vi "MAPPA MISURE.vi"(0 "Torsiometro":refnum<vi>, 1 "DATI NM":T29, 2 "Cluster INFO":T30={"Scelta wattmetro"={"Wattmetro"=enum."No Selection"}, "SET RPM"=0.0, "SET TEMP"=0.0, "Array banchi"=[{"Nome"="Elettropompa", "Tors. scala1"=0, "Tors. scala2"=0, "rpm"=0, "TAMB"=0, "Indici Temperature"=[0, 1], "Indice freno"=1, "alimentatore trifase"=0, "alimentatore monofase"=0, "alimentatore dc arm"=0, "alimentatore dc ecc"=0, "alimentatore dc mp"=0}, {"Nome"="Sommersa", "Tors. scala1"=0, "Tors. scala2"=0, "rpm"=0, "TAMB"=1, "Indici Temperature"=[0, 1], "Indice freno"=0, "alimentatore trifase"=0, "alimentatore monofase"=0, "alimentatore dc arm"=0, "alimentatore dc ecc"=0, "alimentatore dc mp"=0}], "Array valvole linee avvio/fermata"=[], "banco selezionato"=0, "Nomi valvole prop sistema"=[], "canale-- sensore"=[], "Attriti B1"=[], "Attriti B2"=[], "Collegamento elettrico"={"ALIMENTAZIONE ELETTRICA"=enum."AC TRIFASE", "ID"=0, "#rami freddo\\eq term resmeter"=0, "#rami riscaldamento resmeter"=0, "#rami freddo\\eq term resistomat"=0, "#rami riscaldamento resistomat"=0, "CALCOLI"=enum."AC TRIFASE"}, "lingua"=0, "Costanti collaudo"={"P [bar]"=0.0, "T amb. [°C]"=0.0, "Umidità [%]"=0.0, "T acqua [°C] 2"=0.0}, "OPZIONI MISURE RES"={"MISURA A FREDDO"=enum."RESISTOMAT", "MISURA EQ. TERMICO"=enum."RESISTOMAT", "MISURA DT PROVA IN CORSO"=enum."RESISTOMAT - CON FERMATE", "MISURE PRIMA E DOPO"=enum."RESISTOMAT", "STRUMENTI PRESENTI"=enum."NESSUNO"}, "Dati targa motore"={"Vnom"=0.0, "Fnom"=0.0, "Inom"=0.0, "Cnom"=0.0, "Npoli"=0.0, "Scorta 1"=0.0, "Scorta 2"=0.0, "Scorta 3"=0.0}}, 3 "MISURE ALL":T2={"Cluster READ NI"={"AI (0-10V)"={"AI 0"=0.0, "AI 1"=0.0, "AI 2"=0.0, "AI 3"=0.0, "AI 4"=0.0, "AI 5"=0.0, "AI 6"=0.0, "AI 7"=0.0, "AI 8"=0.0, "AI 9"=0.0, "AI 10"=0.0, "AI 11"=0.0, "AI 12"=0.0, "AI 13"=0.0, "AI 14"=0.0, "AI 15"=0.0, "AI 16"=0.0, "AI 17"=0.0, "AI 18"=0.0, "AI 19"=0.0, "AI 20"=0.0, "AI 21"=0.0, "AI 22"=0.0, "AI 23"=0.0, "AI 24"=0.0, "AI 25"=0.0, "AI 26"=0.0, "AI 27"=0.0, "AI 28"=0.0, "AI 29"=0.0, "AI 30"=0.0, "AI 31"=0.0}, "StatoAO_Cdaq[0-10V]"={"AO 1"=0.0, "AO 2"=0.0, "AO 3"=0.0, "AO 4"=0.0}, "Contatori [rpm]"={"RPM 1"=0.0, "RPM 2"=0.0}, "StatoAO_Cdaq [4-20mA]"={"Cdaq_AO [0-10V] 0 for Torque"=0.0, "Cdaq_AO [0-10V] 1"=0.0, "Cdaq_AO [0-10V] 2"=0.0, "Cdaq_AO [0-10V] 3"=0.0}, "StatoDO_Cdaq"={"Scorta 0"=FALSE, "Scorta 1"=FALSE, "Scorta 2"=FALSE, "Scorta 3"=FALSE, "Scorta 4"=FALSE, "Scorta 5"=FALSE, "Scorta 6"=FALSE, "Scorta 7"=FALSE, "Scorta 8"=FALSE, "Scorta 9"=FALSE, "Scorta 10"=FALSE, "Scorta 11"=FALSE, "Scorta 12"=FALSE, "Scorta 13"=FALSE, "Scorta 14"=FALSE, "Scorta 15"=FALSE, "Scorta 16"=FALSE, "Scorta 17"=FALSE, "Scorta 18"=FALSE, "Scorta 19"=FALSE, "Scorta 20"=FALSE, "Scorta 21"=FALSE, "Scorta 22"=FALSE, "Scorta 23"=FALSE, "Scorta 24"=FALSE, "Scorta 25"=FALSE, "Scorta 26"=FALSE, "Scorta 27"=FALSE, "Scorta 28"=FALSE, "Scorta 29"=FALSE, "Scorta 30"=FALSE, "Scorta 31"=FALSE}, "DI"={"Scorta 0"=FALSE, "Scorta 1"=FALSE, "Scorta 2"=FALSE, "Scorta 3"=FALSE, "Scorta 4"=FALSE, "Scorta 5"=FALSE, "Scorta 6"=FALSE, "Scorta 7"=FALSE, "Scorta 8"=FALSE, "Scorta 9"=FALSE, "Scorta 10"=FALSE, "Scorta 11"=FALSE, "Scorta 12"=FALSE, "Scorta 13"=FALSE, "Scorta 14"=FALSE, "Scorta 15"=FALSE, "Scorta 16"=FALSE, "Scorta 17"=FALSE, "Scorta 18"=FALSE, "Scorta 19"=FALSE, "Scorta 20"=FALSE, "Scorta 21"=FALSE, "Scorta 22"=FALSE, "Scorta 23"=FALSE, "Scorta 24"=FALSE, "Scorta 25"=FALSE, "Scorta 26"=FALSE, "Scorta 27"=FALSE, "Scorta 28"=FALSE, "Scorta 29"=FALSE, "Scorta 30"=FALSE, "Scorta 31"=FALSE}, "AI (4-20mA)"={"AI 0"=0.0, "AI 1"=0.0, "AI 2"=0.0, "AI 3"=0.0, "AI 4"=0.0, "AI 5"=0.0, "AI 6"=0.0, "AI 7"=0.0, "AI 8"=0.0, "AI 9"=0.0, "AI 10"=0.0, "AI 11"=0.0, "AI 12"=0.0, "AI 13"=0.0, "AI 14"=0.0, "AI 15"=0.0}, "TC [°C]"={"tc 1"=0.0, "tc 2"=0.0, "tc 3"=0.0, "tc 4"=0.0}, "NI Read Values"={"RPM"=0.0, "Frequency"=0.0, "Mod 1"={"Torsiometro 1"=0.0, "Torsiometro 2"=0.0, "Strin Gauge 1"=0.0, "Strin Gauge 2"=0.0}, "Mod 2"={"Termocoppia 1"=0.0, "Termocoppia 2"=0.0, "Termocoppia 3"=0.0, "Termocoppia 4"=0.0}, "Mod 3"={"PT 100 1"=0.0, "PT 100 2"=0.0, "PT 100 3"=0.0, "PT 100 4"=0.0}}}, "MISURE WT"={"URMS 1"=0.0, "IRMS 1"=0.0, "P 1"=0.0, "S 1"=0.0, "Q 1"=0.0, "LAMBDA 1"=0.0, "PHI 1"=0.0, "F U 1"=0.0, "F I 1"=0.0, "NONE 1"=0.0, "URMS 2"=0.0, "IRMS 2"=0.0, "P 2"=0.0, "S 2"=0.0, "Q 2"=0.0, "LAMBDA 2"=0.0, "PHI 2"=0.0, "F U 2"=0.0, "F I 2"=0.0, "NONE 2"=0.0, "URMS 3"=0.0, "IRMS 3"=0.0, "P 3"=0.0, "S 3"=0.0, "Q 3"=0.0, "LAMBDA 3"=0.0, "PHI 3"=0.0, "F U 3"=0.0, "F I 3"=0.0, "NONE 3"=0.0, "URMS SIGMA"=0.0, "IRMS SIGMA"=0.0, "P SIGMA"=0.0, "S SIGMA"=0.0, "Q SIGMA"=0.0, "LAMBDA SIGMA"=0.0, "PHI SIGMA"=0.0, "F U SIGMA"=0.0, "F I SIGMA"=0.0, "NONE 4"=0.0}, "Resistenze Resistomat"={"Res Ch1"=0.0, "Res Ch2"=0.0, "Res Ch3"=0.0, "Tamb"=0.0}, "INTERFACCIA"={"AI"={"Portate"=[], "Pressioni"=[], "Coppie[Nm]"=[], "Valvole prop %"=[], "RPM"=[], "Livelli"=[], "Temperature"=[], "Riferimenti %"=[], "TENSIONI"=[], "CORRENTI"=[]}, "DI (logici)"={"Start da pulsantiera"=FALSE, "Stop da pulsantiera"=FALSE, "Reset da pulsantiera"=FALSE, "Sistema OK"=FALSE, "Collaudo abilitato"=FALSE, "Potenza trifase abilitata"=FALSE, "Potenza monofase abilitata"=FALSE, "Potenza DC abilitata"=FALSE, "Potenza DC ECC abilitata"=FALSE, "Start alimentazione AC"=FALSE, "Start alimentazione DC"=FALSE, "Start DC eccitazione"=FALSE, "Teleruttore WT abilitato"=FALSE, "Teleruttore Resistomat abilitato"=FALSE, "Teleruttore corto fasi"=FALSE, "Ramo 1 resistomat"=FALSE, "Ramo 2 resistomat"=FALSE, "Ramo 3 resistomat"=FALSE, "B1 Scelta linea elettrica 1"=FALSE, "B1 Scelta linea elettrica 2"=FALSE, "B1 Scelta linea elettrica 3"=FALSE, "B1 Scelta linea elettrica 4"=FALSE, "B1 Scelta linea elettrica 5"=FALSE, "B2 Scelta linea elettrica 1"=FALSE, "B2 Scelta linea elettrica 2"=FALSE, "B2 Scelta linea elettrica 3"=FALSE, "B2 Scelta linea elettrica 4"=FALSE, "B2 Scelta linea elettrica 5"=FALSE, "Rotore bloccato 1"=FALSE, "Rotore bloccato 2"=FALSE, "FRENO 1 abilitato"=FALSE, "FRENO 1 run"=FALSE, "FRENO 1 senso rotaz"=FALSE, "FRENO 1 ctrl velocità"=FALSE, "FRENO 2 abilitato"=FALSE, "FRENO 2 run"=FALSE, "FRENO 2 senso rotaz"=FALSE, "FRENO 2 ctrl velocità"=FALSE, "ALIM 1 abilitato"=FALSE, "ALIM 1 run"=FALSE, "ALIM 2 abilitato"=FALSE, "ALIM 2 run"=FALSE, "ALIM 3 abilitato"=FALSE, "ALIM 3 run"=FALSE, "FRENO 1 ctrl coppia"=FALSE, "FRENO 2 ctrl coppia"=FALSE, "FRENO 3 ctrl coppia"=FALSE, "DI (logici) aggiuntivi impianto"={"Solo freno abilitato"=FALSE, "Carico resistivo abilitato"=FALSE, "AFE+freno abilitato"=FALSE, "Protezioni chiuse"=FALSE, "Start potenza AFE"=FALSE, "AFE in marcia"=FALSE}, "Misura corrente diretta WT"=FALSE, "Misura corrente sens ext"=FALSE, "Sens ext abilitati"=FALSE}, "AO non scalati"={"FRENO1 rif vel"=0.0, "FRENO1 rif Coppia"=0.0, "FRENO2 rif vel"=0.0, "FRENO2 rif Coppia"=0.0, "ALIM1 rif V"=0.0, "ALIM1 rif F"=0.0, "ALIM2 rif V"=0.0, "ALIM2 rif F"=0.0, "ALIM3 rif V"=0.0, "ALIM3 rif F"=0.0, "Fnom keb"=0.0, "Rpm nom keb"=0.0, "Pnom keb"=0.0, "Inom keb"=0.0, "Vnom keb"=0.0, "Rpm max keb"=0.0, "Tempo rampa keb"=0.0, "Tipo Mot keb"=0.0, "FRENO  rif Coppia "=0.0, "FRENO  rif  Corrente"=0.0}, "AO scalati"={"FRENO1 rif vel"=0.0, "FRENO1 rif Coppia"=0.0, "FRENO2 rif vel"=0.0, "FRENO2 rif Coppia"=0.0, "ALIM1 rif V"=0.0, "ALIM1 rif F"=0.0, "ALIM2 rif V"=0.0, "ALIM2 rif F"=0.0, "ALIM3 rif V"=0.0, "ALIM3 rif F"=0.0, "Fnom keb"=0.0, "Rpm nom keb"=0.0, "Pnom keb"=0.0, "Inom keb"=0.0, "Vnom keb"=0.0, "Rpm max keb"=0.0, "Tempo rampa keb"=0.0, "Tipo Mot keb"=0.0, "FRENO  rif Coppia "=0.0, "FRENO  rif  Corrente"=0.0}, "DO (logici)"={"Scelta banco 1"=FALSE, "Scelta banco 2"=FALSE, "Scelta banco 3"=FALSE, "FRENO 1 abilita"=FALSE, "FRENO 1 start"=FALSE, "FRENO 1 senso rotaz"=FALSE, "FRENO 1 ctrl velocità"=FALSE, "FRENO 2 abilita"=FALSE, "FRENO 2 start"=FALSE, "FRENO 2 senso rotaz"=FALSE, "FRENO 2 ctrl velocità"=FALSE, "ALIM 1 abilita"=FALSE, "ALIM 1 start"=FALSE, "ALIM 2 abilita"=FALSE, "ALIM 2 start"=FALSE, "ALIM 3 abilita"=FALSE, "ALIM 3 start"=FALSE, "Abilita linea trifase"=FALSE, "Abilita linea monofase"=FALSE, "Abilita linea dc"=FALSE, "Abilita linea dc eccit"=FALSE, "B1 Linea elettrica 1"=FALSE, "B1 Linea elettrica 2"=FALSE, "B1 Linea elettrica 3"=FALSE, "B1 Linea elettrica 4"=FALSE, "B1 Linea elettrica 5"=FALSE, "B2 Linea elettrica 1"=FALSE, "B2 Linea elettrica 2"=FALSE, "B2 Linea elettrica 3"=FALSE, "B2 Linea elettrica 4"=FALSE, "B2 Linea elettrica 5"=FALSE, "Start potenza AC"=FALSE, "Stop pontenza AC"=FALSE, "Start potenza DC"=FALSE, "Stop potenza DC"=FALSE, "Start potenza eccitaz"=FALSE, "Stop potenza eccitaz"=FALSE, "Reset allarmi"=FALSE, "watchdog"=FALSE, "Scala torsiometro B1"=FALSE, "Controllo torsiom B1"=FALSE, "Scala torsiometro B2"=FALSE, "Controllo torsiom B2"=FALSE, "Teleruttore WT abilita"=FALSE, "Teleruttore Resistomat abilita"=FALSE, "Teleruttore corto fasi"=FALSE, "Ramo 1 resistomat"=FALSE, "Ramo 2 resistomat"=FALSE, "Ramo 3 resistomat"=FALSE, "Collaudo in corso"=FALSE, "Allarme presente"=FALSE, "Enable Res Meter"=FALSE, "Bypass Res Meter"=FALSE, "2nd canale Res Meter"=FALSE, "Scala 200/2000 res meter"=FALSE, "Taratura res meter"=FALSE, "FRENO 1 ctrl coppia"=FALSE, "FRENO 2 ctrl coppia"=FALSE, "FRENO 3 ctrl coppia"=FALSE, "Aggiuntivi impianto"={"Senso rotazione alim 1"=FALSE, "Senso rotazione alim 2"=FALSE}, "ALIM 1 stop"=FALSE, "ALIM 2 stop"=FALSE, "ALIM 3 stop"=FALSE, "FRENO 1 stop"=FALSE, "FRENO 2 stop"=FALSE, "FRENO 3 stop"=FALSE, "B1 configurazione freno B"=FALSE, "B2 configurazione freno B"=FALSE, "Abilita scrittura KEB"=FALSE, "Bench Selection (0-B1,1-B2)"=FALSE, "Select current mode"=FALSE, "Select torque mode"=FALSE, "Select speed mode"=FALSE, "Start"=FALSE, "Stop"=FALSE, "Block"=FALSE, "Enable Force mode"=FALSE, "Abilita linea 125 A"=FALSE, "Abilita linea 63 A"=FALSE, "Abilita linea 16 A"=FALSE, "Aum Tensione Variac"=FALSE, "Dim Tesnione Variac"=FALSE, "Abilita ellectro stractura"=FALSE, "Risprinito Emergence"=FALSE, "Abilita collaudo"=FALSE, "Disabilita collaudo"=FALSE, "External Alaram"=FALSE, "Enable external program"=FALSE, "Reset"=FALSE, "Abilita Ingresso Variac"=FALSE, "Abilita Ventilatore Variac"=FALSE, "Abilita Uscita Variac "=FALSE}}, "FREDDO resistomat"={"Res Ch1"=0.0, "Res Ch2"=0.0, "tAMB"=0.0, "Res Ch3"=0.0}, "STATO PLC 1"={"USCITE PLC"={"AO (real) 2"={"SCORTA 1"=0.0, "SCORTA 2"=0.0, "SCORTA 3"=0.0, "SCORTA 4"=0.0, "SCORTA 5"=0.0, "SCORTA 6"=0.0, "SCORTA 7"=0.0, "SCORTA 8"=0.0}, "statoAO_PLC out"={"Rif Lim coppia freno [%]"=nan, "Rif rpm freno [%]"=nan, "Rif coppia freno [%]"=0.0, "Rif V alimentatore [%]"=0.0, "Rif F alimentatore [%]"=0.0}, "DO (bit)"={"Scelta banco 1"=FALSE, "Set dati motore freno 2"=FALSE, "Diretto inverter"=FALSE, "Filtro LC"=FALSE, "Marcia ALIM (1s)"=FALSE, "Marcia FRENO (1s)"=FALSE, "Stop AFE (1s)"=FALSE, "Stop freno (1s)"=FALSE, "Reset allarmi"=FALSE, "Watchdog"=FALSE, "Senso rotazione"=FALSE, "Abilita collaudo (1s)"=FALSE, "Disabilita collaudo (1s)"=FALSE, "Abilitazione ALIM"=FALSE, "Abilitazione FRENO"=FALSE, "Teleruttore WT"=FALSE, "Senso rot motore prova"=FALSE, "Scorta 7"=FALSE, "Scorta 8"=FALSE, "Scorta 9"=FALSE, "Scorta 10"=FALSE, "Scorta 11"=FALSE, "Scorta 12"=FALSE, "Scorta 13"=FALSE}}, "Stato DI_PLC"={"Sistema OK"=FALSE, "Rotore bloccato"=FALSE, "Scorta 1"=FALSE, "Prova diretto inverter"=FALSE, "Prova con filtro LC"=FALSE, "Teleruttore WT abilitato"=FALSE, "Alim sinus penta abilitato"=FALSE, "Alim sinus penta in marcia"=FALSE, "Freno abilitato"=FALSE, "Freno in marcia"=FALSE, "Senso rotazione freno"=FALSE, "Potenza abilitata"=FALSE, "Scorta 3"=FALSE, "Scorta 4"=FALSE, "scorta 5"=FALSE, "scorta 6"=FALSE}, "AI plc"={"Allarmi 1"=0.0, "Allarmi 2"=0.0, "Scorta 1"=0.0, "Scorta 2"=0.0, "RPM mot prova"=0.0, "I mot prova"=0.0, "RPM freno"=0.0, "I freno"=0.0, "Scorta 3"=0.0, "Scorta 4"=0.0}}, "Res Ch2"=0.0, "Res Ch2 2"=0.0, "FREDDO res meter"={"Res Ch1"=0.0, "Res Ch2"=0.0, "tAMB"=0.0, "Res Ch3"=0.0}, "Resistenze Res Meter"={"Res Ch1"=0.0, "Res Ch2"=0.0, "Res Ch3"=0.0, "Tamb"=0.0}, "READ SINUS PENTA"={"Menù Misure motore (M000-M030)"={"Rif vel a regime (int)"=0, "Rif vel a regime (dec)"=0, "Rif vel dopo rampe (int)"=0, "Rif vel dopo rampe (dec)"=0, "RPM motore (int)"=0, "RPM motore (dec)"=0, "FREQout inverter"=0, "Rif coppia a regime(Nm)"=0, "Richiesta di coppia (Nm)"=0, "Coppia generata dal motore(Nm)"=0, "Rif coppia a regime(%)"=0, "Richiesta di coppia (%)"=0, "Coppia generata dal motore(%)"=0, "Coppia max richiesta prima delle rampe(Nm)"=0, "Coppia max richiesta dopo le rampe(Nm)"=0, "Limite di velocità prima delle rampe"=0, "Limite di velocità dopo le rampe"=0, "Coppia max richiesta prima delle rampe(%)"=0, "Coppia max richiesta dopo le rampe(%)"=0, "Rif di flusso"=0, "Corrente di uscita"=0, "Capacità termica del motore"=0, "Tensione di uscita"=0, "Potenza di uscita"=0, "Energia consumata (LSword)"=0, "Energia consumata (MSword)"=0, "Tensione bus DC"=0, "Tensione di rete"=0}, "Menù regolatore PID (M018-M024)"={"Rif PID a regime(%)"=0, "Rif pid dopo rampe(%)"=0, "Retroazione del pid(%)"=0, "Errore del pid(%)"=0, "uscita del pid(%)"=0, "Rif del pid dopo le rampe"=0, "Retroazione del pid"=0}, "Menù ingressi digitali (M031-M036)"={"Ingressi digitali ritardati"=0, "Ingressi digitali istantanei"=0, "Moresettiera comando loc"=0, "Morsett comando da seriale"=0, "Morsett comando bus di campo"=0, "Ing dig ausiliari da morsettiera"=0, "Ing dig ausiliari da seriale"=0}, "Menù riferimenti (M037-M051)"={"Rif analog est REF"=0, "Rif analog est AIN1"=0, "Rif analog est AIN2"=0, "Rif analog est XAIN4"=0, "Rif analog est XAIN5"=0, "Rif velocità da seriale(int)"=0, "Rif velocità bus di campo(int)"=0, "Rif coppia da seriale"=0, "Rif coppia bus di campo"=0, "Rif del PID da seriale"=0, "Rif del PID da bus di campo"=0, "Retroazione del PID da seriale"=0, "Retroazione del PIDda bus di campo"=0, "Rif da encoder"=0, "Rif in frequenza"=0, "Rif velocità da seriale(dec)"=0, "Rif velocità bus di campo(dec)"=0}, "Menù rampe (P009-P033)"={"Tempo di dec rampa di vel 1"=0, "Tempo di acc rampa di vel 2"=0, "Tempo di dec rampa di vel 2"=0, "Tempo di acc rampa di vel 1"=0, "Unità di mis tempi rampe vel 1/2"=0, "Tempo di acc rampa di vel 3"=0, "Tempo di dec rampa di vel 3"=0, "Tempo di acc rampa di vel 4"=0, "Tempo di dec rampa di vel 4"=0, "Unità di mis tempi rampe vel 3/4"=0, "Selettore arrottondam rampe"=0, "Tempo di arrotond iniz rampa acc"=0, "Tempo di arrotond finale rampa acc"=0, "Tempo di arrotond iniz rampa dec"=0, "Tempo di rampa di salita rif coppia"=0, "Tempo di rampa di discesa rif coppia"=0, "Unità di misura rampa coppia"=0, "Tempo rampa acc marcia jog"=0, "Tempo rampa dec marcia jog"=0, "Reset acc ai cambi pendenza"=0, "rampa di acc in fire mode"=0, "rampa di dec in fire mode"=0, "Tempo di arrotond finale rampa dec"=0}, "Menù controllo motore(C008-C128)"={"Numero motori configurati"=0, "Tipo algoritmo di controllo Mot1"=0, "Tipo rif Mot1"=0, "Tensione nominale rete"=0, "Retroaz di vel da encoder Mot1"=0, "Tipo curva V/f Mot1"=0, "Rotazione delle fasi Mot1"=0, "Freq nominale del motore Mot1"=0, "RPM nominali del motore Mot1"=0, "Potenza nominale del motore Mot1"=0, "Corrente nominale del motore Mot1"=0, "Tensione nominale del motore mot1"=0, "Potenza a vuoto del motore Mot1"=0, "Corrente a vuoto del motore Mot1"=0, "Resistenza statorica del motore Mot1"=0, "Induttanza di dispersione Mot1"=0, "Induttanza mutua motore"=0, "Costante di tempo rotorica"=0, "Costante di tempo filtro pb"=0, "Velocità minima motore"=0, "Velocità massima motore"=0}, "Menù configurazione PID"={"Selezione riferimento n.1"=0, "Selezione retroazione n.1"=0, "Modalità di fuzionamento PID"=0, "Termine derivativo calcolato su err o mis"=0, "Proporz moltiplica deriv e integrale"=0, "Azione del PID"=0}, "ID"=0.0, "Menù uscite digitali"={"MDO4 Inverter pronto"=0}, "Fcarrier"={"Fcarrier Min (Hz)"=0, "Fcarrier Max (Hz)"=0}, "stato inverter M089"=0.0, "Riferimenti"={"Rif tensione"=0, "Rif velocità"=0}, "Comunicazione"=FALSE, "Modalità stop"=0.0}, "STATO PLC 2"={"USCITE PLC"={"AO (real) 2"={"SCORTA 1"=0.0, "SCORTA 2"=0.0, "SCORTA 3"=0.0, "SCORTA 4"=0.0, "SCORTA 5"=0.0, "SCORTA 6"=0.0, "SCORTA 7"=0.0, "SCORTA 8"=0.0}, "statoAO_PLC out"={"Condensatori"=0.0, "Scorta 1"=0.0, "Scorta 2"=0.0}, "DO (bit)"={"Relè misura resistomat"=FALSE, "Misura res ramo 1"=FALSE, "Misura res ramo 2"=FALSE, "Misura res ramo 3"=FALSE, "Scelta banco 2"=FALSE, "Scala Torsiometro"=FALSE, "Ctrl torsiometro"=FALSE, "Select current mode"=FALSE, "Select Torque mode"=FALSE, "Select speed mode"=FALSE, "Watchdog"=FALSE, "Scorta"=FALSE, "Scorta 2"=FALSE, "Scorta 3"=FALSE, "Scorta 4"=FALSE, "Scorta 5"=FALSE, "Bench selection"=FALSE, "External alarm"=FALSE, "Enable external program"=FALSE, "Reset allarmi"=FALSE, "Start"=FALSE, "Stop"=FALSE, "Block"=FALSE, "Scorta 6"=FALSE}}, "Stato DI_PLC"={"Sistema ok"=FALSE, "Relè Resistomat abilitato"=FALSE, "Freno abilitato"=FALSE, "Freno in marcia"=FALSE, "scorta b"=FALSE, "scorta a"=FALSE, "scorta 1"=FALSE, "scorta 2"=FALSE, "scorta 3"=FALSE, "scorta 4"=FALSE, "Scorta 5"=FALSE, "Scorta 6"=FALSE, "Scorta 7"=FALSE, "Scorta 8"=FALSE, "Scorta 9"=FALSE, "Scorta 10"=FALSE}, "AI plc"={"Allarmi 1"=0.0, "Allarmi 2"=0.0, "TC 1"=0.0, "TC 2"=0.0, "TC 3"=0.0, "TC 4"=0.0, "TC 5"=0.0, "TC 6"=0.0, "TC 7"=0.0, "TC 8"=0.0, "PT1000 1"=0.0, "PT1000 2"=0.0, "PT1000 3"=0.0, "PT1000 4"=0.0}}, "STATO PLC 3"={"USCITE PLC"={"AO (real) 2"={"SCORTA 1"=0.0, "SCORTA 2"=0.0, "SCORTA 3"=0.0, "SCORTA 4"=0.0, "SCORTA 5"=0.0, "SCORTA 6"=0.0, "SCORTA 7"=0.0, "SCORTA 8"=0.0}, "statoAO_PLC out"={"Rif velocità alimentatore"=0.0, "Scorta"=0.0, "Tipo Motore  keb"=0.0, "I nom keb"=0.0, "RPM nom keb"=0.0, "V nom keb"=0.0, "F nom keb"=0.0, "t rampa keb"=0.0}, "DO (bit)"={"Select linea Inverter"=FALSE, "Abilita sense wattmetro"=FALSE, "Bypass filtro LC"=FALSE, "Filtro LC"=FALSE, "Bypass trasformatore"=FALSE, "Trasformatore"=FALSE, "Abilita uscite variac"=FALSE, "Abilita linea 125 A"=FALSE, "Abilita linea 63 A"=FALSE, "Abilita linea 16 A"=FALSE, "Abilita Scrittura Dati Keb"=FALSE, "Abilita alimentatore"=FALSE, "Marcia alimentatore (1s)"=FALSE, "Stop alimentatore (1s)"=FALSE, "Senso rot mot prova"=FALSE, "Watchdog"=FALSE, "Aumenta tensione variac"=FALSE, "Diminuisci tensione variac "=FALSE, "Blocco elettroserrature"=FALSE, "Ripristino emergence"=FALSE, "Abilita ingresso variac"=FALSE, "Abilita ventilatore variac"=FALSE, "Reset Allarm"=FALSE, "Scorta 1"=FALSE, "Scorta 2"=FALSE, "Scorta 3"=FALSE, "Scorta 4"=FALSE, "Scorta 5"=FALSE, "Scorta 6"=FALSE, "Scorta 7"=FALSE, "Scorta 8"=FALSE, "Scorta 9"=FALSE, "Abilita collaudo"=FALSE, "Disabilita collaudo "=FALSE, "Scorta 10"=FALSE, "Scorta 11"=FALSE, "Scorta 12"=FALSE, "Scorta 13"=FALSE, "Scorta 14"=FALSE, "Scorta 15"=FALSE}}, "Stato DI_PLC"={"Sistema OK"=FALSE, "Rotore bloccato"=FALSE, "Filtro LC"=FALSE, "Bypass Filtro LC"=FALSE, "Scelta Trasformatore"=FALSE, "Scelta Bypass trasformatore"=FALSE, "Teleruttore wt abilitato"=FALSE, "Alimentatore abilitato"=FALSE, "Alimentatore in marcia"=FALSE, "Scorta 1"=FALSE, "Scorta 2"=FALSE, "Scorta 3"=FALSE, "Potenza abilitata"=FALSE, "Alimentatore in allarme"=FALSE, "Scorta 4"=FALSE, "Conferma dati KEB"=FALSE, "Scorta 5"=FALSE, "Warning Inverter Alimentatore"=FALSE, "Variac Abilitato"=FALSE, "Linea 125 A abilitata"=FALSE, "Linea 63 A abilitata"=FALSE, "Linea 16 A abilitata"=FALSE, "Scorta 6"=FALSE, "Enable force mode"=FALSE}, "AI plc"={"Allarmi 1"=0.0, "Allarmi 2"=0.0, "RPM motore prova"=0.0, "Corrente motore prova"=0.0, "RPM freno"=0.0, "Corrente freno"=0.0, "Tipo motore keb"=0.0, "I nom keb"=0.0, "RPM nom keb"=0.0, "V nom keb"=0.0, "F nom keb"=0.0, "T rampa keb"=0.0, "scorta"=0.0, "Scorta 2"=0.0}}, "DCREG"={"Parametri di misura"={"M000"=0.0, "M001"=0.0, "M002"=0.0, "M003"=0.0, "M004"=0.0, "M005"=0.0, "M006"=0.0, "M007"=0.0, "M008"=0.0, "M009"=0.0, "M010"=0.0, "M011"=0.0, "M012"=0.0, "M013"=0.0, "M014"=0.0, "M015"=0.0, "M016"=0.0, "M017"=0.0, "M018"=0.0, "M019"=0.0, "M020"=0.0, "M021"=0.0, "M022"=0.0, "M023"=0.0, "M024"=0.0, "M025"=0.0, "M026"=0.0, "M027"=0.0, "M028"=0.0, "M029"=0.0, "M030"=0.0, "M031"=0.0}, "Parametri di programmazione"={"P000"=0.0, "P001"=0.0, "P002"=0.0, "P003"=0.0, "P004"=0.0, "P005"=0.0, "P006"=0.0, "P010"=0.0, "P011"=0.0, "P012"=0.0, "P013"=0.0, "P014"=0.0, "P015"=0.0, "P016"=0.0, "P030"=0.0, "P031"=0.0, "P032"=0.0, "P033"=0.0, "P034"=0.0, "P035"=0.0, "P036"=0.0, "P037"=0.0, "P038"=0.0, "P039"=0.0, "P040"=0.0, "P050"=0.0, "P051"=0.0, "P052"=0.0, "P053"=0.0, "P054"=0.0, "P055"=0.0, "P056"=0.0, "P057"=0.0, "P058"=0.0, "P059"=0.0, "P060"=0.0, "P061"=0.0, "P062"=0.0, "P070"=0.0, "P071"=0.0, "P073"=0.0, "P074"=0.0, "P076"=0.0, "P077"=0.0, "P079"=0.0, "P080"=0.0, "P082"=0.0, "P083"=0.0, "P084"=0.0, "P085"=0.0, "P086"=0.0, "P087"=0.0, "P088"=0.0, "P100"=0.0, "P101"=0.0, "P102"=0.0, "P103"=0.0, "P104"=0.0, "P110"=0.0, "P111"=0.0, "P120"=0.0, "P121"=0.0, "P122"=0.0, "P123"=0.0, "P124"=0.0, "P125"=0.0, "P126"=0.0, "P127"=0.0, "P128"=0.0, "P129"=0.0, "P130"=0.0, "P131"=0.0, "P132"=0.0, "P133"=0.0, "P134"=0.0, "P150"=0.0, "P151"=0.0, "P152"=0.0, "P153"=0.0, "P154"=0.0, "P155"=0.0, "P156"=0.0, "P157"=0.0, "P158"=0.0, "P170"=0.0, "P171"=0.0, "P172"=0.0, "P173"=0.0, "P174"=0.0, "P175"=0.0, "P176"=0.0, "P177"=0.0, "P178"=0.0, "P179"=0.0, "P180"=0.0, "P181"=0.0, "P182"=0.0, "P183"=0.0, "P184"=0.0, "P185"=0.0, "P186"=0.0, "P187"=0.0, "P188"=0.0, "P189"=0.0, "P190"=0.0, "P191"=0.0, "P192"=0.0, "P193"=0.0, "P194"=0.0, "P195"=0.0, "P196"=0.0, "P197"=0.0, "P198"=0.0, "P199"=0.0, "P211"=0.0, "P212"=0.0, "P213"=0.0, "P214"=0.0, "P215"=0.0, "P216"=0.0, "P217"=0.0, "P221"=0.0, "P222"=0.0, "P223"=0.0, "P224"=0.0, "P230"=0.0, "P231"=0.0, "P240"=0.0, "P250"=0.0, "P251"=0.0}, "Parametri di configurazione"={"C000"=0.0, "C001"=0.0, "C002"=0.0, "C010"=0.0, "C011"=0.0, "C012"=0.0, "C014"=0.0, "C015"=0.0, "C016"=0.0, "C017"=0.0, "C018"=0.0, "C030"=0.0, "C050"=0.0, "C051"=0.0, "C052"=0.0, "C060"=0.0, "C061"=0.0, "C062"=0.0, "C063"=0.0, "C070"=0.0, "C072"=0.0, "C074"=0.0, "C090"=0.0, "C091"=0.0, "C092"=0.0, "C093"=0.0, "C094"=0.0, "C100"=0.0, "C101"=0.0, "C102"=0.0, "C103"=0.0, "C105"=0.0, "C106"=0.0, "C107"=0.0, "C108"=0.0, "C110"=0.0, "C111"=0.0, "C112"=0.0, "C120"=0.0, "C121"=0.0, "C122"=0.0, "C130"=0.0, "C131"=0.0, "C132"=0.0, "C133"=0.0, "C134"=0.0, "C135"=0.0, "C141"=0.0, "C142"=0.0, "C143"=0.0, "C150"=0.0, "C151"=0.0, "C153"=0.0, "C154"=0.0, "C155"=0.0, "C156"=0.0, "C157"=0.0, "C158"=0.0, "C159"=0.0, "C160"=0.0, "C161"=0.0, "C162"=0.0, "C163"=0.0, "C164"=0.0, "C165"=0.0, "C170"=0.0}, "Codice allarme"=0.0, "Comunicazione"=FALSE}} {"Cluster READ NI"."AI (4-20mA)"."AI 15" format="%#_6f"; "Cluster READ NI"."AI (4-20mA)"."AI 14" format="%#_6f"; "Cluster READ NI"."AI (4-20mA)"."AI 13" format="%#_6f"; "Cluster READ NI"."AI (4-20mA)"."AI 11" format="%#_6f"; "Cluster READ NI"."AI (4-20mA)"."AI 10" format="%#_6f"; "Cluster READ NI"."AI (4-20mA)"."AI 9" format="%#_6f"; "Cluster READ NI"."AI (4-20mA)"."AI 4" format="%#_6f"; "Cluster READ NI"."AI (4-20mA)"."AI 12" format="%#_6f"; "Cluster READ NI"."AI (4-20mA)"."AI 0" format="%#_6f"; "Cluster READ NI"."AI (4-20mA)"."AI 1" format="%#_6f"; "Cluster READ NI"."AI (4-20mA)"."AI 2" format="%#_6f"; "Cluster READ NI"."AI (4-20mA)"."AI 3" format="%#_6f"; "Cluster READ NI"."AI (4-20mA)"."AI 5" format="%#_6f"; "Cluster READ NI"."AI (4-20mA)"."AI 6" format="%#_6f"; "Cluster READ NI"."AI (4-20mA)"."AI 7" format="%#_6f"; "Cluster READ NI"."AI (4-20mA)"."AI 8" format="%#_6f"; "Cluster READ NI"."AI (0-10V)"."AI 31" format="%#_6f"; "Cluster READ NI"."AI (0-10V)"."AI 30" format="%#_6f"; "Cluster READ NI"."AI (0-10V)"."AI 29" format="%#_6f"; "Cluster READ NI"."AI (0-10V)"."AI 28" format="%#_6f"; "Cluster READ NI"."AI (0-10V)"."AI 27" format="%#_6f"; "Cluster READ NI"."AI (0-10V)"."AI 26" format="%#_6f"; "Cluster READ NI"."AI (0-10V)"."AI 25" format="%#_6f"; "Cluster READ NI"."AI (0-10V)"."AI 24" format="%#_6f"; "Cluster READ NI"."AI (0-10V)"."AI 23" format="%#_6f"; "Cluster READ NI"."AI (0-10V)"."AI 22" format="%#_6f"; "Cluster READ NI"."AI (0-10V)"."AI 21" format="%#_6f"; "Cluster READ NI"."AI (0-10V)"."AI 20" format="%#_6f"; "Cluster READ NI"."AI (0-10V)"."AI 19" format="%#_6f"; "Cluster READ NI"."AI (0-10V)"."AI 18" format="%#_6f"; "Cluster READ NI"."AI (0-10V)"."AI 17" format="%#_6f"; "Cluster READ NI"."AI (0-10V)"."AI 16" format="%#_6f"; "Cluster READ NI"."AI (0-10V)"."AI 15" format="%#_6f"; "Cluster READ NI"."AI (0-10V)"."AI 14" format="%#_6f"; "Cluster READ NI"."AI (0-10V)"."AI 13" format="%#_6f"; "Cluster READ NI"."AI (0-10V)"."AI 11" format="%#_6f"; "Cluster READ NI"."AI (0-10V)"."AI 10" format="%#_6f"; "Cluster READ NI"."AI (0-10V)"."AI 9" format="%#_6f"; "Cluster READ NI"."AI (0-10V)"."AI 4" format="%#_6f"; "Cluster READ NI"."AI (0-10V)"."AI 12" format="%#_6f"; "Cluster READ NI"."AI (0-10V)"."AI 0" format="%#_6f"; "Cluster READ NI"."AI (0-10V)"."AI 1" format="%#_6f"; "Cluster READ NI"."AI (0-10V)"."AI 2" format="%#_6f"; "Cluster READ NI"."AI (0-10V)"."AI 3" format="%#_6f"; "Cluster READ NI"."AI (0-10V)"."AI 5" format="%#_6f"; "Cluster READ NI"."AI (0-10V)"."AI 6" format="%#_6f"; "Cluster READ NI"."AI (0-10V)"."AI 7" format="%#_6f"; "Cluster READ NI"."AI (0-10V)"."AI 8" format="%#_6f"}, 4 "ACQ RESISTOMAT?":bool=TRUE, 6 "SIMULAZIONE":bool) -> (14 "Cluster MISURE":T27={"MISURE NM"={"Banco"="", "Anno"="", "Numero"="", "Ntabella"="", "Misura"="", "Tipo Prova"="", "ProgressivoAcq"="", "Descrizione"="", "Data_ora"="", "t. acq [h:m:s]"="", "t. acq [min]"="", "t. acq [s]"="", "n [rpm]"="", "f [Hz]"="", "U1[V]"="", "U2 [V]"="", "U3 [V]"="", "U123_media [V]"="", "I1[A]"="", "I2[A]"="", "I3[A]"="", "I123_media [A]*I"="", "I_123_sbil [%]"="", "Ulin[V]"="", "Uc [V]"="", "Uaux [V]"="", "Ilin[A]*I"="", "Imar[A]"="", "Iaux[A]"="", "Uarm[V]"="", "Uecc[V]"="", "Iarm[A]*I"="", "Iecc[A]"="", "pf"="", "P1 [W]"="", "P1 [kW]"="", "Q [VAR]"="", "Q [kVAR]"="", "S [VA]"="", "S [kVA]"="", "P1arm[W]"="", "P1ecc[W]"="", "Parm[kW]"="", "P1ecc[kW]"="", "Cond[uF]"="", "P1_linea_6fili[W]"="", "P1_linea_6fili[kW]"="", "eta_gr_6fili [%]"="", "eta_inverter_6fili [%]"="", "pf_linea_6fili"="", "U4 [V]"="", "U5 [V]"="", "U6 [V]"="", "U456_media [V]"="", "I4 [A]"="", "I5 [A]"="", "I6 [A]"="", "I456_media [A]"="", "C [Nm]*C"="", "Cric [Nm]"="", "Cric\\Cnom"="", "Iric[A]"="", "Iric\\Inom"="", "P2_mecc [W]"="", "P2_mecc [kW]"="", "eta motore [%]"="", "Scorr[%]"="", "Tamb[°C]"="", "R1[ohm]"="", "R2[ohm]"="", "R3[ohm]"="", "Rmedia[ohm]"="", "DT_R1[°C]"="", "DT_R2[°C]"="", "DT_R3[°C]"="", "DT_media[°C]"="", "R_marcia[ohm]"="", "R_aux[ohm]"="", "DT_marcia[°C]"="", "DT_aux[°C]"="", "R_Arm[ohm]"="", "R_Ecc[ohm]"="", "DT_Arm[°C]"="", "DT_Ecc[°C]"="", "TambFreddo[°C]"="", "R1_freddo[ohm]"="", "R2_freddo[ohm]"="", "R3_freddo[ohm]"="", "Rmedia_freddo[ohm]"="", "R_Marcia_freddo[ohm]"="", "R_Aux_freddo[ohm]"="", "R_Arm_freddo[ohm]"="", "R_Ecc_freddo[ohm]"="", "TC1 [°C]"="", "TC2 [°C]"="", "TC3 [°C]"="", "TC4 [°C]"="", "TC5 [°C]"="", "TC6 [°C]"="", "TC7 [°C]"="", "TC8 [°C]"="", "PT1000_1[°C]"="", "PT1000_2[°C]"="", "PT1000_3[°C]"="", "Vdc eccitatrice[V]"="", "Idc eccitatrice[A]"="", "Vdc rotore[V]"="", "Idc rotore[A]"="", "Vac rotore[V]"="", "Iac rotore[V]"="", "V dinamo[V]"="", "Portata Q"="", "Pressione H"="", "U1'[V]"="", "U2'[V]"="", "U3'[V]"="", "I1'[A]"="", "I2'[A]"="", "I3'[A]"="", "U''R-N"="", "U''S-N"="", "U'' T-N"="", "U''R-S"="", "U''R-T"="", "U''S-T"="", "I1''[A]"="", "I2''[A]"="", "I3''[A]"="", "F''[Hz]"="", "P''[kW]"="", "CosFi''"="", "PT1000_4[°C]"="", "Scorta 3"=""}, "MISURE ALL"={"Cluster READ NI"={"AI (0-10V)"={"AI 0"=0.0, "AI 1"=0.0, "AI 2"=0.0, "AI 3"=0.0, "AI 4"=0.0, "AI 5"=0.0, "AI 6"=0.0, "AI 7"=0.0, "AI 8"=0.0, "AI 9"=0.0, "AI 10"=0.0, "AI 11"=0.0, "AI 12"=0.0, "AI 13"=0.0, "AI 14"=0.0, "AI 15"=0.0, "AI 16"=0.0, "AI 17"=0.0, "AI 18"=0.0, "AI 19"=0.0, "AI 20"=0.0, "AI 21"=0.0, "AI 22"=0.0, "AI 23"=0.0, "AI 24"=0.0, "AI 25"=0.0, "AI 26"=0.0, "AI 27"=0.0, "AI 28"=0.0, "AI 29"=0.0, "AI 30"=0.0, "AI 31"=0.0}, "StatoAO_Cdaq[0-10V]"={"AO 1"=0.0, "AO 2"=0.0, "AO 3"=0.0, "AO 4"=0.0}, "Contatori [rpm]"={"RPM 1"=0.0, "RPM 2"=0.0}, "StatoAO_Cdaq [4-20mA]"={"Cdaq_AO [0-10V] 0 for Torque"=0.0, "Cdaq_AO [0-10V] 1"=0.0, "Cdaq_AO [0-10V] 2"=0.0, "Cdaq_AO [0-10V] 3"=0.0}, "StatoDO_Cdaq"={"Scorta 0"=FALSE, "Scorta 1"=FALSE, "Scorta 2"=FALSE, "Scorta 3"=FALSE, "Scorta 4"=FALSE, "Scorta 5"=FALSE, "Scorta 6"=FALSE, "Scorta 7"=FALSE, "Scorta 8"=FALSE, "Scorta 9"=FALSE, "Scorta 10"=FALSE, "Scorta 11"=FALSE, "Scorta 12"=FALSE, "Scorta 13"=FALSE, "Scorta 14"=FALSE, "Scorta 15"=FALSE, "Scorta 16"=FALSE, "Scorta 17"=FALSE, "Scorta 18"=FALSE, "Scorta 19"=FALSE, "Scorta 20"=FALSE, "Scorta 21"=FALSE, "Scorta 22"=FALSE, "Scorta 23"=FALSE, "Scorta 24"=FALSE, "Scorta 25"=FALSE, "Scorta 26"=FALSE, "Scorta 27"=FALSE, "Scorta 28"=FALSE, "Scorta 29"=FALSE, "Scorta 30"=FALSE, "Scorta 31"=FALSE}, "DI"={"Scorta 0"=FALSE, "Scorta 1"=FALSE, "Scorta 2"=FALSE, "Scorta 3"=FALSE, "Scorta 4"=FALSE, "Scorta 5"=FALSE, "Scorta 6"=FALSE, "Scorta 7"=FALSE, "Scorta 8"=FALSE, "Scorta 9"=FALSE, "Scorta 10"=FALSE, "Scorta 11"=FALSE, "Scorta 12"=FALSE, "Scorta 13"=FALSE, "Scorta 14"=FALSE, "Scorta 15"=FALSE, "Scorta 16"=FALSE, "Scorta 17"=FALSE, "Scorta 18"=FALSE, "Scorta 19"=FALSE, "Scorta 20"=FALSE, "Scorta 21"=FALSE, "Scorta 22"=FALSE, "Scorta 23"=FALSE, "Scorta 24"=FALSE, "Scorta 25"=FALSE, "Scorta 26"=FALSE, "Scorta 27"=FALSE, "Scorta 28"=FALSE, "Scorta 29"=FALSE, "Scorta 30"=FALSE, "Scorta 31"=FALSE}, "AI (4-20mA)"={"AI 0"=0.0, "AI 1"=0.0, "AI 2"=0.0, "AI 3"=0.0, "AI 4"=0.0, "AI 5"=0.0, "AI 6"=0.0, "AI 7"=0.0, "AI 8"=0.0, "AI 9"=0.0, "AI 10"=0.0, "AI 11"=0.0, "AI 12"=0.0, "AI 13"=0.0, "AI 14"=0.0, "AI 15"=0.0}, "TC [°C]"={"tc 1"=0.0, "tc 2"=0.0, "tc 3"=0.0, "tc 4"=0.0}, "NI Read Values"={"RPM"=0.0, "Frequency"=0.0, "Mod 1"={"Torsiometro 1"=0.0, "Torsiometro 2"=0.0, "Strin Gauge 1"=0.0, "Strin Gauge 2"=0.0}, "Mod 2"={"Termocoppia 1"=0.0, "Termocoppia 2"=0.0, "Termocoppia 3"=0.0, "Termocoppia 4"=0.0}, "Mod 3"={"PT 100 1"=0.0, "PT 100 2"=0.0, "PT 100 3"=0.0, "PT 100 4"=0.0}}}, "MISURE WT"={"URMS 1"=0.0, "IRMS 1"=0.0, "P 1"=0.0, "S 1"=0.0, "Q 1"=0.0, "LAMBDA 1"=0.0, "PHI 1"=0.0, "F U 1"=0.0, "F I 1"=0.0, "NONE 1"=0.0, "URMS 2"=0.0, "IRMS 2"=0.0, "P 2"=0.0, "S 2"=0.0, "Q 2"=0.0, "LAMBDA 2"=0.0, "PHI 2"=0.0, "F U 2"=0.0, "F I 2"=0.0, "NONE 2"=0.0, "URMS 3"=0.0, "IRMS 3"=0.0, "P 3"=0.0, "S 3"=0.0, "Q 3"=0.0, "LAMBDA 3"=0.0, "PHI 3"=0.0, "F U 3"=0.0, "F I 3"=0.0, "NONE 3"=0.0, "URMS SIGMA"=0.0, "IRMS SIGMA"=0.0, "P SIGMA"=0.0, "S SIGMA"=0.0, "Q SIGMA"=0.0, "LAMBDA SIGMA"=0.0, "PHI SIGMA"=0.0, "F U SIGMA"=0.0, "F I SIGMA"=0.0, "NONE 4"=0.0}, "Resistenze Resistomat"={"Res Ch1"=0.0, "Res Ch2"=0.0, "Res Ch3"=0.0, "Tamb"=0.0}, "INTERFACCIA"={"AI"={"Portate"=[], "Pressioni"=[], "Coppie[Nm]"=[], "Valvole prop %"=[], "RPM"=[], "Livelli"=[], "Temperature"=[], "Riferimenti %"=[], "TENSIONI"=[], "CORRENTI"=[]}, "DI (logici)"={"Start da pulsantiera"=FALSE, "Stop da pulsantiera"=FALSE, "Reset da pulsantiera"=FALSE, "Sistema OK"=FALSE, "Collaudo abilitato"=FALSE, "Potenza trifase abilitata"=FALSE, "Potenza monofase abilitata"=FALSE, "Potenza DC abilitata"=FALSE, "Potenza DC ECC abilitata"=FALSE, "Start alimentazione AC"=FALSE, "Start alimentazione DC"=FALSE, "Start DC eccitazione"=FALSE, "Teleruttore WT abilitato"=FALSE, "Teleruttore Resistomat abilitato"=FALSE, "Teleruttore corto fasi"=FALSE, "Ramo 1 resistomat"=FALSE, "Ramo 2 resistomat"=FALSE, "Ramo 3 resistomat"=FALSE, "B1 Scelta linea elettrica 1"=FALSE, "B1 Scelta linea elettrica 2"=FALSE, "B1 Scelta linea elettrica 3"=FALSE, "B1 Scelta linea elettrica 4"=FALSE, "B1 Scelta linea elettrica 5"=FALSE, "B2 Scelta linea elettrica 1"=FALSE, "B2 Scelta linea elettrica 2"=FALSE, "B2 Scelta linea elettrica 3"=FALSE, "B2 Scelta linea elettrica 4"=FALSE, "B2 Scelta linea elettrica 5"=FALSE, "Rotore bloccato 1"=FALSE, "Rotore bloccato 2"=FALSE, "FRENO 1 abilitato"=FALSE, "FRENO 1 run"=FALSE, "FRENO 1 senso rotaz"=FALSE, "FRENO 1 ctrl velocità"=FALSE, "FRENO 2 abilitato"=FALSE, "FRENO 2 run"=FALSE, "FRENO 2 senso rotaz"=FALSE, "FRENO 2 ctrl velocità"=FALSE, "ALIM 1 abilitato"=FALSE, "ALIM 1 run"=FALSE, "ALIM 2 abilitato"=FALSE, "ALIM 2 run"=FALSE, "ALIM 3 abilitato"=FALSE, "ALIM 3 run"=FALSE, "FRENO 1 ctrl coppia"=FALSE, "FRENO 2 ctrl coppia"=FALSE, "FRENO 3 ctrl coppia"=FALSE, "DI (logici) aggiuntivi impianto"={"Solo freno abilitato"=FALSE, "Carico resistivo abilitato"=FALSE, "AFE+freno abilitato"=FALSE, "Protezioni chiuse"=FALSE, "Start potenza AFE"=FALSE, "AFE in marcia"=FALSE}, "Misura corrente diretta WT"=FALSE, "Misura corrente sens ext"=FALSE, "Sens ext abilitati"=FALSE}, "AO non scalati"={"FRENO1 rif vel"=0.0, "FRENO1 rif Coppia"=0.0, "FRENO2 rif vel"=0.0, "FRENO2 rif Coppia"=0.0, "ALIM1 rif V"=0.0, "ALIM1 rif F"=0.0, "ALIM2 rif V"=0.0, "ALIM2 rif F"=0.0, "ALIM3 rif V"=0.0, "ALIM3 rif F"=0.0, "Fnom keb"=0.0, "Rpm nom keb"=0.0, "Pnom keb"=0.0, "Inom keb"=0.0, "Vnom keb"=0.0, "Rpm max keb"=0.0, "Tempo rampa keb"=0.0, "Tipo Mot keb"=0.0, "FRENO  rif Coppia "=0.0, "FRENO  rif  Corrente"=0.0}, "AO scalati"={"FRENO1 rif vel"=0.0, "FRENO1 rif Coppia"=0.0, "FRENO2 rif vel"=0.0, "FRENO2 rif Coppia"=0.0, "ALIM1 rif V"=0.0, "ALIM1 rif F"=0.0, "ALIM2 rif V"=0.0, "ALIM2 rif F"=0.0, "ALIM3 rif V"=0.0, "ALIM3 rif F"=0.0, "Fnom keb"=0.0, "Rpm nom keb"=0.0, "Pnom keb"=0.0, "Inom keb"=0.0, "Vnom keb"=0.0, "Rpm max keb"=0.0, "Tempo rampa keb"=0.0, "Tipo Mot keb"=0.0, "FRENO  rif Coppia "=0.0, "FRENO  rif  Corrente"=0.0}, "DO (logici)"={"Scelta banco 1"=FALSE, "Scelta banco 2"=FALSE, "Scelta banco 3"=FALSE, "FRENO 1 abilita"=FALSE, "FRENO 1 start"=FALSE, "FRENO 1 senso rotaz"=FALSE, "FRENO 1 ctrl velocità"=FALSE, "FRENO 2 abilita"=FALSE, "FRENO 2 start"=FALSE, "FRENO 2 senso rotaz"=FALSE, "FRENO 2 ctrl velocità"=FALSE, "ALIM 1 abilita"=FALSE, "ALIM 1 start"=FALSE, "ALIM 2 abilita"=FALSE, "ALIM 2 start"=FALSE, "ALIM 3 abilita"=FALSE, "ALIM 3 start"=FALSE, "Abilita linea trifase"=FALSE, "Abilita linea monofase"=FALSE, "Abilita linea dc"=FALSE, "Abilita linea dc eccit"=FALSE, "B1 Linea elettrica 1"=FALSE, "B1 Linea elettrica 2"=FALSE, "B1 Linea elettrica 3"=FALSE, "B1 Linea elettrica 4"=FALSE, "B1 Linea elettrica 5"=FALSE, "B2 Linea elettrica 1"=FALSE, "B2 Linea elettrica 2"=FALSE, "B2 Linea elettrica 3"=FALSE, "B2 Linea elettrica 4"=FALSE, "B2 Linea elettrica 5"=FALSE, "Start potenza AC"=FALSE, "Stop pontenza AC"=FALSE, "Start potenza DC"=FALSE, "Stop potenza DC"=FALSE, "Start potenza eccitaz"=FALSE, "Stop potenza eccitaz"=FALSE, "Reset allarmi"=FALSE, "watchdog"=FALSE, "Scala torsiometro B1"=FALSE, "Controllo torsiom B1"=FALSE, "Scala torsiometro B2"=FALSE, "Controllo torsiom B2"=FALSE, "Teleruttore WT abilita"=FALSE, "Teleruttore Resistomat abilita"=FALSE, "Teleruttore corto fasi"=FALSE, "Ramo 1 resistomat"=FALSE, "Ramo 2 resistomat"=FALSE, "Ramo 3 resistomat"=FALSE, "Collaudo in corso"=FALSE, "Allarme presente"=FALSE, "Enable Res Meter"=FALSE, "Bypass Res Meter"=FALSE, "2nd canale Res Meter"=FALSE, "Scala 200/2000 res meter"=FALSE, "Taratura res meter"=FALSE, "FRENO 1 ctrl coppia"=FALSE, "FRENO 2 ctrl coppia"=FALSE, "FRENO 3 ctrl coppia"=FALSE, "Aggiuntivi impianto"={"Senso rotazione alim 1"=FALSE, "Senso rotazione alim 2"=FALSE}, "ALIM 1 stop"=FALSE, "ALIM 2 stop"=FALSE, "ALIM 3 stop"=FALSE, "FRENO 1 stop"=FALSE, "FRENO 2 stop"=FALSE, "FRENO 3 stop"=FALSE, "B1 configurazione freno B"=FALSE, "B2 configurazione freno B"=FALSE, "Abilita scrittura KEB"=FALSE, "Bench Selection (0-B1,1-B2)"=FALSE, "Select current mode"=FALSE, "Select torque mode"=FALSE, "Select speed mode"=FALSE, "Start"=FALSE, "Stop"=FALSE, "Block"=FALSE, "Enable Force mode"=FALSE, "Abilita linea 125 A"=FALSE, "Abilita linea 63 A"=FALSE, "Abilita linea 16 A"=FALSE, "Aum Tensione Variac"=FALSE, "Dim Tesnione Variac"=FALSE, "Abilita ellectro stractura"=FALSE, "Risprinito Emergence"=FALSE, "Abilita collaudo"=FALSE, "Disabilita collaudo"=FALSE, "External Alaram"=FALSE, "Enable external program"=FALSE, "Reset"=FALSE, "Abilita Ingresso Variac"=FALSE, "Abilita Ventilatore Variac"=FALSE, "Abilita Uscita Variac "=FALSE}}, "FREDDO resistomat"={"Res Ch1"=0.0, "Res Ch2"=0.0, "tAMB"=0.0, "Res Ch3"=0.0}, "STATO PLC 1"={"USCITE PLC"={"AO (real) 2"={"SCORTA 1"=0.0, "SCORTA 2"=0.0, "SCORTA 3"=0.0, "SCORTA 4"=0.0, "SCORTA 5"=0.0, "SCORTA 6"=0.0, "SCORTA 7"=0.0, "SCORTA 8"=0.0}, "statoAO_PLC out"={"Rif Lim coppia freno [%]"=nan, "Rif rpm freno [%]"=nan, "Rif coppia freno [%]"=0.0, "Rif V alimentatore [%]"=0.0, "Rif F alimentatore [%]"=0.0}, "DO (bit)"={"Scelta banco 1"=FALSE, "Set dati motore freno 2"=FALSE, "Diretto inverter"=FALSE, "Filtro LC"=FALSE, "Marcia ALIM (1s)"=FALSE, "Marcia FRENO (1s)"=FALSE, "Stop AFE (1s)"=FALSE, "Stop freno (1s)"=FALSE, "Reset allarmi"=FALSE, "Watchdog"=FALSE, "Senso rotazione"=FALSE, "Abilita collaudo (1s)"=FALSE, "Disabilita collaudo (1s)"=FALSE, "Abilitazione ALIM"=FALSE, "Abilitazione FRENO"=FALSE, "Teleruttore WT"=FALSE, "Senso rot motore prova"=FALSE, "Scorta 7"=FALSE, "Scorta 8"=FALSE, "Scorta 9"=FALSE, "Scorta 10"=FALSE, "Scorta 11"=FALSE, "Scorta 12"=FALSE, "Scorta 13"=FALSE}}, "Stato DI_PLC"={"Sistema OK"=FALSE, "Rotore bloccato"=FALSE, "Scorta 1"=FALSE, "Prova diretto inverter"=FALSE, "Prova con filtro LC"=FALSE, "Teleruttore WT abilitato"=FALSE, "Alim sinus penta abilitato"=FALSE, "Alim sinus penta in marcia"=FALSE, "Freno abilitato"=FALSE, "Freno in marcia"=FALSE, "Senso rotazione freno"=FALSE, "Potenza abilitata"=FALSE, "Scorta 3"=FALSE, "Scorta 4"=FALSE, "scorta 5"=FALSE, "scorta 6"=FALSE}, "AI plc"={"Allarmi 1"=0.0, "Allarmi 2"=0.0, "Scorta 1"=0.0, "Scorta 2"=0.0, "RPM mot prova"=0.0, "I mot prova"=0.0, "RPM freno"=0.0, "I freno"=0.0, "Scorta 3"=0.0, "Scorta 4"=0.0}}, "Res Ch2"=0.0, "Res Ch2 2"=0.0, "FREDDO res meter"={"Res Ch1"=0.0, "Res Ch2"=0.0, "tAMB"=0.0, "Res Ch3"=0.0}, "Resistenze Res Meter"={"Res Ch1"=0.0, "Res Ch2"=0.0, "Res Ch3"=0.0, "Tamb"=0.0}, "READ SINUS PENTA"={"Menù Misure motore (M000-M030)"={"Rif vel a regime (int)"=0, "Rif vel a regime (dec)"=0, "Rif vel dopo rampe (int)"=0, "Rif vel dopo rampe (dec)"=0, "RPM motore (int)"=0, "RPM motore (dec)"=0, "FREQout inverter"=0, "Rif coppia a regime(Nm)"=0, "Richiesta di coppia (Nm)"=0, "Coppia generata dal motore(Nm)"=0, "Rif coppia a regime(%)"=0, "Richiesta di coppia (%)"=0, "Coppia generata dal motore(%)"=0, "Coppia max richiesta prima delle rampe(Nm)"=0, "Coppia max richiesta dopo le rampe(Nm)"=0, "Limite di velocità prima delle rampe"=0, "Limite di velocità dopo le rampe"=0, "Coppia max richiesta prima delle rampe(%)"=0, "Coppia max richiesta dopo le rampe(%)"=0, "Rif di flusso"=0, "Corrente di uscita"=0, "Capacità termica del motore"=0, "Tensione di uscita"=0, "Potenza di uscita"=0, "Energia consumata (LSword)"=0, "Energia consumata (MSword)"=0, "Tensione bus DC"=0, "Tensione di rete"=0}, "Menù regolatore PID (M018-M024)"={"Rif PID a regime(%)"=0, "Rif pid dopo rampe(%)"=0, "Retroazione del pid(%)"=0, "Errore del pid(%)"=0, "uscita del pid(%)"=0, "Rif del pid dopo le rampe"=0, "Retroazione del pid"=0}, "Menù ingressi digitali (M031-M036)"={"Ingressi digitali ritardati"=0, "Ingressi digitali istantanei"=0, "Moresettiera comando loc"=0, "Morsett comando da seriale"=0, "Morsett comando bus di campo"=0, "Ing dig ausiliari da morsettiera"=0, "Ing dig ausiliari da seriale"=0}, "Menù riferimenti (M037-M051)"={"Rif analog est REF"=0, "Rif analog est AIN1"=0, "Rif analog est AIN2"=0, "Rif analog est XAIN4"=0, "Rif analog est XAIN5"=0, "Rif velocità da seriale(int)"=0, "Rif velocità bus di campo(int)"=0, "Rif coppia da seriale"=0, "Rif coppia bus di campo"=0, "Rif del PID da seriale"=0, "Rif del PID da bus di campo"=0, "Retroazione del PID da seriale"=0, "Retroazione del PIDda bus di campo"=0, "Rif da encoder"=0, "Rif in frequenza"=0, "Rif velocità da seriale(dec)"=0, "Rif velocità bus di campo(dec)"=0}, "Menù rampe (P009-P033)"={"Tempo di dec rampa di vel 1"=0, "Tempo di acc rampa di vel 2"=0, "Tempo di dec rampa di vel 2"=0, "Tempo di acc rampa di vel 1"=0, "Unità di mis tempi rampe vel 1/2"=0, "Tempo di acc rampa di vel 3"=0, "Tempo di dec rampa di vel 3"=0, "Tempo di acc rampa di vel 4"=0, "Tempo di dec rampa di vel 4"=0, "Unità di mis tempi rampe vel 3/4"=0, "Selettore arrottondam rampe"=0, "Tempo di arrotond iniz rampa acc"=0, "Tempo di arrotond finale rampa acc"=0, "Tempo di arrotond iniz rampa dec"=0, "Tempo di rampa di salita rif coppia"=0, "Tempo di rampa di discesa rif coppia"=0, "Unità di misura rampa coppia"=0, "Tempo rampa acc marcia jog"=0, "Tempo rampa dec marcia jog"=0, "Reset acc ai cambi pendenza"=0, "rampa di acc in fire mode"=0, "rampa di dec in fire mode"=0, "Tempo di arrotond finale rampa dec"=0}, "Menù controllo motore(C008-C128)"={"Numero motori configurati"=0, "Tipo algoritmo di controllo Mot1"=0, "Tipo rif Mot1"=0, "Tensione nominale rete"=0, "Retroaz di vel da encoder Mot1"=0, "Tipo curva V/f Mot1"=0, "Rotazione delle fasi Mot1"=0, "Freq nominale del motore Mot1"=0, "RPM nominali del motore Mot1"=0, "Potenza nominale del motore Mot1"=0, "Corrente nominale del motore Mot1"=0, "Tensione nominale del motore mot1"=0, "Potenza a vuoto del motore Mot1"=0, "Corrente a vuoto del motore Mot1"=0, "Resistenza statorica del motore Mot1"=0, "Induttanza di dispersione Mot1"=0, "Induttanza mutua motore"=0, "Costante di tempo rotorica"=0, "Costante di tempo filtro pb"=0, "Velocità minima motore"=0, "Velocità massima motore"=0}, "Menù configurazione PID"={"Selezione riferimento n.1"=0, "Selezione retroazione n.1"=0, "Modalità di fuzionamento PID"=0, "Termine derivativo calcolato su err o mis"=0, "Proporz moltiplica deriv e integrale"=0, "Azione del PID"=0}, "ID"=0.0, "Menù uscite digitali"={"MDO4 Inverter pronto"=0}, "Fcarrier"={"Fcarrier Min (Hz)"=0, "Fcarrier Max (Hz)"=0}, "stato inverter M089"=0.0, "Riferimenti"={"Rif tensione"=0, "Rif velocità"=0}, "Comunicazione"=FALSE, "Modalità stop"=0.0}, "STATO PLC 2"={"USCITE PLC"={"AO (real) 2"={"SCORTA 1"=0.0, "SCORTA 2"=0.0, "SCORTA 3"=0.0, "SCORTA 4"=0.0, "SCORTA 5"=0.0, "SCORTA 6"=0.0, "SCORTA 7"=0.0, "SCORTA 8"=0.0}, "statoAO_PLC out"={"Condensatori"=0.0, "Scorta 1"=0.0, "Scorta 2"=0.0}, "DO (bit)"={"Relè misura resistomat"=FALSE, "Misura res ramo 1"=FALSE, "Misura res ramo 2"=FALSE, "Misura res ramo 3"=FALSE, "Scelta banco 2"=FALSE, "Scala Torsiometro"=FALSE, "Ctrl torsiometro"=FALSE, "Select current mode"=FALSE, "Select Torque mode"=FALSE, "Select speed mode"=FALSE, "Watchdog"=FALSE, "Scorta"=FALSE, "Scorta 2"=FALSE, "Scorta 3"=FALSE, "Scorta 4"=FALSE, "Scorta 5"=FALSE, "Bench selection"=FALSE, "External alarm"=FALSE, "Enable external program"=FALSE, "Reset allarmi"=FALSE, "Start"=FALSE, "Stop"=FALSE, "Block"=FALSE, "Scorta 6"=FALSE}}, "Stato DI_PLC"={"Sistema ok"=FALSE, "Relè Resistomat abilitato"=FALSE, "Freno abilitato"=FALSE, "Freno in marcia"=FALSE, "scorta b"=FALSE, "scorta a"=FALSE, "scorta 1"=FALSE, "scorta 2"=FALSE, "scorta 3"=FALSE, "scorta 4"=FALSE, "Scorta 5"=FALSE, "Scorta 6"=FALSE, "Scorta 7"=FALSE, "Scorta 8"=FALSE, "Scorta 9"=FALSE, "Scorta 10"=FALSE}, "AI plc"={"Allarmi 1"=0.0, "Allarmi 2"=0.0, "TC 1"=0.0, "TC 2"=0.0, "TC 3"=0.0, "TC 4"=0.0, "TC 5"=0.0, "TC 6"=0.0, "TC 7"=0.0, "TC 8"=0.0, "PT1000 1"=0.0, "PT1000 2"=0.0, "PT1000 3"=0.0, "PT1000 4"=0.0}}, "STATO PLC 3"={"USCITE PLC"={"AO (real) 2"={"SCORTA 1"=0.0, "SCORTA 2"=0.0, "SCORTA 3"=0.0, "SCORTA 4"=0.0, "SCORTA 5"=0.0, "SCORTA 6"=0.0, "SCORTA 7"=0.0, "SCORTA 8"=0.0}, "statoAO_PLC out"={"Rif velocità alimentatore"=0.0, "Scorta"=0.0, "Tipo Motore  keb"=0.0, "I nom keb"=0.0, "RPM nom keb"=0.0, "V nom keb"=0.0, "F nom keb"=0.0, "t rampa keb"=0.0}, "DO (bit)"={"Select linea Inverter"=FALSE, "Abilita sense wattmetro"=FALSE, "Bypass filtro LC"=FALSE, "Filtro LC"=FALSE, "Bypass trasformatore"=FALSE, "Trasformatore"=FALSE, "Abilita uscite variac"=FALSE, "Abilita linea 125 A"=FALSE, "Abilita linea 63 A"=FALSE, "Abilita linea 16 A"=FALSE, "Abilita Scrittura Dati Keb"=FALSE, "Abilita alimentatore"=FALSE, "Marcia alimentatore (1s)"=FALSE, "Stop alimentatore (1s)"=FALSE, "Senso rot mot prova"=FALSE, "Watchdog"=FALSE, "Aumenta tensione variac"=FALSE, "Diminuisci tensione variac "=FALSE, "Blocco elettroserrature"=FALSE, "Ripristino emergence"=FALSE, "Abilita ingresso variac"=FALSE, "Abilita ventilatore variac"=FALSE, "Reset Allarm"=FALSE, "Scorta 1"=FALSE, "Scorta 2"=FALSE, "Scorta 3"=FALSE, "Scorta 4"=FALSE, "Scorta 5"=FALSE, "Scorta 6"=FALSE, "Scorta 7"=FALSE, "Scorta 8"=FALSE, "Scorta 9"=FALSE, "Abilita collaudo"=FALSE, "Disabilita collaudo "=FALSE, "Scorta 10"=FALSE, "Scorta 11"=FALSE, "Scorta 12"=FALSE, "Scorta 13"=FALSE, "Scorta 14"=FALSE, "Scorta 15"=FALSE}}, "Stato DI_PLC"={"Sistema OK"=FALSE, "Rotore bloccato"=FALSE, "Filtro LC"=FALSE, "Bypass Filtro LC"=FALSE, "Scelta Trasformatore"=FALSE, "Scelta Bypass trasformatore"=FALSE, "Teleruttore wt abilitato"=FALSE, "Alimentatore abilitato"=FALSE, "Alimentatore in marcia"=FALSE, "Scorta 1"=FALSE, "Scorta 2"=FALSE, "Scorta 3"=FALSE, "Potenza abilitata"=FALSE, "Alimentatore in allarme"=FALSE, "Scorta 4"=FALSE, "Conferma dati KEB"=FALSE, "Scorta 5"=FALSE, "Warning Inverter Alimentatore"=FALSE, "Variac Abilitato"=FALSE, "Linea 125 A abilitata"=FALSE, "Linea 63 A abilitata"=FALSE, "Linea 16 A abilitata"=FALSE, "Scorta 6"=FALSE, "Enable force mode"=FALSE}, "AI plc"={"Allarmi 1"=0.0, "Allarmi 2"=0.0, "RPM motore prova"=0.0, "Corrente motore prova"=0.0, "RPM freno"=0.0, "Corrente freno"=0.0, "Tipo motore keb"=0.0, "I nom keb"=0.0, "RPM nom keb"=0.0, "V nom keb"=0.0, "F nom keb"=0.0, "T rampa keb"=0.0, "scorta"=0.0, "Scorta 2"=0.0}}, "DCREG"={"Parametri di misura"={"M000"=0.0, "M001"=0.0, "M002"=0.0, "M003"=0.0, "M004"=0.0, "M005"=0.0, "M006"=0.0, "M007"=0.0, "M008"=0.0, "M009"=0.0, "M010"=0.0, "M011"=0.0, "M012"=0.0, "M013"=0.0, "M014"=0.0, "M015"=0.0, "M016"=0.0, "M017"=0.0, "M018"=0.0, "M019"=0.0, "M020"=0.0, "M021"=0.0, "M022"=0.0, "M023"=0.0, "M024"=0.0, "M025"=0.0, "M026"=0.0, "M027"=0.0, "M028"=0.0, "M029"=0.0, "M030"=0.0, "M031"=0.0}, "Parametri di programmazione"={"P000"=0.0, "P001"=0.0, "P002"=0.0, "P003"=0.0, "P004"=0.0, "P005"=0.0, "P006"=0.0, "P010"=0.0, "P011"=0.0, "P012"=0.0, "P013"=0.0, "P014"=0.0, "P015"=0.0, "P016"=0.0, "P030"=0.0, "P031"=0.0, "P032"=0.0, "P033"=0.0, "P034"=0.0, "P035"=0.0, "P036"=0.0, "P037"=0.0, "P038"=0.0, "P039"=0.0, "P040"=0.0, "P050"=0.0, "P051"=0.0, "P052"=0.0, "P053"=0.0, "P054"=0.0, "P055"=0.0, "P056"=0.0, "P057"=0.0, "P058"=0.0, "P059"=0.0, "P060"=0.0, "P061"=0.0, "P062"=0.0, "P070"=0.0, "P071"=0.0, "P073"=0.0, "P074"=0.0, "P076"=0.0, "P077"=0.0, "P079"=0.0, "P080"=0.0, "P082"=0.0, "P083"=0.0, "P084"=0.0, "P085"=0.0, "P086"=0.0, "P087"=0.0, "P088"=0.0, "P100"=0.0, "P101"=0.0, "P102"=0.0, "P103"=0.0, "P104"=0.0, "P110"=0.0, "P111"=0.0, "P120"=0.0, "P121"=0.0, "P122"=0.0, "P123"=0.0, "P124"=0.0, "P125"=0.0, "P126"=0.0, "P127"=0.0, "P128"=0.0, "P129"=0.0, "P130"=0.0, "P131"=0.0, "P132"=0.0, "P133"=0.0, "P134"=0.0, "P150"=0.0, "P151"=0.0, "P152"=0.0, "P153"=0.0, "P154"=0.0, "P155"=0.0, "P156"=0.0, "P157"=0.0, "P158"=0.0, "P170"=0.0, "P171"=0.0, "P172"=0.0, "P173"=0.0, "P174"=0.0, "P175"=0.0, "P176"=0.0, "P177"=0.0, "P178"=0.0, "P179"=0.0, "P180"=0.0, "P181"=0.0, "P182"=0.0, "P183"=0.0, "P184"=0.0, "P185"=0.0, "P186"=0.0, "P187"=0.0, "P188"=0.0, "P189"=0.0, "P190"=0.0, "P191"=0.0, "P192"=0.0, "P193"=0.0, "P194"=0.0, "P195"=0.0, "P196"=0.0, "P197"=0.0, "P198"=0.0, "P199"=0.0, "P211"=0.0, "P212"=0.0, "P213"=0.0, "P214"=0.0, "P215"=0.0, "P216"=0.0, "P217"=0.0, "P221"=0.0, "P222"=0.0, "P223"=0.0, "P224"=0.0, "P230"=0.0, "P231"=0.0, "P240"=0.0, "P250"=0.0, "P251"=0.0}, "Parametri di configurazione"={"C000"=0.0, "C001"=0.0, "C002"=0.0, "C010"=0.0, "C011"=0.0, "C012"=0.0, "C014"=0.0, "C015"=0.0, "C016"=0.0, "C017"=0.0, "C018"=0.0, "C030"=0.0, "C050"=0.0, "C051"=0.0, "C052"=0.0, "C060"=0.0, "C061"=0.0, "C062"=0.0, "C063"=0.0, "C070"=0.0, "C072"=0.0, "C074"=0.0, "C090"=0.0, "C091"=0.0, "C092"=0.0, "C093"=0.0, "C094"=0.0, "C100"=0.0, "C101"=0.0, "C102"=0.0, "C103"=0.0, "C105"=0.0, "C106"=0.0, "C107"=0.0, "C108"=0.0, "C110"=0.0, "C111"=0.0, "C112"=0.0, "C120"=0.0, "C121"=0.0, "C122"=0.0, "C130"=0.0, "C131"=0.0, "C132"=0.0, "C133"=0.0, "C134"=0.0, "C135"=0.0, "C141"=0.0, "C142"=0.0, "C143"=0.0, "C150"=0.0, "C151"=0.0, "C153"=0.0, "C154"=0.0, "C155"=0.0, "C156"=0.0, "C157"=0.0, "C158"=0.0, "C159"=0.0, "C160"=0.0, "C161"=0.0, "C162"=0.0, "C163"=0.0, "C164"=0.0, "C165"=0.0, "C170"=0.0}, "Codice allarme"=0.0, "Comunicazione"=FALSE}}} {"MISURE ALL"."Cluster READ NI"."AI (4-20mA)"."AI 15" format="%#_6f"; "MISURE ALL"."Cluster READ NI"."AI (4-20mA)"."AI 14" format="%#_6f"; "MISURE ALL"."Cluster READ NI"."AI (4-20mA)"."AI 13" format="%#_6f"; "MISURE ALL"."Cluster READ NI"."AI (4-20mA)"."AI 11" format="%#_6f"; "MISURE ALL"."Cluster READ NI"."AI (4-20mA)"."AI 10" format="%#_6f"; "MISURE ALL"."Cluster READ NI"."AI (4-20mA)"."AI 9" format="%#_6f"; "MISURE ALL"."Cluster READ NI"."AI (4-20mA)"."AI 4" format="%#_6f"; "MISURE ALL"."Cluster READ NI"."AI (4-20mA)"."AI 12" format="%#_6f"; "MISURE ALL"."Cluster READ NI"."AI (4-20mA)"."AI 0" format="%#_6f"; "MISURE ALL"."Cluster READ NI"."AI (4-20mA)"."AI 1" format="%#_6f"; "MISURE ALL"."Cluster READ NI"."AI (4-20mA)"."AI 2" format="%#_6f"; "MISURE ALL"."Cluster READ NI"."AI (4-20mA)"."AI 3" format="%#_6f"; "MISURE ALL"."Cluster READ NI"."AI (4-20mA)"."AI 5" format="%#_6f"; "MISURE ALL"."Cluster READ NI"."AI (4-20mA)"."AI 6" format="%#_6f"; "MISURE ALL"."Cluster READ NI"."AI (4-20mA)"."AI 7" format="%#_6f"; "MISURE ALL"."Cluster READ NI"."AI (4-20mA)"."AI 8" format="%#_6f"; "MISURE ALL"."Cluster READ NI"."AI (0-10V)"."AI 31" format="%#_6f"; "MISURE ALL"."Cluster READ NI"."AI (0-10V)"."AI 30" format="%#_6f"; "MISURE ALL"."Cluster READ NI"."AI (0-10V)"."AI 29" format="%#_6f"; "MISURE ALL"."Cluster READ NI"."AI (0-10V)"."AI 28" format="%#_6f"; "MISURE ALL"."Cluster READ NI"."AI (0-10V)"."AI 27" format="%#_6f"; "MISURE ALL"."Cluster READ NI"."AI (0-10V)"."AI 26" format="%#_6f"; "MISURE ALL"."Cluster READ NI"."AI (0-10V)"."AI 25" format="%#_6f"; "MISURE ALL"."Cluster READ NI"."AI (0-10V)"."AI 24" format="%#_6f"; "MISURE ALL"."Cluster READ NI"."AI (0-10V)"."AI 23" format="%#_6f"; "MISURE ALL"."Cluster READ NI"."AI (0-10V)"."AI 22" format="%#_6f"; "MISURE ALL"."Cluster READ NI"."AI (0-10V)"."AI 21" format="%#_6f"; "MISURE ALL"."Cluster READ NI"."AI (0-10V)"."AI 20" format="%#_6f"; "MISURE ALL"."Cluster READ NI"."AI (0-10V)"."AI 19" format="%#_6f"; "MISURE ALL"."Cluster READ NI"."AI (0-10V)"."AI 18" format="%#_6f"; "MISURE ALL"."Cluster READ NI"."AI (0-10V)"."AI 17" format="%#_6f"; "MISURE ALL"."Cluster READ NI"."AI (0-10V)"."AI 16" format="%#_6f"; "MISURE ALL"."Cluster READ NI"."AI (0-10V)"."AI 15" format="%#_6f"; "MISURE ALL"."Cluster READ NI"."AI (0-10V)"."AI 14" format="%#_6f"; "MISURE ALL"."Cluster READ NI"."AI (0-10V)"."AI 13" format="%#_6f"; "MISURE ALL"."Cluster READ NI"."AI (0-10V)"."AI 11" format="%#_6f"; "MISURE ALL"."Cluster READ NI"."AI (0-10V)"."AI 10" format="%#_6f"; "MISURE ALL"."Cluster READ NI"."AI (0-10V)"."AI 9" format="%#_6f"; "MISURE ALL"."Cluster READ NI"."AI (0-10V)"."AI 4" format="%#_6f"; "MISURE ALL"."Cluster READ NI"."AI (0-10V)"."AI 12" format="%#_6f"; "MISURE ALL"."Cluster READ NI"."AI (0-10V)"."AI 0" format="%#_6f"; "MISURE ALL"."Cluster READ NI"."AI (0-10V)"."AI 1" format="%#_6f"; "MISURE ALL"."Cluster READ NI"."AI (0-10V)"."AI 2" format="%#_6f"; "MISURE ALL"."Cluster READ NI"."AI (0-10V)"."AI 3" format="%#_6f"; "MISURE ALL"."Cluster READ NI"."AI (0-10V)"."AI 5" format="%#_6f"; "MISURE ALL"."Cluster READ NI"."AI (0-10V)"."AI 6" format="%#_6f"; "MISURE ALL"."Cluster READ NI"."AI (0-10V)"."AI 7" format="%#_6f"; "MISURE ALL"."Cluster READ NI"."AI (0-10V)"."AI 8" format="%#_6f"})   [LabVIEW 2019]
uses:
  TypeDef/Cluster INFO.ctl
  TypeDef/WT SELECTION.ctl
  TypeDef/Definizione linea.ctl
  TypeDef/Collegamenti_elettrici.ctl
  TypeDef/Control Calcoli.ctl
  TypeDef/Cluster MISURE.ctl
  TypeDef/MISURE NM.ctl
  TypeDef/Cluster misure ALL.ctl
  TypeDef/Cluster NI.ctl
  cDAQ_PLC Folder/controls/StatoAO_cdaq.ctl
  cDAQ_PLC Folder/controls/statoDO_Cdaq.ctl
  TypeDef/MISURE WT.ctl
  TypeDef/ClusterRes.ctl
  TypeDef/INTERFACCIA.ctl
  TypeDef/Lista AO sistema.ctl
  TypeDef/DOinterfaccia.ctl
  cDAQ_PLC Folder/ST1200_LIST_IO/STATO PLC 1.ctl
  cDAQ_PLC Folder/ST1200_LIST_IO/Uscite PLC 1.ctl
  cDAQ_PLC Folder/controls/statoAO_plc_1.ctl
  cDAQ_PLC Folder/ST1200_LIST_IO/StatoDO_PLC_1.ctl
  SINUS PENTA SANTERNO/controls/Parametri inverter letti.ctl
  cDAQ_PLC Folder/ST1200_LIST_IO/STATO PLC 2.ctl
  cDAQ_PLC Folder/ST1200_LIST_IO/Uscite PLC 2.ctl
  cDAQ_PLC Folder/controls/statoAO_plc_2.ctl
  cDAQ_PLC Folder/ST1200_LIST_IO/StatoDO_PLC_2.ctl
  cDAQ_PLC Folder/ST1200_LIST_IO/STATO PLC 3.ctl
  cDAQ_PLC Folder/ST1200_LIST_IO/Uscite PLC 3.ctl
  cDAQ_PLC Folder/controls/statoAO_plc_3.ctl
  cDAQ_PLC Folder/ST1200_LIST_IO/StatoDO_PLC_3.ctl
  DCREG/Parametri DCREG letti.ctl
  cDAQ_PLC Folder/cDAQ/SET ARRAY DO.ctl
  cDAQ_PLC Folder/cDAQ/SET SINGLE DO.ctl
  cDAQ_PLC Folder/cDAQ/DO List.ctl
  Global procedura abilitata.vi
  Linea idraulica selezionata.vi
  Prova selezionata.vi
  Global prova in corso.vi
  Stato comandi freno.vi
  Stato alimentatore 1.vi
  Global compensazione attriti.vi
  Global grandezze linea.vi
  <vilib>/ptbypt/NI_PtbyPt.lvlib
panel:
  in  "Descrizione":string
  in  "Reset":bool
  in  "Array":T1(array[cluster])
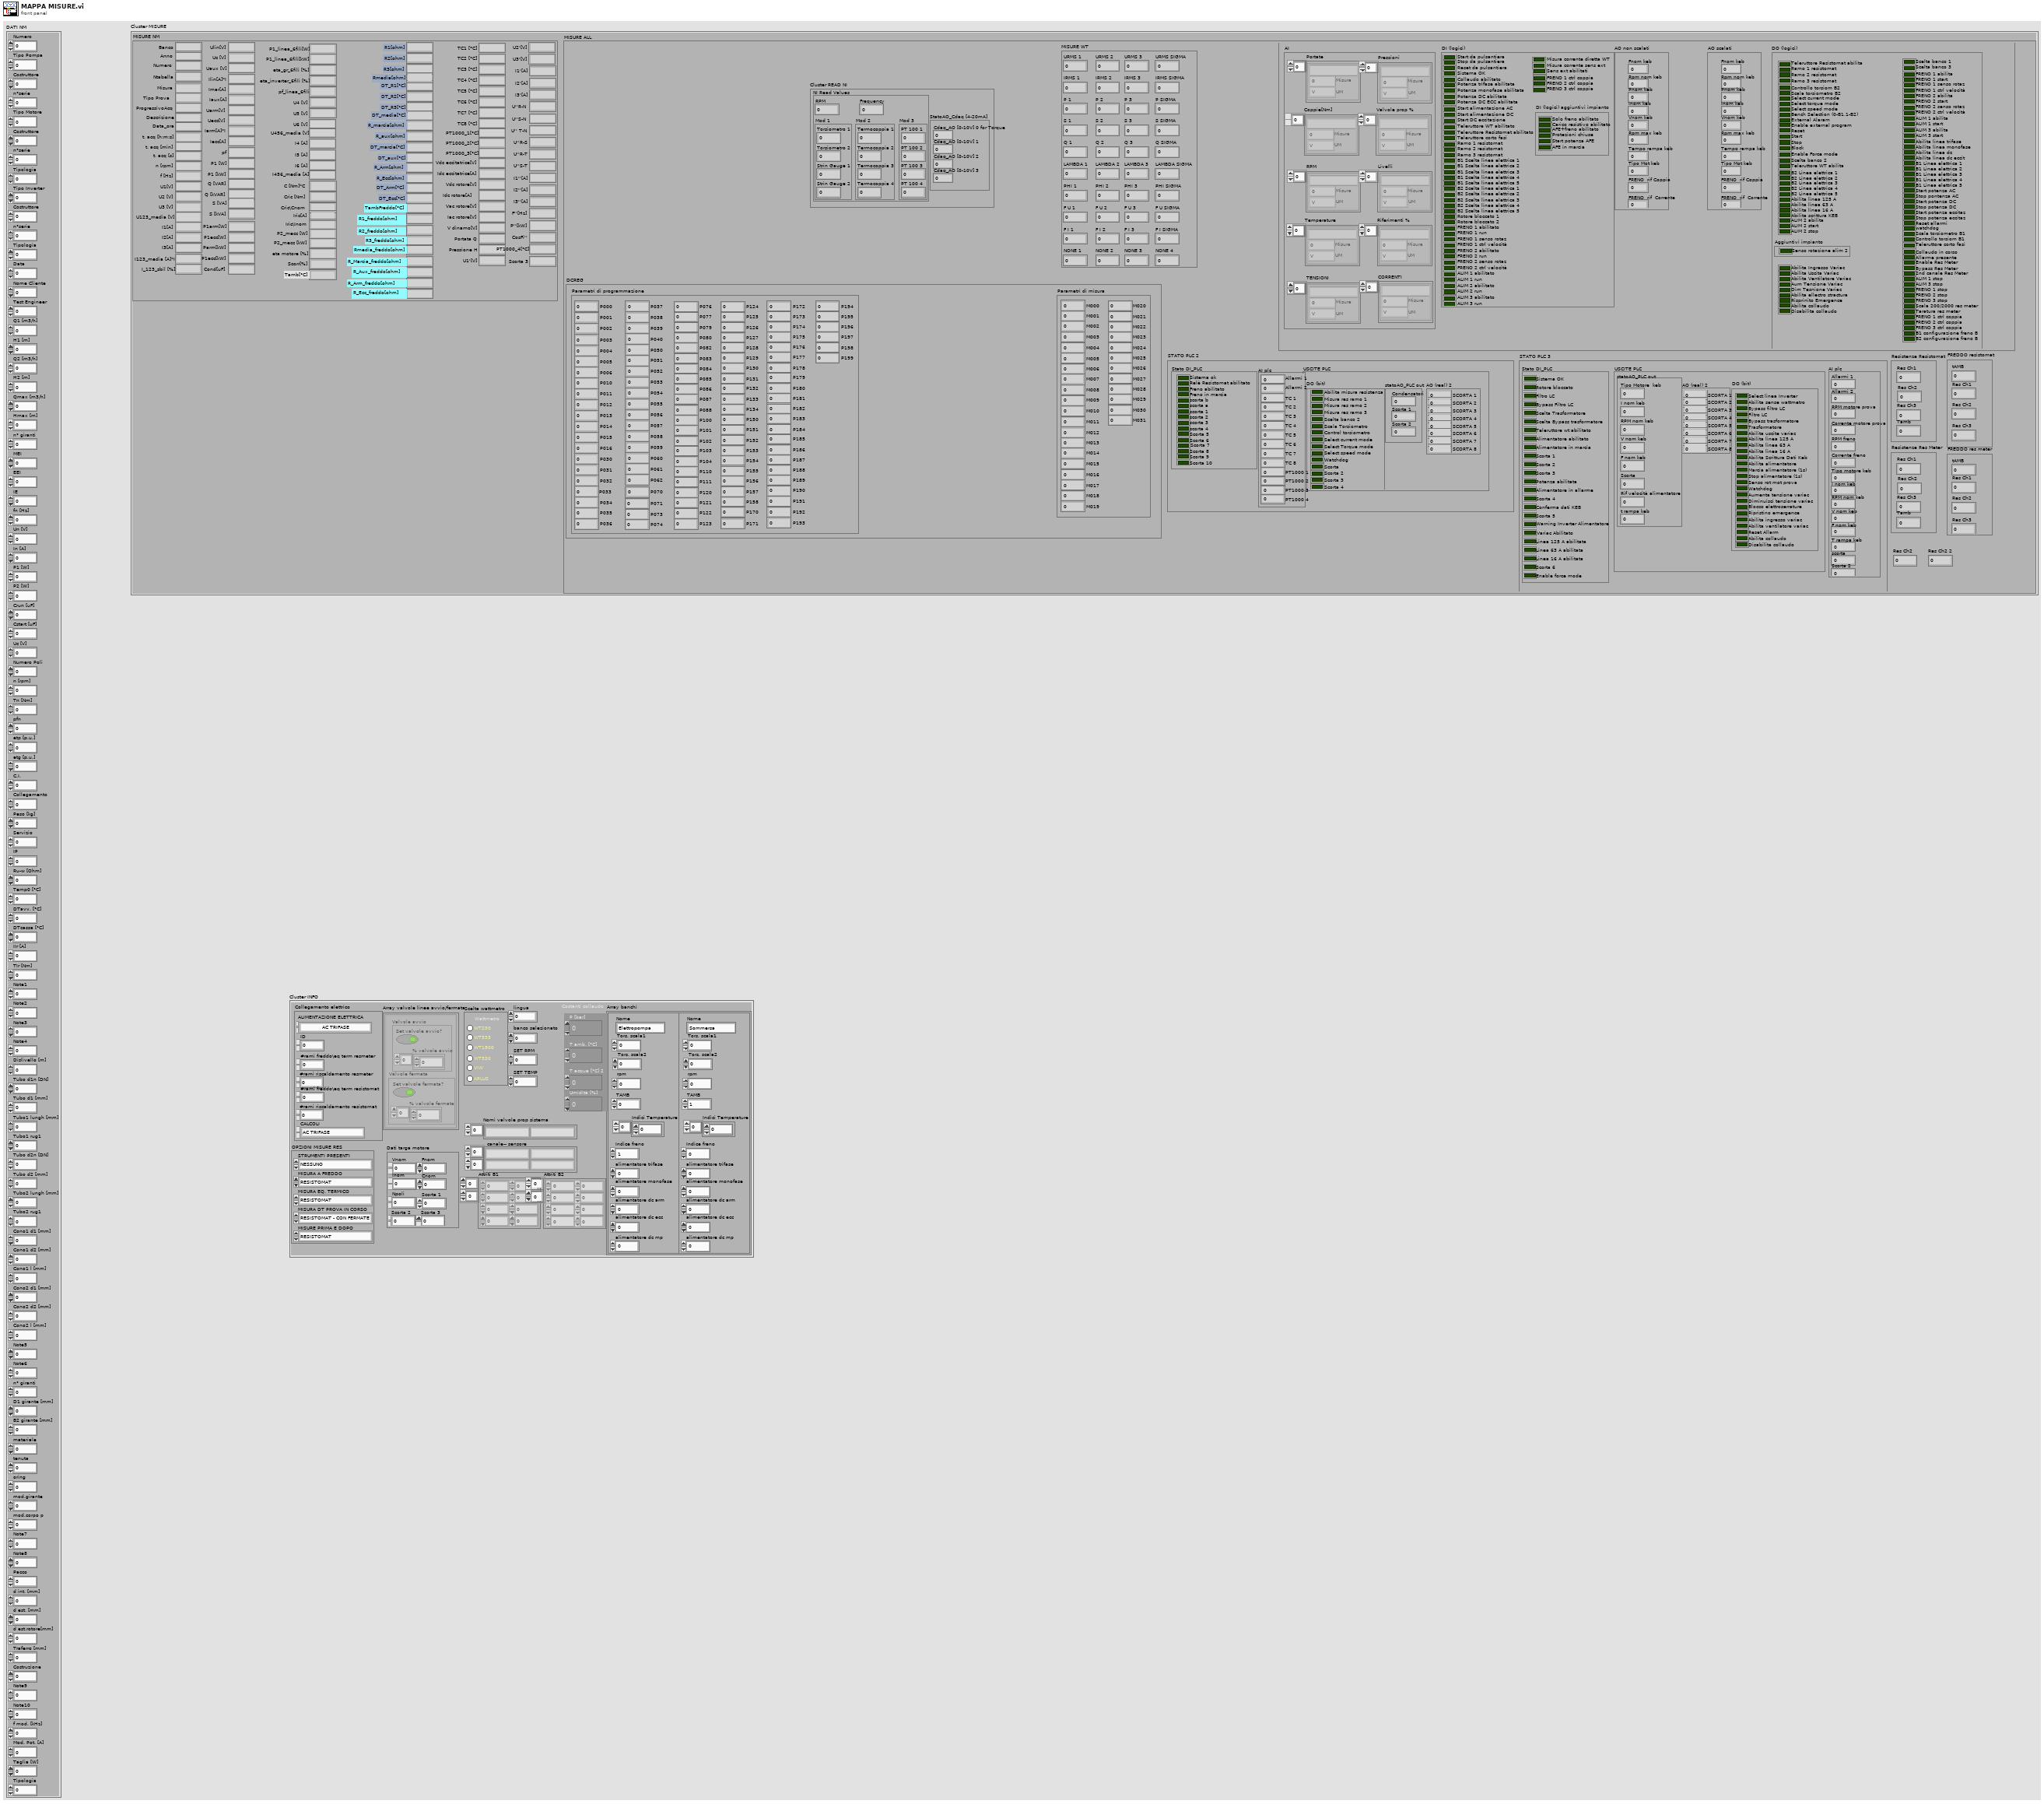
[diagram p1: front panel]
types:
  T1 = cluster{"portata":i32, "Hasp":i32, "Hmand":i32, "Torsiometro":i32, "rpm":i32, "Hdiff?":bool}[]
  T2 = typedef "Cluster misure ALL.ctl" = cluster{"Cluster READ NI":T3, "MISURE WT":T6, "Resistenze Resistomat":T7, "INTERFACCIA":T8, "FREDDO resistomat":cluster{"Res Ch1":dbl, "Res Ch2":dbl, "tAMB":dbl, "Res Ch3":dbl}, "STATO PLC 1":T13, "Res Ch2":dbl, "Res Ch2 2":dbl, "FREDDO res meter":cluster{"Res Ch1":dbl, "Res Ch2":dbl, "tAMB":dbl, "Res Ch3":dbl}, "Resistenze Res Meter":T7, "READ SINUS PENTA":T17, "STATO PLC 2":T18, "STATO PLC 3":T22, "DCREG":T26}
  T3 = typedef "Cluster NI.ctl" = cluster{"AI (0-10V)":cluster{"AI 0":dbl, "AI 1":dbl, "AI 2":dbl, "AI 3":dbl, "AI 4":dbl, "AI 5":dbl, "AI 6":dbl, "AI 7":dbl, "AI 8":dbl, "AI 9":dbl, "AI 10":dbl, "AI 11":dbl, "AI 12":dbl, "AI 13":dbl, "AI 14":dbl, "AI 15":dbl, "AI 16":dbl, "AI 17":dbl, "AI 18":dbl, "AI 19":dbl, "AI 20":dbl, "AI 21":dbl, "AI 22":dbl, "AI 23":dbl, "AI 24":dbl, "AI 25":dbl, "AI 26":dbl, "AI 27":dbl, "AI 28":dbl, "AI 29":dbl, "AI 30":dbl, "AI 31":dbl}, "StatoAO_Cdaq[0-10V]":cluster{"AO 1":dbl, "AO 2":dbl, "AO 3":dbl, "AO 4":dbl}, "Contatori [rpm]":cluster{"RPM 1":dbl, "RPM 2":dbl}, "StatoAO_Cdaq [4-20mA]":T4, "StatoDO_Cdaq":T5, "DI":cluster{"Scorta 0":bool, "Scorta 1":bool, "Scorta 2":bool, "Scorta 3":bool, "Scorta 4":bool, "Scorta 5":bool, "Scorta 6":bool, "Scorta 7":bool, "Scorta 8":bool, "Scorta 9":bool, "Scorta 10":bool, "Scorta 11":bool, "Scorta 12":bool, "Scorta 13":bool, "Scorta 14":bool, "Scorta 15":bool, "Scorta 16":bool, "Scorta 17":bool, "Scorta 18":bool, "Scorta 19":bool, "Scorta 20":bool, "Scorta 21":bool, "Scorta 22":bool, "Scorta 23":bool, "Scorta 24":bool, "Scorta 25":bool, "Scorta 26":bool, "Scorta 27":bool, "Scorta 28":bool, "Scorta 29":bool, "Scorta 30":bool, "Scorta 31":bool}, "AI (4-20mA)":cluster{"AI 0":dbl, "AI 1":dbl, "AI 2":dbl, "AI 3":dbl, "AI 4":dbl, "AI 5":dbl, "AI 6":dbl, "AI 7":dbl, "AI 8":dbl, "AI 9":dbl, "AI 10":dbl, "AI 11":dbl, "AI 12":dbl, "AI 13":dbl, "AI 14":dbl, "AI 15":dbl}, "TC [°C]":cluster{"tc 1":dbl, "tc 2":dbl, "tc 3":dbl, "tc 4":dbl}, "NI Read Values":cluster{"RPM":dbl, "Frequency":dbl, "Mod 1":cluster{"Torsiometro 1":dbl, "Torsiometro 2":dbl, "Strin Gauge 1":dbl, "Strin Gauge 2":dbl}, "Mod 2":cluster{"Termocoppia 1":dbl, "Termocoppia 2":dbl, "Termocoppia 3":dbl, "Termocoppia 4":dbl}, "Mod 3":cluster{"PT 100 1":dbl, "PT 100 2":dbl, "PT 100 3":dbl, "PT 100 4":dbl}}}
  T4 = typedef "StatoAO_cdaq.ctl" = cluster{"Cdaq_AO [0-10V] 0 for Torque":dbl, "Cdaq_AO [0-10V] 1":dbl, "Cdaq_AO [0-10V] 2":dbl, "Cdaq_AO [0-10V] 3":dbl}
  T5 = typedef "statoDO_Cdaq.ctl" = cluster{"Scorta 0":bool, "Scorta 1":bool, "Scorta 2":bool, "Scorta 3":bool, "Scorta 4":bool, "Scorta 5":bool, "Scorta 6":bool, "Scorta 7":bool, "Scorta 8":bool, "Scorta 9":bool, "Scorta 10":bool, "Scorta 11":bool, "Scorta 12":bool, "Scorta 13":bool, "Scorta 14":bool, "Scorta 15":bool, "Scorta 16":bool, "Scorta 17":bool, "Scorta 18":bool, "Scorta 19":bool, "Scorta 20":bool, "Scorta 21":bool, "Scorta 22":bool, "Scorta 23":bool, "Scorta 24":bool, "Scorta 25":bool, "Scorta 26":bool, "Scorta 27":bool, "Scorta 28":bool, "Scorta 29":bool, "Scorta 30":bool, "Scorta 31":bool}
  T6 = typedef "MISURE WT.ctl" = cluster{"URMS 1":dbl, "IRMS 1":dbl, "P 1":dbl, "S 1":dbl, "Q 1":dbl, "LAMBDA 1":dbl, "PHI 1":dbl, "F U 1":dbl, "F I 1":dbl, "NONE 1":dbl, "URMS 2":dbl, "IRMS 2":dbl, "P 2":dbl, "S 2":dbl, "Q 2":dbl, "LAMBDA 2":dbl, "PHI 2":dbl, "F U 2":dbl, "F I 2":dbl, "NONE 2":dbl, "URMS 3":dbl, "IRMS 3":dbl, "P 3":dbl, "S 3":dbl, "Q 3":dbl, "LAMBDA 3":dbl, "PHI 3":dbl, "F U 3":dbl, "F I 3":dbl, "NONE 3":dbl, "URMS SIGMA":dbl, "IRMS SIGMA":dbl, "P SIGMA":dbl, "S SIGMA":dbl, "Q SIGMA":dbl, "LAMBDA SIGMA":dbl, "PHI SIGMA":dbl, "F U SIGMA":dbl, "F I SIGMA":dbl, "NONE 4":dbl}
  T7 = typedef "ClusterRes.ctl" = cluster{"Res Ch1":dbl, "Res Ch2":dbl, "Res Ch3":dbl, "Tamb":dbl}
  T8 = typedef "INTERFACCIA.ctl" = cluster{"AI":cluster{"Portate":T9[], "Pressioni":T9[], "Coppie[Nm]":T9[], "Valvole prop %":T9[], "RPM":T9[], "Livelli":T9[], "Temperature":T9[], "Riferimenti %":T9[], "TENSIONI":T9[], "CORRENTI":T9[]}, "DI (logici)":cluster{"Start da pulsantiera":bool, "Stop da pulsantiera":bool, "Reset da pulsantiera":bool, "Sistema OK":bool, "Collaudo abilitato":bool, "Potenza trifase abilitata":bool, "Potenza monofase abilitata":bool, "Potenza DC abilitata":bool, "Potenza DC ECC abilitata":bool, "Start alimentazione AC":bool, "Start alimentazione DC":bool, "Start DC eccitazione":bool, "Teleruttore WT abilitato":bool, "Teleruttore Resistomat abilitato":bool, "Teleruttore corto fasi":bool, "Ramo 1 resistomat":bool, "Ramo 2 resistomat":bool, "Ramo 3 resistomat":bool, "B1 Scelta linea elettrica 1":bool, "B1 Scelta linea elettrica 2":bool, "B1 Scelta linea elettrica 3":bool, "B1 Scelta linea elettrica 4":bool, "B1 Scelta linea elettrica 5":bool, "B2 Scelta linea elettrica 1":bool, "B2 Scelta linea elettrica 2":bool, "B2 Scelta linea elettrica 3":bool, "B2 Scelta linea elettrica 4":bool, "B2 Scelta linea elettrica 5":bool, "Rotore bloccato 1":bool, "Rotore bloccato 2":bool, "FRENO 1 abilitato":bool, "FRENO 1 run":bool, "FRENO 1 senso rotaz":bool, "FRENO 1 ctrl velocità":bool, "FRENO 2 abilitato":bool, "FRENO 2 run":bool, "FRENO 2 senso rotaz":bool, "FRENO 2 ctrl velocità":bool, "ALIM 1 abilitato":bool, "ALIM 1 run":bool, "ALIM 2 abilitato":bool, "ALIM 2 run":bool, "ALIM 3 abilitato":bool, "ALIM 3 run":bool, "FRENO 1 ctrl coppia":bool, "FRENO 2 ctrl coppia":bool, "FRENO 3 ctrl coppia":bool, "DI (logici) aggiuntivi impianto":cluster{"Solo freno abilitato":bool, "Carico resistivo abilitato":bool, "AFE+freno abilitato":bool, "Protezioni chiuse":bool, "Start potenza AFE":bool, "AFE in marcia":bool}, "Misura corrente diretta WT":bool, "Misura corrente sens ext":bool, "Sens ext abilitati":bool}, "AO non scalati":T11, "AO scalati":T11, "DO (logici)":T12}
  T9 = typedef "ClusterMisura_e_Unità_INPUT.ctl" = cluster{"Misura":dbl, "UM":T10, "Descrizione":string}
  T10 = typedef "UnitàMisura.ctl" = enum16{"V", "mA", "Bar", "RPM", "m3/s", "m3/min", "m3/h", "l/s", "l/min", "in3/min", "ft3/min", "gpm", "igpm", "igph", "%", "°C", "m", "Nm", "A"}
  T11 = typedef "Lista AO sistema.ctl" = cluster{"FRENO1 rif vel":dbl, "FRENO1 rif Coppia":dbl, "FRENO2 rif vel":dbl, "FRENO2 rif Coppia":dbl, "ALIM1 rif V":dbl, "ALIM1 rif F":dbl, "ALIM2 rif V":dbl, "ALIM2 rif F":dbl, "ALIM3 rif V":dbl, "ALIM3 rif F":dbl, "Fnom keb":dbl, "Rpm nom keb":dbl, "Pnom keb":dbl, "Inom keb":dbl, "Vnom keb":dbl, "Rpm max keb":dbl, "Tempo rampa keb":dbl, "Tipo Mot keb":dbl, "FRENO  rif Coppia ":dbl, "FRENO  rif  Corrente":dbl}
  T12 = typedef "DOinterfaccia.ctl" = cluster{"Scelta banco 1":bool, "Scelta banco 2":bool, "Scelta banco 3":bool, "FRENO 1 abilita":bool, "FRENO 1 start":bool, "FRENO 1 senso rotaz":bool, "FRENO 1 ctrl velocità":bool, "FRENO 2 abilita":bool, "FRENO 2 start":bool, "FRENO 2 senso rotaz":bool, "FRENO 2 ctrl velocità":bool, "ALIM 1 abilita":bool, "ALIM 1 start":bool, "ALIM 2 abilita":bool, "ALIM 2 start":bool, "ALIM 3 abilita":bool, "ALIM 3 start":bool, "Abilita linea trifase":bool, "Abilita linea monofase":bool, "Abilita linea dc":bool, "Abilita linea dc eccit":bool, "B1 Linea elettrica 1":bool, "B1 Linea elettrica 2":bool, "B1 Linea elettrica 3":bool, "B1 Linea elettrica 4":bool, "B1 Linea elettrica 5":bool, "B2 Linea elettrica 1":bool, "B2 Linea elettrica 2":bool, "B2 Linea elettrica 3":bool, "B2 Linea elettrica 4":bool, "B2 Linea elettrica 5":bool, "Start potenza AC":bool, "Stop pontenza AC":bool, "Start potenza DC":bool, "Stop potenza DC":bool, "Start potenza eccitaz":bool, "Stop potenza eccitaz":bool, "Reset allarmi":bool, "watchdog":bool, "Scala torsiometro B1":bool, "Controllo torsiom B1":bool, "Scala torsiometro B2":bool, "Controllo torsiom B2":bool, "Teleruttore WT abilita":bool, "Teleruttore Resistomat abilita":bool, "Teleruttore corto fasi":bool, "Ramo 1 resistomat":bool, "Ramo 2 resistomat":bool, "Ramo 3 resistomat":bool, "Collaudo in corso":bool, "Allarme presente":bool, "Enable Res Meter":bool, "Bypass Res Meter":bool, "2nd canale Res Meter":bool, "Scala 200/2000 res meter":bool, "Taratura res meter":bool, "FRENO 1 ctrl coppia":bool, "FRENO 2 ctrl coppia":bool, "FRENO 3 ctrl coppia":bool, "Aggiuntivi impianto":cluster{"Senso rotazione alim 1":bool, "Senso rotazione alim 2":bool}, "ALIM 1 stop":bool, "ALIM 2 stop":bool, "ALIM 3 stop":bool, "FRENO 1 stop":bool, "FRENO 2 stop":bool, "FRENO 3 stop":bool, "B1 configurazione freno B":bool, "B2 configurazione freno B":bool, "Abilita scrittura KEB":bool, "Bench Selection (0-B1,1-B2)":bool, "Select current mode":bool, "Select torque mode":bool, "Select speed mode":bool, "Start":bool, "Stop":bool, "Block":bool, "Enable Force mode":bool, "Abilita linea 125 A":bool, "Abilita linea 63 A":bool, "Abilita linea 16 A":bool, "Aum Tensione Variac":bool, "Dim Tesnione Variac":bool, "Abilita ellectro stractura":bool, "Risprinito Emergence":bool, "Abilita collaudo":bool, "Disabilita collaudo":bool, "External Alaram":bool, "Enable external program":bool, "Reset":bool, "Abilita Ingresso Variac":bool, "Abilita Ventilatore Variac":bool, "Abilita Uscita Variac ":bool}
  T13 = typedef "STATO PLC 1.ctl" = cluster{"USCITE PLC":T14, "Stato DI_PLC":cluster{"Sistema OK":bool, "Rotore bloccato":bool, "Scorta 1":bool, "Prova diretto inverter":bool, "Prova con filtro LC":bool, "Teleruttore WT abilitato":bool, "Alim sinus penta abilitato":bool, "Alim sinus penta in marcia":bool, "Freno abilitato":bool, "Freno in marcia":bool, "Senso rotazione freno":bool, "Potenza abilitata":bool, "Scorta 3":bool, "Scorta 4":bool, "scorta 5":bool, "scorta 6":bool}, "AI plc":cluster{"Allarmi 1":dbl, "Allarmi 2":dbl, "Scorta 1":dbl, "Scorta 2":dbl, "RPM mot prova":dbl, "I mot prova":dbl, "RPM freno":dbl, "I freno":dbl, "Scorta 3":dbl, "Scorta 4":dbl}}
  T14 = typedef "Uscite PLC 1.ctl" = cluster{"AO (real) 2":cluster{"SCORTA 1":dbl, "SCORTA 2":dbl, "SCORTA 3":dbl, "SCORTA 4":dbl, "SCORTA 5":dbl, "SCORTA 6":dbl, "SCORTA 7":dbl, "SCORTA 8":dbl}, "statoAO_PLC out":T15, "DO (bit)":T16}
  T15 = typedef "statoAO_plc_1.ctl" = cluster{"Rif Lim coppia freno [%]":dbl, "Rif rpm freno [%]":dbl, "Rif coppia freno [%]":dbl, "Rif V alimentatore [%]":dbl, "Rif F alimentatore [%]":dbl}
  T16 = typedef "StatoDO_PLC_1.ctl" = cluster{"Scelta banco 1":bool, "Set dati motore freno 2":bool, "Diretto inverter":bool, "Filtro LC":bool, "Marcia ALIM (1s)":bool, "Marcia FRENO (1s)":bool, "Stop AFE (1s)":bool, "Stop freno (1s)":bool, "Reset allarmi":bool, "Watchdog":bool, "Senso rotazione":bool, "Abilita collaudo (1s)":bool, "Disabilita collaudo (1s)":bool, "Abilitazione ALIM":bool, "Abilitazione FRENO":bool, "Teleruttore WT":bool, "Senso rot motore prova":bool, "Scorta 7":bool, "Scorta 8":bool, "Scorta 9":bool, "Scorta 10":bool, "Scorta 11":bool, "Scorta 12":bool, "Scorta 13":bool}
  T17 = typedef "Parametri inverter letti.ctl" = cluster{"Menù Misure motore (M000-M030)":cluster{"Rif vel a regime (int)":u16, "Rif vel a regime (dec)":u16, "Rif vel dopo rampe (int)":u16, "Rif vel dopo rampe (dec)":u16, "RPM motore (int)":u16, "RPM motore (dec)":u16, "FREQout inverter":u16, "Rif coppia a regime(Nm)":u16, "Richiesta di coppia (Nm)":u16, "Coppia generata dal motore(Nm)":u16, "Rif coppia a regime(%)":u16, "Richiesta di coppia (%)":u16, "Coppia generata dal motore(%)":u16, "Coppia max richiesta prima delle rampe(Nm)":u16, "Coppia max richiesta dopo le rampe(Nm)":u16, "Limite di velocità prima delle rampe":u16, "Limite di velocità dopo le rampe":u16, "Coppia max richiesta prima delle rampe(%)":u16, "Coppia max richiesta dopo le rampe(%)":u16, "Rif di flusso":u16, "Corrente di uscita":u16, "Capacità termica del motore":u16, "Tensione di uscita":u16, "Potenza di uscita":u16, "Energia consumata (LSword)":u16, "Energia consumata (MSword)":u16, "Tensione bus DC":u16, "Tensione di rete":u16}, "Menù regolatore PID (M018-M024)":cluster{"Rif PID a regime(%)":u16, "Rif pid dopo rampe(%)":u16, "Retroazione del pid(%)":u16, "Errore del pid(%)":u16, "uscita del pid(%)":u16, "Rif del pid dopo le rampe":u16, "Retroazione del pid":u16}, "Menù ingressi digitali (M031-M036)":cluster{"Ingressi digitali ritardati":u16, "Ingressi digitali istantanei":u16, "Moresettiera comando loc":u16, "Morsett comando da seriale":u16, "Morsett comando bus di campo":u16, "Ing dig ausiliari da morsettiera":u16, "Ing dig ausiliari da seriale":u16}, "Menù riferimenti (M037-M051)":cluster{"Rif analog est REF":u16, "Rif analog est AIN1":u16, "Rif analog est AIN2":u16, "Rif analog est XAIN4":u16, "Rif analog est XAIN5":u16, "Rif velocità da seriale(int)":u16, "Rif velocità bus di campo(int)":u16, "Rif coppia da seriale":u16, "Rif coppia bus di campo":u16, "Rif del PID da seriale":u16, "Rif del PID da bus di campo":u16, "Retroazione del PID da seriale":u16, "Retroazione del PIDda bus di campo":u16, "Rif da encoder":u16, "Rif in frequenza":u16, "Rif velocità da seriale(dec)":u16, "Rif velocità bus di campo(dec)":u16}, "Menù rampe (P009-P033)":cluster{"Tempo di dec rampa di vel 1":u16, "Tempo di acc rampa di vel 2":u16, "Tempo di dec rampa di vel 2":u16, "Tempo di acc rampa di vel 1":u16, "Unità di mis tempi rampe vel 1/2":u16, "Tempo di acc rampa di vel 3":u16, "Tempo di dec rampa di vel 3":u16, "Tempo di acc rampa di vel 4":u16, "Tempo di dec rampa di vel 4":u16, "Unità di mis tempi rampe vel 3/4":u16, "Selettore arrottondam rampe":u16, "Tempo di arrotond iniz rampa acc":u16, "Tempo di arrotond finale rampa acc":u16, "Tempo di arrotond iniz rampa dec":u16, "Tempo di rampa di salita rif coppia":u16, "Tempo di rampa di discesa rif coppia":u16, "Unità di misura rampa coppia":u16, "Tempo rampa acc marcia jog":u16, "Tempo rampa dec marcia jog":u16, "Reset acc ai cambi pendenza":u16, "rampa di acc in fire mode":u16, "rampa di dec in fire mode":u16, "Tempo di arrotond finale rampa dec":u16}, "Menù controllo motore(C008-C128)":cluster{"Numero motori configurati":u16, "Tipo algoritmo di controllo Mot1":u16, "Tipo rif Mot1":u16, "Tensione nominale rete":u16, "Retroaz di vel da encoder Mot1":u16, "Tipo curva V/f Mot1":u16, "Rotazione delle fasi Mot1":u16, "Freq nominale del motore Mot1":u16, "RPM nominali del motore Mot1":u16, "Potenza nominale del motore Mot1":u16, "Corrente nominale del motore Mot1":u16, "Tensione nominale del motore mot1":u16, "Potenza a vuoto del motore Mot1":u16, "Corrente a vuoto del motore Mot1":u16, "Resistenza statorica del motore Mot1":u16, "Induttanza di dispersione Mot1":u16, "Induttanza mutua motore":u16, "Costante di tempo rotorica":u16, "Costante di tempo filtro pb":u16, "Velocità minima motore":u16, "Velocità massima motore":u16}, "Menù configurazione PID":cluster{"Selezione riferimento n.1":u16, "Selezione retroazione n.1":u16, "Modalità di fuzionamento PID":u16, "Termine derivativo calcolato su err o mis":u16, "Proporz moltiplica deriv e integrale":u16, "Azione del PID":u16}, "ID":dbl, "Menù uscite digitali":cluster{"MDO4 Inverter pronto":u16}, "Fcarrier":cluster{"Fcarrier Min (Hz)":u16, "Fcarrier Max (Hz)":u16}, "stato inverter M089":dbl, "Riferimenti":cluster{"Rif tensione":u16, "Rif velocità":u16}, "Comunicazione":bool, "Modalità stop":dbl}
  T18 = typedef "STATO PLC 2.ctl" = cluster{"USCITE PLC":T19, "Stato DI_PLC":cluster{"Sistema ok":bool, "Relè Resistomat abilitato":bool, "Freno abilitato":bool, "Freno in marcia":bool, "scorta b":bool, "scorta a":bool, "scorta 1":bool, "scorta 2":bool, "scorta 3":bool, "scorta 4":bool, "Scorta 5":bool, "Scorta 6":bool, "Scorta 7":bool, "Scorta 8":bool, "Scorta 9":bool, "Scorta 10":bool}, "AI plc":cluster{"Allarmi 1":dbl, "Allarmi 2":dbl, "TC 1":dbl, "TC 2":dbl, "TC 3":dbl, "TC 4":dbl, "TC 5":dbl, "TC 6":dbl, "TC 7":dbl, "TC 8":dbl, "PT1000 1":dbl, "PT1000 2":dbl, "PT1000 3":dbl, "PT1000 4":dbl}}
  T19 = typedef "Uscite PLC 2.ctl" = cluster{"AO (real) 2":cluster{"SCORTA 1":dbl, "SCORTA 2":dbl, "SCORTA 3":dbl, "SCORTA 4":dbl, "SCORTA 5":dbl, "SCORTA 6":dbl, "SCORTA 7":dbl, "SCORTA 8":dbl}, "statoAO_PLC out":T20, "DO (bit)":T21}
  T20 = typedef "statoAO_plc_2.ctl" = cluster{"Condensatori":dbl, "Scorta 1":dbl, "Scorta 2":dbl}
  T21 = typedef "StatoDO_PLC_2.ctl" = cluster{"Relè misura resistomat":bool, "Misura res ramo 1":bool, "Misura res ramo 2":bool, "Misura res ramo 3":bool, "Scelta banco 2":bool, "Scala Torsiometro":bool, "Ctrl torsiometro":bool, "Select current mode":bool, "Select Torque mode":bool, "Select speed mode":bool, "Watchdog":bool, "Scorta":bool, "Scorta 2":bool, "Scorta 3":bool, "Scorta 4":bool, "Scorta 5":bool, "Bench selection":bool, "External alarm":bool, "Enable external program":bool, "Reset allarmi":bool, "Start":bool, "Stop":bool, "Block":bool, "Scorta 6":bool}
  T22 = typedef "STATO PLC 3.ctl" = cluster{"USCITE PLC":T23, "Stato DI_PLC":cluster{"Sistema OK":bool, "Rotore bloccato":bool, "Filtro LC":bool, "Bypass Filtro LC":bool, "Scelta Trasformatore":bool, "Scelta Bypass trasformatore":bool, "Teleruttore wt abilitato":bool, "Alimentatore abilitato":bool, "Alimentatore in marcia":bool, "Scorta 1":bool, "Scorta 2":bool, "Scorta 3":bool, "Potenza abilitata":bool, "Alimentatore in allarme":bool, "Scorta 4":bool, "Conferma dati KEB":bool, "Scorta 5":bool, "Warning Inverter Alimentatore":bool, "Variac Abilitato":bool, "Linea 125 A abilitata":bool, "Linea 63 A abilitata":bool, "Linea 16 A abilitata":bool, "Scorta 6":bool, "Enable force mode":bool}, "AI plc":cluster{"Allarmi 1":dbl, "Allarmi 2":dbl, "RPM motore prova":dbl, "Corrente motore prova":dbl, "RPM freno":dbl, "Corrente freno":dbl, "Tipo motore keb":dbl, "I nom keb":dbl, "RPM nom keb":dbl, "V nom keb":dbl, "F nom keb":dbl, "T rampa keb":dbl, "scorta":dbl, "Scorta 2":dbl}}
  T23 = typedef "Uscite PLC 3.ctl" = cluster{"AO (real) 2":cluster{"SCORTA 1":dbl, "SCORTA 2":dbl, "SCORTA 3":dbl, "SCORTA 4":dbl, "SCORTA 5":dbl, "SCORTA 6":dbl, "SCORTA 7":dbl, "SCORTA 8":dbl}, "statoAO_PLC out":T24, "DO (bit)":T25}
  T24 = typedef "statoAO_plc_3.ctl" = cluster{"Rif velocità alimentatore":dbl, "Scorta":dbl, "Tipo Motore  keb":dbl, "I nom keb":dbl, "RPM nom keb":dbl, "V nom keb":dbl, "F nom keb":dbl, "t rampa keb":dbl}
  T25 = typedef "StatoDO_PLC_3.ctl" = cluster{"Select linea Inverter":bool, "Abilita sense wattmetro":bool, "Bypass filtro LC":bool, "Filtro LC":bool, "Bypass trasformatore":bool, "Trasformatore":bool, "Abilita uscite variac":bool, "Abilita linea 125 A":bool, "Abilita linea 63 A":bool, "Abilita linea 16 A":bool, "Abilita Scrittura Dati Keb":bool, "Abilita alimentatore":bool, "Marcia alimentatore (1s)":bool, "Stop alimentatore (1s)":bool, "Senso rot mot prova":bool, "Watchdog":bool, "Aumenta tensione variac":bool, "Diminuisci tensione variac ":bool, "Blocco elettroserrature":bool, "Ripristino emergence":bool, "Abilita ingresso variac":bool, "Abilita ventilatore variac":bool, "Reset Allarm":bool, "Scorta 1":bool, "Scorta 2":bool, "Scorta 3":bool, "Scorta 4":bool, "Scorta 5":bool, "Scorta 6":bool, "Scorta 7":bool, "Scorta 8":bool, "Scorta 9":bool, "Abilita collaudo":bool, "Disabilita collaudo ":bool, "Scorta 10":bool, "Scorta 11":bool, "Scorta 12":bool, "Scorta 13":bool, "Scorta 14":bool, "Scorta 15":bool}
  T26 = typedef "Parametri DCREG letti.ctl" = cluster{"Parametri di misura":cluster{"M000":dbl, "M001":dbl, "M002":dbl, "M003":dbl, "M004":dbl, "M005":dbl, "M006":dbl, "M007":dbl, "M008":dbl, "M009":dbl, "M010":dbl, "M011":dbl, "M012":dbl, "M013":dbl, "M014":dbl, "M015":dbl, "M016":dbl, "M017":dbl, "M018":dbl, "M019":dbl, "M020":dbl, "M021":dbl, "M022":dbl, "M023":dbl, "M024":dbl, "M025":dbl, "M026":dbl, "M027":dbl, "M028":dbl, "M029":dbl, "M030":dbl, "M031":dbl}, "Parametri di programmazione":cluster{"P000":dbl, "P001":dbl, "P002":dbl, "P003":dbl, "P004":dbl, "P005":dbl, "P006":dbl, "P010":dbl, "P011":dbl, "P012":dbl, "P013":dbl, "P014":dbl, "P015":dbl, "P016":dbl, "P030":dbl, "P031":dbl, "P032":dbl, "P033":dbl, "P034":dbl, "P035":dbl, "P036":dbl, "P037":dbl, "P038":dbl, "P039":dbl, "P040":dbl, "P050":dbl, "P051":dbl, "P052":dbl, "P053":dbl, "P054":dbl, "P055":dbl, "P056":dbl, "P057":dbl, "P058":dbl, "P059":dbl, "P060":dbl, "P061":dbl, "P062":dbl, "P070":dbl, "P071":dbl, "P073":dbl, "P074":dbl, "P076":dbl, "P077":dbl, "P079":dbl, "P080":dbl, "P082":dbl, "P083":dbl, "P084":dbl, "P085":dbl, "P086":dbl, "P087":dbl, "P088":dbl, "P100":dbl, "P101":dbl, "P102":dbl, "P103":dbl, "P104":dbl, "P110":dbl, "P111":dbl, "P120":dbl, "P121":dbl, "P122":dbl, "P123":dbl, "P124":dbl, "P125":dbl, "P126":dbl, "P127":dbl, "P128":dbl, "P129":dbl, "P130":dbl, "P131":dbl, "P132":dbl, "P133":dbl, "P134":dbl, "P150":dbl, "P151":dbl, "P152":dbl, "P153":dbl, "P154":dbl, "P155":dbl, "P156":dbl, "P157":dbl, "P158":dbl, "P170":dbl, "P171":dbl, "P172":dbl, "P173":dbl, "P174":dbl, "P175":dbl, "P176":dbl, "P177":dbl, "P178":dbl, "P179":dbl, "P180":dbl, "P181":dbl, "P182":dbl, "P183":dbl, "P184":dbl, "P185":dbl, "P186":dbl, "P187":dbl, "P188":dbl, "P189":dbl, "P190":dbl, "P191":dbl, "P192":dbl, "P193":dbl, "P194":dbl, "P195":dbl, "P196":dbl, "P197":dbl, "P198":dbl, "P199":dbl, "P211":dbl, "P212":dbl, "P213":dbl, "P214":dbl, "P215":dbl, "P216":dbl, "P217":dbl, "P221":dbl, "P222":dbl, "P223":dbl, "P224":dbl, "P230":dbl, "P231":dbl, "P240":dbl, "P250":dbl, "P251":dbl}, "Parametri di configurazione":cluster{"C000":dbl, "C001":dbl, "C002":dbl, "C010":dbl, "C011":dbl, "C012":dbl, "C014":dbl, "C015":dbl, "C016":dbl, "C017":dbl, "C018":dbl, "C030":dbl, "C050":dbl, "C051":dbl, "C052":dbl, "C060":dbl, "C061":dbl, "C062":dbl, "C063":dbl, "C070":dbl, "C072":dbl, "C074":dbl, "C090":dbl, "C091":dbl, "C092":dbl, "C093":dbl, "C094":dbl, "C100":dbl, "C101":dbl, "C102":dbl, "C103":dbl, "C105":dbl, "C106":dbl, "C107":dbl, "C108":dbl, "C110":dbl, "C111":dbl, "C112":dbl, "C120":dbl, "C121":dbl, "C122":dbl, "C130":dbl, "C131":dbl, "C132":dbl, "C133":dbl, "C134":dbl, "C135":dbl, "C141":dbl, "C142":dbl, "C143":dbl, "C150":dbl, "C151":dbl, "C153":dbl, "C154":dbl, "C155":dbl, "C156":dbl, "C157":dbl, "C158":dbl, "C159":dbl, "C160":dbl, "C161":dbl, "C162":dbl, "C163":dbl, "C164":dbl, "C165":dbl, "C170":dbl}, "Codice allarme":dbl, "Comunicazione":bool}
  T27 = typedef "Cluster MISURE.ctl" = cluster{"MISURE NM":T28, "MISURE ALL":T2}
  T28 = typedef "MISURE NM.ctl" = cluster{"Banco":string, "Anno":string, "Numero":string, "Ntabella":string, "Misura":string, "Tipo Prova":string, "ProgressivoAcq":string, "Descrizione":string, "Data_ora":string, "t. acq [h:m:s]":string, "t. acq [min]":string, "t. acq [s]":string, "n [rpm]":string, "f [Hz]":string, "U1[V]":string, "U2 [V]":string, "U3 [V]":string, "U123_media [V]":string, "I1[A]":string, "I2[A]":string, "I3[A]":string, "I123_media [A]*I":string, "I_123_sbil [%]":string, "Ulin[V]":string, "Uc [V]":string, "Uaux [V]":string, "Ilin[A]*I":string, "Imar[A]":string, "Iaux[A]":string, "Uarm[V]":string, "Uecc[V]":string, "Iarm[A]*I":string, "Iecc[A]":string, "pf":string, "P1 [W]":string, "P1 [kW]":string, "Q [VAR]":string, "Q [kVAR]":string, "S [VA]":string, "S [kVA]":string, "P1arm[W]":string, "P1ecc[W]":string, "Parm[kW]":string, "P1ecc[kW]":string, "Cond[uF]":string, "P1_linea_6fili[W]":string, "P1_linea_6fili[kW]":string, "eta_gr_6fili [%]":string, "eta_inverter_6fili [%]":string, "pf_linea_6fili":string, "U4 [V]":string, "U5 [V]":string, "U6 [V]":string, "U456_media [V]":string, "I4 [A]":string, "I5 [A]":string, "I6 [A]":string, "I456_media [A]":string, "C [Nm]*C":string, "Cric [Nm]":string, "Cric\\Cnom":string, "Iric[A]":string, "Iric\\Inom":string, "P2_mecc [W]":string, "P2_mecc [kW]":string, "eta motore [%]":string, "Scorr[%]":string, "Tamb[°C]":string, "R1[ohm]":string, "R2[ohm]":string, "R3[ohm]":string, "Rmedia[ohm]":string, "DT_R1[°C]":string, "DT_R2[°C]":string, "DT_R3[°C]":string, "DT_media[°C]":string, "R_marcia[ohm]":string, "R_aux[ohm]":string, "DT_marcia[°C]":string, "DT_aux[°C]":string, "R_Arm[ohm]":string, "R_Ecc[ohm]":string, "DT_Arm[°C]":string, "DT_Ecc[°C]":string, "TambFreddo[°C]":string, "R1_freddo[ohm]":string, "R2_freddo[ohm]":string, "R3_freddo[ohm]":string, "Rmedia_freddo[ohm]":string, "R_Marcia_freddo[ohm]":string, "R_Aux_freddo[ohm]":string, "R_Arm_freddo[ohm]":string, "R_Ecc_freddo[ohm]":string, "TC1 [°C]":string, "TC2 [°C]":string, "TC3 [°C]":string, "TC4 [°C]":string, "TC5 [°C]":string, "TC6 [°C]":string, "TC7 [°C]":string, "TC8 [°C]":string, "PT1000_1[°C]":string, "PT1000_2[°C]":string, "PT1000_3[°C]":string, "Vdc eccitatrice[V]":string, "Idc eccitatrice[A]":string, "Vdc rotore[V]":string, "Idc rotore[A]":string, "Vac rotore[V]":string, "Iac rotore[V]":string, "V dinamo[V]":string, "Portata Q":string, "Pressione H":string, "U1'[V]":string, "U2'[V]":string, "U3'[V]":string, "I1'[A]":string, "I2'[A]":string, "I3'[A]":string, "U''R-N":string, "U''S-N":string, "U'' T-N":string, "U''R-S":string, "U''R-T":string, "U''S-T":string, "I1''[A]":string, "I2''[A]":string, "I3''[A]":string, "F''[Hz]":string, "P''[kW]":string, "CosFi''":string, "PT1000_4[°C]":string, "Scorta 3":string}
  T29 = cluster{"Numero":dbl, "Tipo Pompa":dbl, "Costruttore":dbl, "n°serie":dbl, "Tipo Motore":dbl, "Costruttore":dbl, "n°serie":dbl, "Tipologia":dbl, "Tipo Inverter":dbl, "Costruttore":dbl, "n°serie":dbl, "Tipologia":dbl, "Data":dbl, "Nome Cliente":dbl, "Test Engineer":dbl, "Q1 [m3/h]":dbl, "H1 [m]":dbl, "Q2 [m3/h]":dbl, "H2 [m]":dbl, "Qmax [m3/h]":dbl, "Hmax [m]":dbl, "n° giranti":dbl, "MEI":dbl, "EEI":dbl, "IE":dbl, "fn [Hz]":dbl, "Un [V]":dbl, "In [A]":dbl, "P1 [W]":dbl, "P2 [W]":dbl, "Crun [uF]":dbl, "Cstart [uF]":dbl, "Uc [V]":dbl, "Numero Poli":dbl, "n [rpm]":dbl, "Tn [Nm]":dbl, "pfn":dbl, "etp [p.u.]":dbl, "etg [p.u.]":dbl, "C.I.":dbl, "Collegamento":dbl, "Peso [kg]":dbl, "Servizio":dbl, "IP":dbl, "Ru-w [Ohm]":dbl, "Temp0 [°C]":dbl, "DTavv. [°C]":dbl, "DTcassa [°C]":dbl, "IIr [A]":dbl, "TIr [Nm]":dbl, "Note1":dbl, "Note2":dbl, "Note3":dbl, "Note4":dbl, "Dislivello [m]":dbl, "Tubo d1n [DN]":dbl, "Tubo d1 [mm]":dbl, "Tubo1 lungh [mm]":dbl, "Tubo1 rug1":dbl, "Tubo d2n [DN]":dbl, "Tubo d2 [mm]":dbl, "Tubo2 lungh [mm]":dbl, "Tubo2 rug1":dbl, "Cono1 d1 [mm]":dbl, "Cono1 d2 [mm]":dbl, "Cono1 l [mm]":dbl, "Cono2 d1 [mm]":dbl, "Cono2 d2 [mm]":dbl, "Cono2 l [mm]":dbl, "Note5":dbl, "Note6":dbl, "n° giranti":dbl, "D1 girante [mm]":dbl, "B2 girante [mm]":dbl, "materiale":dbl, "tenuta":dbl, "oring":dbl, "mod.girante":dbl, "mod.corpo p":dbl, "Note7":dbl, "Note8":dbl, "Pacco":dbl, "d int. [mm]":dbl, "d est. [mm]":dbl, "d est.rotore[mm]":dbl, "Traferro [mm]":dbl, "Costruzione":dbl, "Note9":dbl, "Note10":dbl, "f mod. [kHz]":dbl, "Mod. Pot. [A]":dbl, "Taglia [W]":dbl, "Tipologia":dbl}
  T30 = typedef "Cluster INFO.ctl" = cluster{"Scelta wattmetro":cluster{"Wattmetro":T31}, "SET RPM":dbl, "SET TEMP":dbl, "Array banchi":T32[], "Array valvole linee avvio/fermata":cluster{"Valvole avvio":cluster{"Set valvole avvio?":bool, "% valvole avvio":dbl[]}, "Valvole fermata":cluster{"Set valvole fermata?":bool, "% valvole fermata":dbl[]}}[], "banco selezionato":i8, "Nomi valvole prop sistema":string[], "canale-- sensore":string[][], "Attriti B1":dbl[][], "Attriti B2":dbl[][], "Collegamento elettrico":cluster{"ALIMENTAZIONE ELETTRICA":T33, "ID":i16, "#rami freddo\\eq term resmeter":i16, "#rami riscaldamento resmeter":i16, "#rami freddo\\eq term resistomat":i16, "#rami riscaldamento resistomat":i16, "CALCOLI":T34}, "lingua":i16, "Costanti collaudo":cluster{"P [bar]":dbl, "T amb. [°C]":dbl, "Umidità [%]":dbl, "T acqua [°C] 2":dbl}, "OPZIONI MISURE RES":cluster{"MISURA A FREDDO":enum16{"NESSUNO", "RESISTOMAT", "RES METER", "ENTRAMBI"}, "MISURA EQ. TERMICO":enum16{"NESSUNO", "RESISTOMAT", "RES METER", "ENTRAMBI"}, "MISURA DT PROVA IN CORSO":enum16{"NESSUNO", "RESISTOMAT - CON FERMATE", "RES METER - CON FERMATE", "RES METER - CONTINUO"}, "MISURE PRIMA E DOPO":enum16{"NESSUNO", "RESISTOMAT", "RES METER"}, "STRUMENTI PRESENTI":enum16{"NESSUNO", "RESISTOMAT", "RES METER", "ENTRAMBI"}}, "Dati targa motore":cluster{"Vnom":dbl, "Fnom":dbl, "Inom":dbl, "Cnom":dbl, "Npoli":dbl, "Scorta 1":dbl, "Scorta 2":dbl, "Scorta 3":dbl}}
  T31 = typedef "WT SELECTION.ctl" = enum32{"No Selection", "WT230", "WT333", "WT1800", "WT330", "VIW", "APLUS"}
  T32 = typedef "Definizione linea.ctl" = cluster{"Nome":string, "Tors. scala1":i32, "Tors. scala2":i32, "rpm":i32, "TAMB":i32, "Indici Temperature":i16[], "Indice freno":i16, "alimentatore trifase":i16, "alimentatore monofase":i16, "alimentatore dc arm":i16, "alimentatore dc ecc":i16, "alimentatore dc mp":i16}
  T33 = typedef "Collegamenti_elettrici.ctl" = enum16{"AC TRIFASE", "AC TRIFASE + FRENO", "AC MONOFASE", "DC CON ECCITAZIONE", "DC CON ECCITAZIONE + FRENO", "DC NO ECCITAZIONE", "DC NO ECCITAZIONE + FRENO", "FRENO TRASC + AFE", "SOLO FRENO", "CARICO RESISTIVO", "GENERICO", "SOLO ACQUISITORE", "SCORTA 4", "SCORTA 5", "SCORTA 6"}
  T34 = typedef "Control Calcoli.ctl" = enum16{"AC TRIFASE", "AC MONOFASE", "DC ECCITAZIONE", "DC NO ECCITAZIONE", "POMPA TRIFASE", "POMPA MONOFASE", "GENERICO", "TRASFORMATORE", "ALTERNATORE TRASCINATO", "GRUPPO ELETTROGENO"}
  T35 = enum32{"Torque [Nm]", "Power [W]", "Speed [RPM]"}
  T36 = cluster{"Coppia compensazione":dbl, "RPM compensazione":dbl}
  T37 = typedef "Stato inverter selezionato.ctl" = cluster{"Stato comandi freno":T38, "Stato":cluster{"rif C%":dbl, "rif vel%":dbl, "Controllo effettivo":enum32{"Torque [Nm]", "Power [W]", "Speed [RPM]"}, "Controllo desiderato":enum32{"Torque [Nm]", "Power [W]", "Speed [RPM]"}, "Fine rampa C":bool, "Fine rampa RPM":bool, "Senso rotaz":bool, "Start":bool, "C stabile":bool, "P stabile":bool, "RPM stabile":bool}}
  T38 = typedef "Comandi freno.ctl" = cluster{"Control":cluster{"Control Type":enum32{"Torque [Nm]", "Power [W]", "Speed [RPM]", "Corrente [A]"}, "Set":dbl, "Inverti senso di rotazione":bool}, "Start\\stop":cluster{"Start":bool, "STOP":bool}, "Status":cluster{"Ready":bool, "Running":bool, "Regulation":bool}, "PID":bool, "Abilita":cluster{"Abilita":bool}, "Status ref":cluster{"Torque":dbl, "Speed":dbl}}
  T39 = typedef "Grandezze banco.ctl" = cluster{"Coppia":dbl, "RPM":dbl, "Tamb":dbl, "Temperature":dbl[]}
  T40 = cluster{"Togli offset":bool, "Offset":dbl, "Scala torsiometro":u16, "SCALA":enum32{"SCALA HIGH", "SCALA LOW", "AUTO"}, "Stato Scala":string}
  T41 = typedef "SET ARRAY DO.ctl" = T42[]
  T42 = typedef "SET SINGLE DO.ctl" = cluster{"DO":T43, "Value":bool}
  T43 = typedef "DO List.ctl" = enum16{"OFF: ALL DO", "*ABILITA freno 1", "*ABILITA freno 2", "*ABILITA freno 3", "*START freno 1", "*START freno 2", "*START freno 3", "*STOP freno 1", "*STOP freno 3", "*STOP freno 2", "*Senso rot freno 1", "*Senso rot freno 2", "*Senso rot freno 3", "*Ctrl velocità freno 1", "*Ctrl velocità freno 2", "*Ctrl velocità freno 3", "*Ctrl coppia freno 1", "*Ctrl coppia freno 2", "*Ctrl coppia freno 3", "*ABILITA alimentatore 1", "*ABILITA alimentatore 2", "*ABILITA alimentatore 3", "*ABILITA alimentatore 4", "*START alimentatore 1", "*START alimentatore 2", "*START alimentatore 3", "*START alimentatore 4", "*STOP alimentatore 1", "*STOP alimentatore 2", "*STOP alimentatore 3", "*STOP alimentatore 4", "SENSO ROT alimentatore 1", "SENSO ROT alimentatore 2", "Abilita LEM 1000A", "Abilita LEM 300A", "Abilita sensori EXT WT", "B1 Seleziona linea 1", "B1 Seleziona linea 2", "B1 Seleziona linea 3", "B1 Seleziona linea 4", "B1 Seleziona linea 5", "B2 Seleziona linea 1", "B2 Seleziona linea 2", "B2 Seleziona linea 3", "B2 Seleziona linea 4", "B2 Seleziona linea 5", "*Reset allarmi", "*Start potenza AC", "*Stop potenza AC", "*Start potenza DC", "*Stop potenza DC", "*Start potenza DC eccit", "*Stop pontenza DC eccit", "Bypass res meter", "2nd canale res meter", "Enable res meter", "*Abilit teler ramo WT", "*Abil teler ramo princ Resit", "*Abil teler ramo 1 Resist", "*Abil teler ramo 2 Resist", "*Abil teler ramo 3 Resist", "*Abil cortocirc avvolgim", "*Controllo torsiometro B1", "*Controllo Torsiom B2", "*Scala torsiometro B1", "*Scala torsiometro B2", "*Collaudo in corso", "*Allarme presente", "Abilitazione elettroserratura", "Exit", "*Abilita collaudo", "*Abilita potenza trifase", "*Abilita potenza monofase", "*Abilita potenza DC", "*Abilita potenza DC eccit", "*Disabilita teleruttori potenza", "Set teleruttori prova a freddo", "Prova a freddo monofase", "Watchdog", "Forza DO PLC 3", "Forza DO PLC 2", "Forza DO PLC 1", "Forza DO cDAQ", "Scala 2000(T) 200(F) res meter", "Seleziona banco 1", "Seleziona banco 2", "Comando azionam in blocco", "Comando azionam reset", "Sensibilità freno 16 32 nm", "Reset Allarmi", "Carico res - Ramo 1", "Carico res - Ramo 2", "Carico res - Ramo 3", "Carico res - Ramo 4", "Carico res - Ramo 5", "Carico res - Ramo 6", "Carico res - Ramo 7", "Carico res - Ramo 8", "Carico res - Ramo 9", "Carico res - Ramo 10", "Carico res - Ramo 11", "Carico res - Start ventilatore", "Carico res - Stop ventilatore", "Abilita potenza solo freno", "Abilita AFE + freno trasc", "Abilita potenza carico resistivo", "Chiudi potenza AFE", "Apri potenza AFE", "Start AFE", "Config Banco2 TDE", "Misura diretto WT", "Ripristina centralina protezioni", "Abilita Scrittura Dati Keb", "Bench Selection(0-B1,1-B2)", "Select current mode", "Select torque mode", "Select speed mode", "Extenal alarm", "Enable Extenal program ", "Start ", "Stop", "Enable force mode", "Abilita linea 125 A", "Abilita linea 63 A", "Abilita linea 16 A", "Aum Tensione Variac", "Dim Tesnione Variac", "Abilita Ellecto Stractura", "Riprinto Emergenxe ", "Abilita Collaudo", "Disabilita Collaudo", "Abilita Ingresso Variac", "Abilita Uscita Variac", "Abilita ventilatore Variac"}
  T44 = typedef "Comandi_Alimentatore.ctl" = cluster{"RIF 1":dbl, "RIF 2":dbl, "Status":cluster{"Ready":bool, "Running":bool, "Regulation":bool}, "Start\\stop":cluster{"Start":bool, "Stop":bool}, "PID RIF1":bool, "PID RIF2":bool, "Status ref":cluster{"RIF 1":dbl, "RIF 2":dbl}, "Abilita":cluster{"Abilita":bool}}
  T45 = cluster{"RIF 1":dbl, "RIF 2":dbl, "Abilitato":bool, "In marcia":bool, "Fine rampa RIF1":bool, "Fine rampa RIF2":bool, "Vstabile":bool, "F stabile":bool, "PID RIF1":bool, "PID RIF2":bool, "Alimentatore 1":T44}
  T46 = enum32{"Torque [Nm]", "Power [W]", "Speed [RPM]", "Corrente [A]"}
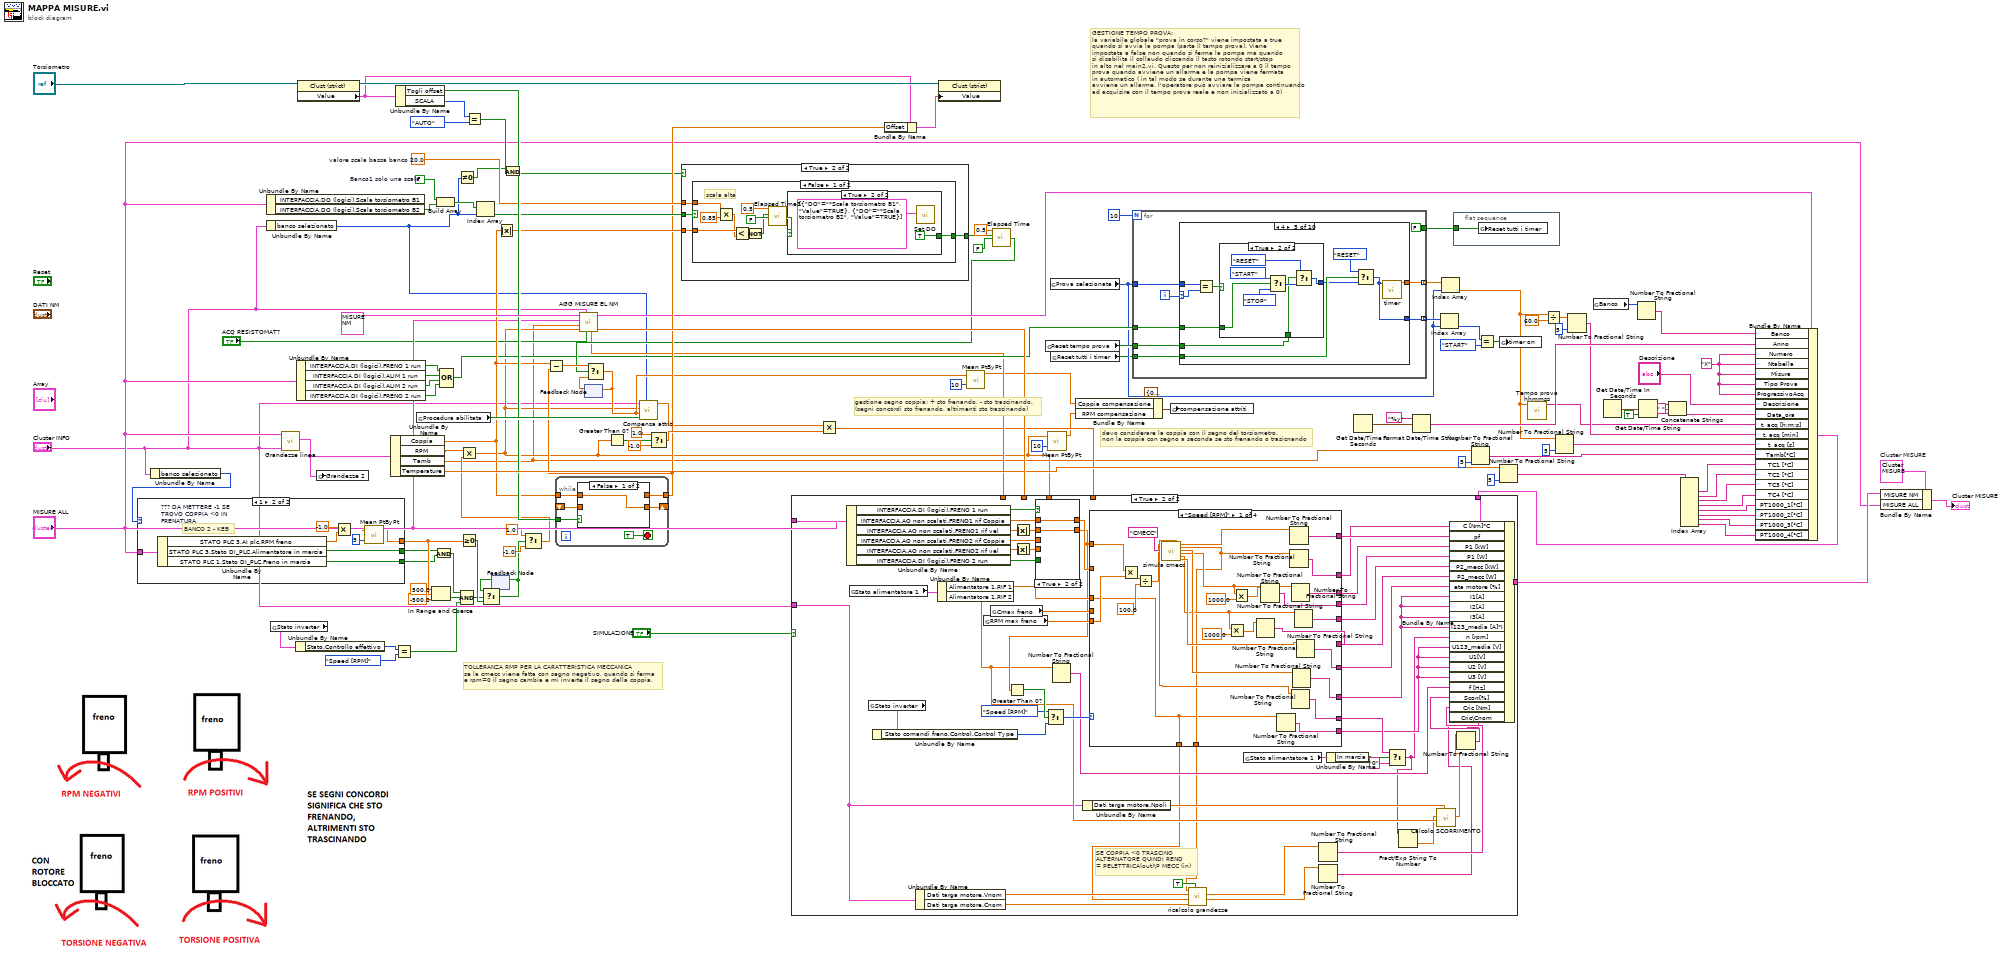
[diagram p0: block diagram]
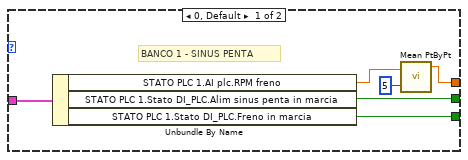
[diagram p2: hidden frame]
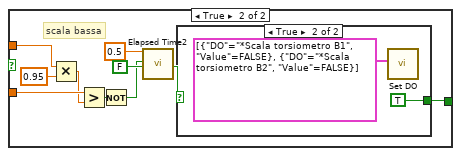
[diagram p5: hidden frame]
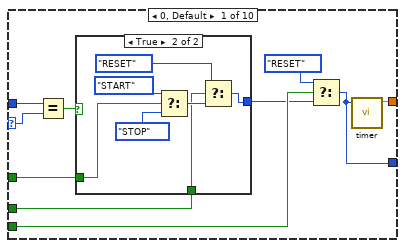
[diagram p8: hidden frame]
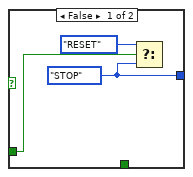
[diagram p9: hidden frame]
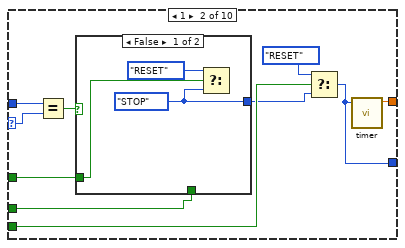
[diagram p10: hidden frame]
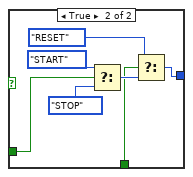
[diagram p11: hidden frame]
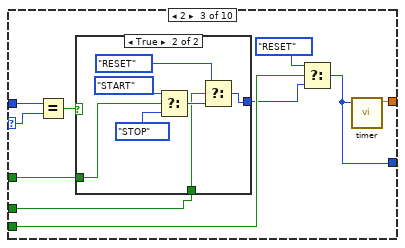
[diagram p12: hidden frame]
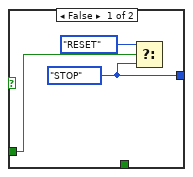
[diagram p13: hidden frame]
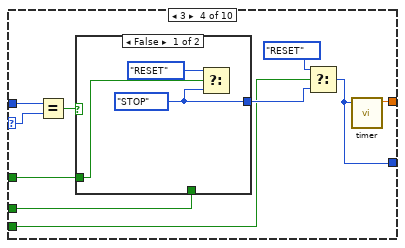
[diagram p14: hidden frame]
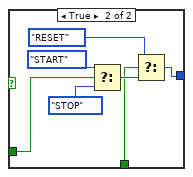
[diagram p15: hidden frame]
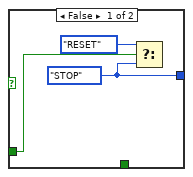
[diagram p16: hidden frame]
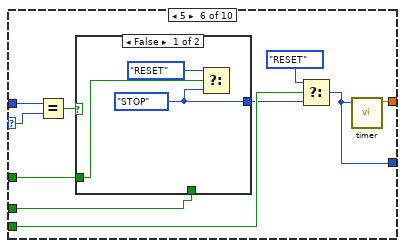
[diagram p17: hidden frame]
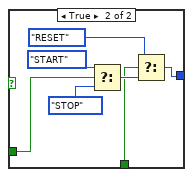
[diagram p18: hidden frame]
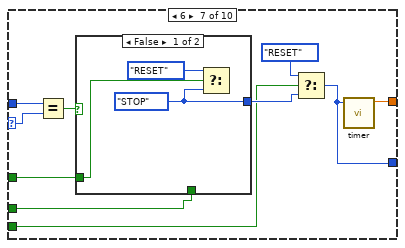
[diagram p19: hidden frame]
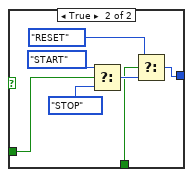
[diagram p20: hidden frame]
diagram:
  w24 = FALSE  # Banco1 solo una scala
  w82 = 10.0  # valore scala bassa banco 2
  w103 = "X" ("Numero")
  w123 = T27 {"MISURE NM"={"Banco"="", "Anno"="", "Numero"="", "Ntabella"="", "Misura"="", "Tipo Prova"="", "ProgressivoAcq"="", "Descrizione"="", "Data_ora"="", "t. acq [h:m:s]"="", "t. acq [min]"="", "t. acq [s]"="", "n [rpm]"="", "f [Hz]"="", "U1[V]"="", "U2 [V]"="", "U3 [V]"="", "U123_media [V]"="", "I1[A]"="", "I2[A]"="", "I3[A]"="", "I123_media [A]*I"="", "I_123_sbil [%]"="", "Ulin[V]"="", "Uc [V]"="", "Uaux [V]"="", "Ilin[A]*I"="", "Imar[A]"="", "Iaux[A]"="", "Uarm[V]"="", "Uecc[V]"="", "Iarm[A]*I"="", "Iecc[A]"="", "pf"="", "P1 [W]"="", "P1 [kW]"="", "Q [VAR]"="", "Q [kVAR]"="", "S [VA]"="", "S [kVA]"="", "P1arm[W]"="", "P1ecc[W]"="", "Parm[kW]"="", "P1ecc[kW]"="", "Cond[uF]"="", "P1_linea_6fili[W]"="", "P1_linea_6fili[kW]"="", "eta_gr_6fili [%]"="", "eta_inverter_6fili [%]"="", "pf_linea_6fili"="", "U4 [V]"="", "U5 [V]"="", "U6 [V]"="", "U456_media [V]"="", "I4 [A]"="", "I5 [A]"="", "I6 [A]"="", "I456_media [A]"="", "C [Nm]*C"="", "Cric [Nm]"="", "Cric\\Cnom"="", "Iric[A]"="", "Iric\\Inom"="", "P2_mecc [W]"="", "P2_mecc [kW]"="", "eta motore [%]"="", "Scorr[%]"="", "Tamb[°C]"="", "R1[ohm]"="", "R2[ohm]"="", "R3[ohm]"="", "Rmedia[ohm]"="", "DT_R1[°C]"="", "DT_R2[°C]"="", "DT_R3[°C]"="", "DT_media[°C]"="", "R_marcia[ohm]"="", "R_aux[ohm]"="", "DT_marcia[°C]"="", "DT_aux[°C]"="", "R_Arm[ohm]"="", "R_Ecc[ohm]"="", "DT_Arm[°C]"="", "DT_Ecc[°C]"="", "TambFreddo[°C]"="", "R1_freddo[ohm]"="", "R2_freddo[ohm]"="", "R3_freddo[ohm]"="", "Rmedia_freddo[ohm]"="", "R_Marcia_freddo[ohm]"="", "R_Aux_freddo[ohm]"="", "R_Arm_freddo[ohm]"="", "R_Ecc_freddo[ohm]"="", "TC1 [°C]"="", "TC2 [°C]"="", "TC3 [°C]"="", "TC4 [°C]"="", "TC5 [°C]"="", "TC6 [°C]"="", "TC7 [°C]"="", "TC8 [°C]"="", "PT1000_1[°C]"="", "PT1000_2[°C]"="", "PT1000_3[°C]"="", "Vdc eccitatrice[V]"="", "Idc eccitatrice[A]"="", "Vdc rotore[V]"="", "Idc rotore[A]"="", "Vac rotore[V]"="", "Iac rotore[V]"="", "V dinamo[V]"="", "Portata Q"="", "Pressione H"="", "U1'[V]"="", "U2'[V]"="", "U3'[V]"="", "I1'[A]"="", "I2'[A]"="", "I3'[A]"="", "U''R-N"="", "U''S-N"="", "U'' T-N"="", "U''R-S"="", "U''R-T"="", "U''S-T"="", "I1''[A]"="", "I2''[A]"="", "I3''[A]"="", "F''[Hz]"="", "P''[kW]"="", "CosFi''"="", "PT1000_4[°C]"="", "Scorta 3"=""}, "MISURE ALL"={"Cluster READ NI"={"AI (0-10V)"={"AI 0"=0.0, "AI 1"=0.0, "AI 2"=0.0, "AI 3"=0.0, "AI 4"=0.0, "AI 5"=0.0, "AI 6"=0.0, "AI 7"=0.0, "AI 8"=0.0, "AI 9"=0.0, "AI 10"=0.0, "AI 11"=0.0, "AI 12"=0.0, "AI 13"=0.0, "AI 14"=0.0, "AI 15"=0.0, "AI 16"=0.0, "AI 17"=0.0, "AI 18"=0.0, "AI 19"=0.0, "AI 20"=0.0, "AI 21"=0.0, "AI 22"=0.0, "AI 23"=0.0, "AI 24"=0.0, "AI 25"=0.0, "AI 26"=0.0, "AI 27"=0.0, "AI 28"=0.0, "AI 29"=0.0, "AI 30"=0.0, "AI 31"=0.0}, "StatoAO_Cdaq[0-10V]"={"AO 1"=0.0, "AO 2"=0.0, "AO 3"=0.0, "AO 4"=0.0}, "Contatori [rpm]"={"RPM 1"=0.0, "RPM 2"=0.0}, "StatoAO_Cdaq [4-20mA]"={"Cdaq_AO [0-10V] 0 for Torque"=0.0, "Cdaq_AO [0-10V] 1"=0.0, "Cdaq_AO [0-10V] 2"=0.0, "Cdaq_AO [0-10V] 3"=0.0}, "StatoDO_Cdaq"={"Scorta 0"=FALSE, "Scorta 1"=FALSE, "Scorta 2"=FALSE, "Scorta 3"=FALSE, "Scorta 4"=FALSE, "Scorta 5"=FALSE, "Scorta 6"=FALSE, "Scorta 7"=FALSE, "Scorta 8"=FALSE, "Scorta 9"=FALSE, "Scorta 10"=FALSE, "Scorta 11"=FALSE, "Scorta 12"=FALSE, "Scorta 13"=FALSE, "Scorta 14"=FALSE, "Scorta 15"=FALSE, "Scorta 16"=FALSE, "Scorta 17"=FALSE, "Scorta 18"=FALSE, "Scorta 19"=FALSE, "Scorta 20"=FALSE, "Scorta 21"=FALSE, "Scorta 22"=FALSE, "Scorta 23"=FALSE, "Scorta 24"=FALSE, "Scorta 25"=FALSE, "Scorta 26"=FALSE, "Scorta 27"=FALSE, "Scorta 28"=FALSE, "Scorta 29"=FALSE, "Scorta 30"=FALSE, "Scorta 31"=FALSE}, "DI"={"Scorta 0"=FALSE, "Scorta 1"=FALSE, "Scorta 2"=FALSE, "Scorta 3"=FALSE, "Scorta 4"=FALSE, "Scorta 5"=FALSE, "Scorta 6"=FALSE, "Scorta 7"=FALSE, "Scorta 8"=FALSE, "Scorta 9"=FALSE, "Scorta 10"=FALSE, "Scorta 11"=FALSE, "Scorta 12"=FALSE, "Scorta 13"=FALSE, "Scorta 14"=FALSE, "Scorta 15"=FALSE, "Scorta 16"=FALSE, "Scorta 17"=FALSE, "Scorta 18"=FALSE, "Scorta 19"=FALSE, "Scorta 20"=FALSE, "Scorta 21"=FALSE, "Scorta 22"=FALSE, "Scorta 23"=FALSE, "Scorta 24"=FALSE, "Scorta 25"=FALSE, "Scorta 26"=FALSE, "Scorta 27"=FALSE, "Scorta 28"=FALSE, "Scorta 29"=FALSE, "Scorta 30"=FALSE, "Scorta 31"=FALSE}, "AI (4-20mA)"={"AI 0"=0.0, "AI 1"=0.0, "AI 2"=0.0, "AI 3"=0.0, "AI 4"=0.0, "AI 5"=0.0, "AI 6"=0.0, "AI 7"=0.0, "AI 8"=0.0, "AI 9"=0.0, "AI 10"=0.0, "AI 11"=0.0, "AI 12"=0.0, "AI 13"=0.0, "AI 14"=0.0, "AI 15"=0.0}, "TC [°C]"={"tc 1"=0.0, "tc 2"=0.0, "tc 3"=0.0, "tc 4"=0.0}, "NI Read Values"={"RPM"=0.0, "Frequency"=0.0, "Mod 1"={"Torsiometro 1"=0.0, "Torsiometro 2"=0.0, "Strin Gauge 1"=0.0, "Strin Gauge 2"=0.0}, "Mod 2"={"Termocoppia 1"=0.0, "Termocoppia 2"=0.0, "Termocoppia 3"=0.0, "Termocoppia 4"=0.0}, "Mod 3"={"PT 100 1"=0.0, "PT 100 2"=0.0, "PT 100 3"=0.0, "PT 100 4"=0.0}}}, "MISURE WT"={"URMS 1"=0.0, "IRMS 1"=0.0, "P 1"=0.0, "S 1"=0.0, "Q 1"=0.0, "LAMBDA 1"=0.0, "PHI 1"=0.0, "F U 1"=0.0, "F I 1"=0.0, "NONE 1"=0.0, "URMS 2"=0.0, "IRMS 2"=0.0, "P 2"=0.0, "S 2"=0.0, "Q 2"=0.0, "LAMBDA 2"=0.0, "PHI 2"=0.0, "F U 2"=0.0, "F I 2"=0.0, "NONE 2"=0.0, "URMS 3"=0.0, "IRMS 3"=0.0, "P 3"=0.0, "S 3"=0.0, "Q 3"=0.0, "LAMBDA 3"=0.0, "PHI 3"=0.0, "F U 3"=0.0, "F I 3"=0.0, "NONE 3"=0.0, "URMS SIGMA"=0.0, "IRMS SIGMA"=0.0, "P SIGMA"=0.0, "S SIGMA"=0.0, "Q SIGMA"=0.0, "LAMBDA SIGMA"=0.0, "PHI SIGMA"=0.0, "F U SIGMA"=0.0, "F I SIGMA"=0.0, "NONE 4"=0.0}, "Resistenze Resistomat"={"Res Ch1"=0.0, "Res Ch2"=0.0, "Res Ch3"=0.0, "Tamb"=0.0}, "INTERFACCIA"={"AI"={"Portate"=[], "Pressioni"=[], "Coppie[Nm]"=[], "Valvole prop %"=[], "RPM"=[], "Livelli"=[], "Temperature"=[], "Riferimenti %"=[], "TENSIONI"=[], "CORRENTI"=[]}, "DI (logici)"={"Start da pulsantiera"=FALSE, "Stop da pulsantiera"=FALSE, "Reset da pulsantiera"=FALSE, "Sistema OK"=FALSE, "Collaudo abilitato"=FALSE, "Potenza trifase abilitata"=FALSE, "Potenza monofase abilitata"=FALSE, "Potenza DC abilitata"=FALSE, "Potenza DC ECC abilitata"=FALSE, "Start alimentazione AC"=FALSE, "Start alimentazione DC"=FALSE, "Start DC eccitazione"=FALSE, "Teleruttore WT abilitato"=FALSE, "Teleruttore Resistomat abilitato"=FALSE, "Teleruttore corto fasi"=FALSE, "Ramo 1 resistomat"=FALSE, "Ramo 2 resistomat"=FALSE, "Ramo 3 resistomat"=FALSE, "B1 Scelta linea elettrica 1"=FALSE, "B1 Scelta linea elettrica 2"=FALSE, "B1 Scelta linea elettrica 3"=FALSE, "B1 Scelta linea elettrica 4"=FALSE, "B1 Scelta linea elettrica 5"=FALSE, "B2 Scelta linea elettrica 1"=FALSE, "B2 Scelta linea elettrica 2"=FALSE, "B2 Scelta linea elettrica 3"=FALSE, "B2 Scelta linea elettrica 4"=FALSE, "B2 Scelta linea elettrica 5"=FALSE, "Rotore bloccato 1"=FALSE, "Rotore bloccato 2"=FALSE, "FRENO 1 abilitato"=FALSE, "FRENO 1 run"=FALSE, "FRENO 1 senso rotaz"=FALSE, "FRENO 1 ctrl velocità"=FALSE, "FRENO 2 abilitato"=FALSE, "FRENO 2 run"=FALSE, "FRENO 2 senso rotaz"=FALSE, "FRENO 2 ctrl velocità"=FALSE, "ALIM 1 abilitato"=FALSE, "ALIM 1 run"=FALSE, "ALIM 2 abilitato"=FALSE, "ALIM 2 run"=FALSE, "ALIM 3 abilitato"=FALSE, "ALIM 3 run"=FALSE, "FRENO 1 ctrl coppia"=FALSE, "FRENO 2 ctrl coppia"=FALSE, "FRENO 3 ctrl coppia"=FALSE, "DI (logici) aggiuntivi impianto"={"Solo freno abilitato"=FALSE, "Carico resistivo abilitato"=FALSE, "AFE+freno abilitato"=FALSE, "Protezioni chiuse"=FALSE, "Start potenza AFE"=FALSE, "AFE in marcia"=FALSE}, "Misura corrente diretta WT"=FALSE, "Misura corrente sens ext"=FALSE, "Sens ext abilitati"=FALSE}, "AO non scalati"={"FRENO1 rif vel"=0.0, "FRENO1 rif Coppia"=0.0, "FRENO2 rif vel"=0.0, "FRENO2 rif Coppia"=0.0, "ALIM1 rif V"=0.0, "ALIM1 rif F"=0.0, "ALIM2 rif V"=0.0, "ALIM2 rif F"=0.0, "ALIM3 rif V"=0.0, "ALIM3 rif F"=0.0, "Fnom keb"=0.0, "Rpm nom keb"=0.0, "Pnom keb"=0.0, "Inom keb"=0.0, "Vnom keb"=0.0, "Rpm max keb"=0.0, "Tempo rampa keb"=0.0, "Tipo Mot keb"=0.0, "FRENO  rif Coppia "=0.0, "FRENO  rif  Corrente"=0.0}, "AO scalati"={"FRENO1 rif vel"=0.0, "FRENO1 rif Coppia"=0.0, "FRENO2 rif vel"=0.0, "FRENO2 rif Coppia"=0.0, "ALIM1 rif V"=0.0, "ALIM1 rif F"=0.0, "ALIM2 rif V"=0.0, "ALIM2 rif F"=0.0, "ALIM3 rif V"=0.0, "ALIM3 rif F"=0.0, "Fnom keb"=0.0, "Rpm nom keb"=0.0, "Pnom keb"=0.0, "Inom keb"=0.0, "Vnom keb"=0.0, "Rpm max keb"=0.0, "Tempo rampa keb"=0.0, "Tipo Mot keb"=0.0, "FRENO  rif Coppia "=0.0, "FRENO  rif  Corrente"=0.0}, "DO (logici)"={"Scelta banco 1"=FALSE, "Scelta banco 2"=FALSE, "Scelta banco 3"=FALSE, "FRENO 1 abilita"=FALSE, "FRENO 1 start"=FALSE, "FRENO 1 senso rotaz"=FALSE, "FRENO 1 ctrl velocità"=FALSE, "FRENO 2 abilita"=FALSE, "FRENO 2 start"=FALSE, "FRENO 2 senso rotaz"=FALSE, "FRENO 2 ctrl velocità"=FALSE, "ALIM 1 abilita"=FALSE, "ALIM 1 start"=FALSE, "ALIM 2 abilita"=FALSE, "ALIM 2 start"=FALSE, "ALIM 3 abilita"=FALSE, "ALIM 3 start"=FALSE, "Abilita linea trifase"=FALSE, "Abilita linea monofase"=FALSE, "Abilita linea dc"=FALSE, "Abilita linea dc eccit"=FALSE, "B1 Linea elettrica 1"=FALSE, "B1 Linea elettrica 2"=FALSE, "B1 Linea elettrica 3"=FALSE, "B1 Linea elettrica 4"=FALSE, "B1 Linea elettrica 5"=FALSE, "B2 Linea elettrica 1"=FALSE, "B2 Linea elettrica 2"=FALSE, "B2 Linea elettrica 3"=FALSE, "B2 Linea elettrica 4"=FALSE, "B2 Linea elettrica 5"=FALSE, "Start potenza AC"=FALSE, "Stop pontenza AC"=FALSE, "Start potenza DC"=FALSE, "Stop potenza DC"=FALSE, "Start potenza eccitaz"=FALSE, "Stop potenza eccitaz"=FALSE, "Reset allarmi"=FALSE, "watchdog"=FALSE, "Scala torsiometro B1"=FALSE, "Controllo torsiom B1"=FALSE, "Scala torsiometro B2"=FALSE, "Controllo torsiom B2"=FALSE, "Teleruttore WT abilita"=FALSE, "Teleruttore Resistomat abilita"=FALSE, "Teleruttore corto fasi"=FALSE, "Ramo 1 resistomat"=FALSE, "Ramo 2 resistomat"=FALSE, "Ramo 3 resistomat"=FALSE, "Collaudo in corso"=FALSE, "Allarme presente"=FALSE, "Enable Res Meter"=FALSE, "Bypass Res Meter"=FALSE, "2nd canale Res Meter"=FALSE, "Scala 200/2000 res meter"=FALSE, "Taratura res meter"=FALSE, "FRENO 1 ctrl coppia"=FALSE, "FRENO 2 ctrl coppia"=FALSE, "FRENO 3 ctrl coppia"=FALSE, "Aggiuntivi impianto"={"Senso rotazione alim 1"=FALSE, "Senso rotazione alim 2"=FALSE}, "ALIM 1 stop"=FALSE, "ALIM 2 stop"=FALSE, "ALIM 3 stop"=FALSE, "FRENO 1 stop"=FALSE, "FRENO 2 stop"=FALSE, "FRENO 3 stop"=FALSE, "B1 configurazione freno B"=FALSE, "B2 configurazione freno B"=FALSE, "Abilita scrittura KEB"=FALSE, "Bench Selection (0-B1,1-B2)"=FALSE, "Select current mode"=FALSE, "Select torque mode"=FALSE, "Select speed mode"=FALSE, "Start"=FALSE, "Stop"=FALSE, "Block"=FALSE, "Enable Force mode"=FALSE, "Abilita linea 125 A"=FALSE, "Abilita linea 63 A"=FALSE, "Abilita linea 16 A"=FALSE, "Aum Tensione Variac"=FALSE, "Dim Tesnione Variac"=FALSE, "Abilita ellectro stractura"=FALSE, "Risprinito Emergence"=FALSE, "Abilita collaudo"=FALSE, "Disabilita collaudo"=FALSE, "External Alaram"=FALSE, "Enable external program"=FALSE, "Reset"=FALSE, "Abilita Ingresso Variac"=FALSE, "Abilita Ventilatore Variac"=FALSE, "Abilita Uscita Variac "=FALSE}}, "FREDDO resistomat"={"Res Ch1"=0.0, "Res Ch2"=0.0, "tAMB"=0.0, "Res Ch3"=0.0}, "STATO PLC 1"={"USCITE PLC"={"AO (real) 2"={"SCORTA 1"=0.0, "SCORTA 2"=0.0, "SCORTA 3"=0.0, "SCORTA 4"=0.0, "SCORTA 5"=0.0, "SCORTA 6"=0.0, "SCORTA 7"=0.0, "SCORTA 8"=0.0}, "statoAO_PLC out"={"Rif Lim coppia freno [%]"=nan, "Rif rpm freno [%]"=nan, "Rif coppia freno [%]"=0.0, "Rif V alimentatore [%]"=0.0, "Rif F alimentatore [%]"=0.0}, "DO (bit)"={"Scelta banco 1"=FALSE, "Set dati motore freno 2"=FALSE, "Diretto inverter"=FALSE, "Filtro LC"=FALSE, "Marcia ALIM (1s)"=FALSE, "Marcia FRENO (1s)"=FALSE, "Stop AFE (1s)"=FALSE, "Stop freno (1s)"=FALSE, "Reset allarmi"=FALSE, "Watchdog"=FALSE, "Senso rotazione"=FALSE, "Abilita collaudo (1s)"=FALSE, "Disabilita collaudo (1s)"=FALSE, "Abilitazione ALIM"=FALSE, "Abilitazione FRENO"=FALSE, "Teleruttore WT"=FALSE, "Senso rot motore prova"=FALSE, "Scorta 7"=FALSE, "Scorta 8"=FALSE, "Scorta 9"=FALSE, "Scorta 10"=FALSE, "Scorta 11"=FALSE, "Scorta 12"=FALSE, "Scorta 13"=FALSE}}, "Stato DI_PLC"={"Sistema OK"=FALSE, "Rotore bloccato"=FALSE, "Scorta 1"=FALSE, "Prova diretto inverter"=FALSE, "Prova con filtro LC"=FALSE, "Teleruttore WT abilitato"=FALSE, "Alim sinus penta abilitato"=FALSE, "Alim sinus penta in marcia"=FALSE, "Freno abilitato"=FALSE, "Freno in marcia"=FALSE, "Senso rotazione freno"=FALSE, "Potenza abilitata"=FALSE, "Scorta 3"=FALSE, "Scorta 4"=FALSE, "scorta 5"=FALSE, "scorta 6"=FALSE}, "AI plc"={"Allarmi 1"=0.0, "Allarmi 2"=0.0, "Scorta 1"=0.0, "Scorta 2"=0.0, "RPM mot prova"=0.0, "I mot prova"=0.0, "RPM freno"=0.0, "I freno"=0.0, "Scorta 3"=0.0, "Scorta 4"=0.0}}, "Res Ch2"=0.0, "Res Ch2 2"=0.0, "FREDDO res meter"={"Res Ch1"=0.0, "Res Ch2"=0.0, "tAMB"=0.0, "Res Ch3"=0.0}, "Resistenze Res Meter"={"Res Ch1"=0.0, "Res Ch2"=0.0, "Res Ch3"=0.0, "Tamb"=0.0}, "READ SINUS PENTA"={"Menù Misure motore (M000-M030)"={"Rif vel a regime (int)"=0, "Rif vel a regime (dec)"=0, "Rif vel dopo rampe (int)"=0, "Rif vel dopo rampe (dec)"=0, "RPM motore (int)"=0, "RPM motore (dec)"=0, "FREQout inverter"=0, "Rif coppia a regime(Nm)"=0, "Richiesta di coppia (Nm)"=0, "Coppia generata dal motore(Nm)"=0, "Rif coppia a regime(%)"=0, "Richiesta di coppia (%)"=0, "Coppia generata dal motore(%)"=0, "Coppia max richiesta prima delle rampe(Nm)"=0, "Coppia max richiesta dopo le rampe(Nm)"=0, "Limite di velocità prima delle rampe"=0, "Limite di velocità dopo le rampe"=0, "Coppia max richiesta prima delle rampe(%)"=0, "Coppia max richiesta dopo le rampe(%)"=0, "Rif di flusso"=0, "Corrente di uscita"=0, "Capacità termica del motore"=0, "Tensione di uscita"=0, "Potenza di uscita"=0, "Energia consumata (LSword)"=0, "Energia consumata (MSword)"=0, "Tensione bus DC"=0, "Tensione di rete"=0}, "Menù regolatore PID (M018-M024)"={"Rif PID a regime(%)"=0, "Rif pid dopo rampe(%)"=0, "Retroazione del pid(%)"=0, "Errore del pid(%)"=0, "uscita del pid(%)"=0, "Rif del pid dopo le rampe"=0, "Retroazione del pid"=0}, "Menù ingressi digitali (M031-M036)"={"Ingressi digitali ritardati"=0, "Ingressi digitali istantanei"=0, "Moresettiera comando loc"=0, "Morsett comando da seriale"=0, "Morsett comando bus di campo"=0, "Ing dig ausiliari da morsettiera"=0, "Ing dig ausiliari da seriale"=0}, "Menù riferimenti (M037-M051)"={"Rif analog est REF"=0, "Rif analog est AIN1"=0, "Rif analog est AIN2"=0, "Rif analog est XAIN4"=0, "Rif analog est XAIN5"=0, "Rif velocità da seriale(int)"=0, "Rif velocità bus di campo(int)"=0, "Rif coppia da seriale"=0, "Rif coppia bus di campo"=0, "Rif del PID da seriale"=0, "Rif del PID da bus di campo"=0, "Retroazione del PID da seriale"=0, "Retroazione del PIDda bus di campo"=0, "Rif da encoder"=0, "Rif in frequenza"=0, "Rif velocità da seriale(dec)"=0, "Rif velocità bus di campo(dec)"=0}, "Menù rampe (P009-P033)"={"Tempo di dec rampa di vel 1"=0, "Tempo di acc rampa di vel 2"=0, "Tempo di dec rampa di vel 2"=0, "Tempo di acc rampa di vel 1"=0, "Unità di mis tempi rampe vel 1/2"=0, "Tempo di acc rampa di vel 3"=0, "Tempo di dec rampa di vel 3"=0, "Tempo di acc rampa di vel 4"=0, "Tempo di dec rampa di vel 4"=0, "Unità di mis tempi rampe vel 3/4"=0, "Selettore arrottondam rampe"=0, "Tempo di arrotond iniz rampa acc"=0, "Tempo di arrotond finale rampa acc"=0, "Tempo di arrotond iniz rampa dec"=0, "Tempo di rampa di salita rif coppia"=0, "Tempo di rampa di discesa rif coppia"=0, "Unità di misura rampa coppia"=0, "Tempo rampa acc marcia jog"=0, "Tempo rampa dec marcia jog"=0, "Reset acc ai cambi pendenza"=0, "rampa di acc in fire mode"=0, "rampa di dec in fire mode"=0, "Tempo di arrotond finale rampa dec"=0}, "Menù controllo motore(C008-C128)"={"Numero motori configurati"=0, "Tipo algoritmo di controllo Mot1"=0, "Tipo rif Mot1"=0, "Tensione nominale rete"=0, "Retroaz di vel da encoder Mot1"=0, "Tipo curva V/f Mot1"=0, "Rotazione delle fasi Mot1"=0, "Freq nominale del motore Mot1"=0, "RPM nominali del motore Mot1"=0, "Potenza nominale del motore Mot1"=0, "Corrente nominale del motore Mot1"=0, "Tensione nominale del motore mot1"=0, "Potenza a vuoto del motore Mot1"=0, "Corrente a vuoto del motore Mot1"=0, "Resistenza statorica del motore Mot1"=0, "Induttanza di dispersione Mot1"=0, "Induttanza mutua motore"=0, "Costante di tempo rotorica"=0, "Costante di tempo filtro pb"=0, "Velocità minima motore"=0, "Velocità massima motore"=0}, "Menù configurazione PID"={"Selezione riferimento n.1"=0, "Selezione retroazione n.1"=0, "Modalità di fuzionamento PID"=0, "Termine derivativo calcolato su err o mis"=0, "Proporz moltiplica deriv e integrale"=0, "Azione del PID"=0}, "ID"=0.0, "Menù uscite digitali"={"MDO4 Inverter pronto"=0}, "Fcarrier"={"Fcarrier Min (Hz)"=0, "Fcarrier Max (Hz)"=0}, "stato inverter M089"=0.0, "Riferimenti"={"Rif tensione"=0, "Rif velocità"=0}, "Comunicazione"=FALSE, "Modalità stop"=0.0}, "STATO PLC 2"={"USCITE PLC"={"AO (real) 2"={"SCORTA 1"=0.0, "SCORTA 2"=0.0, "SCORTA 3"=0.0, "SCORTA 4"=0.0, "SCORTA 5"=0.0, "SCORTA 6"=0.0, "SCORTA 7"=0.0, "SCORTA 8"=0.0}, "statoAO_PLC out"={"Condensatori"=0.0, "Scorta 1"=0.0, "Scorta 2"=0.0}, "DO (bit)"={"Relè misura resistomat"=FALSE, "Misura res ramo 1"=FALSE, "Misura res ramo 2"=FALSE, "Misura res ramo 3"=FALSE, "Scelta banco 2"=FALSE, "Scala Torsiometro"=FALSE, "Ctrl torsiometro"=FALSE, "Select current mode"=FALSE, "Select Torque mode"=FALSE, "Select speed mode"=FALSE, "Watchdog"=FALSE, "Scorta"=FALSE, "Scorta 2"=FALSE, "Scorta 3"=FALSE, "Scorta 4"=FALSE, "Scorta 5"=FALSE, "Bench selection"=FALSE, "External alarm"=FALSE, "Enable external program"=FALSE, "Reset allarmi"=FALSE, "Start"=FALSE, "Stop"=FALSE, "Block"=FALSE, "Scorta 6"=FALSE}}, "Stato DI_PLC"={"Sistema ok"=FALSE, "Relè Resistomat abilitato"=FALSE, "Freno abilitato"=FALSE, "Freno in marcia"=FALSE, "scorta b"=FALSE, "scorta a"=FALSE, "scorta 1"=FALSE, "scorta 2"=FALSE, "scorta 3"=FALSE, "scorta 4"=FALSE, "Scorta 5"=FALSE, "Scorta 6"=FALSE, "Scorta 7"=FALSE, "Scorta 8"=FALSE, "Scorta 9"=FALSE, "Scorta 10"=FALSE}, "AI plc"={"Allarmi 1"=0.0, "Allarmi 2"=0.0, "TC 1"=0.0, "TC 2"=0.0, "TC 3"=0.0, "TC 4"=0.0, "TC 5"=0.0, "TC 6"=0.0, "TC 7"=0.0, "TC 8"=0.0, "PT1000 1"=0.0, "PT1000 2"=0.0, "PT1000 3"=0.0, "PT1000 4"=0.0}}, "STATO PLC 3"={"USCITE PLC"={"AO (real) 2"={"SCORTA 1"=0.0, "SCORTA 2"=0.0, "SCORTA 3"=0.0, "SCORTA 4"=0.0, "SCORTA 5"=0.0, "SCORTA 6"=0.0, "SCORTA 7"=0.0, "SCORTA 8"=0.0}, "statoAO_PLC out"={"Rif velocità alimentatore"=0.0, "Scorta"=0.0, "Tipo Motore  keb"=0.0, "I nom keb"=0.0, "RPM nom keb"=0.0, "V nom keb"=0.0, "F nom keb"=0.0, "t rampa keb"=0.0}, "DO (bit)"={"Select linea Inverter"=FALSE, "Abilita sense wattmetro"=FALSE, "Bypass filtro LC"=FALSE, "Filtro LC"=FALSE, "Bypass trasformatore"=FALSE, "Trasformatore"=FALSE, "Abilita uscite variac"=FALSE, "Abilita linea 125 A"=FALSE, "Abilita linea 63 A"=FALSE, "Abilita linea 16 A"=FALSE, "Abilita Scrittura Dati Keb"=FALSE, "Abilita alimentatore"=FALSE, "Marcia alimentatore (1s)"=FALSE, "Stop alimentatore (1s)"=FALSE, "Senso rot mot prova"=FALSE, "Watchdog"=FALSE, "Aumenta tensione variac"=FALSE, "Diminuisci tensione variac "=FALSE, "Blocco elettroserrature"=FALSE, "Ripristino emergence"=FALSE, "Abilita ingresso variac"=FALSE, "Abilita ventilatore variac"=FALSE, "Reset Allarm"=FALSE, "Scorta 1"=FALSE, "Scorta 2"=FALSE, "Scorta 3"=FALSE, "Scorta 4"=FALSE, "Scorta 5"=FALSE, "Scorta 6"=FALSE, "Scorta 7"=FALSE, "Scorta 8"=FALSE, "Scorta 9"=FALSE, "Abilita collaudo"=FALSE, "Disabilita collaudo "=FALSE, "Scorta 10"=FALSE, "Scorta 11"=FALSE, "Scorta 12"=FALSE, "Scorta 13"=FALSE, "Scorta 14"=FALSE, "Scorta 15"=FALSE}}, "Stato DI_PLC"={"Sistema OK"=FALSE, "Rotore bloccato"=FALSE, "Filtro LC"=FALSE, "Bypass Filtro LC"=FALSE, "Scelta Trasformatore"=FALSE, "Scelta Bypass trasformatore"=FALSE, "Teleruttore wt abilitato"=FALSE, "Alimentatore abilitato"=FALSE, "Alimentatore in marcia"=FALSE, "Scorta 1"=FALSE, "Scorta 2"=FALSE, "Scorta 3"=FALSE, "Potenza abilitata"=FALSE, "Alimentatore in allarme"=FALSE, "Scorta 4"=FALSE, "Conferma dati KEB"=FALSE, "Scorta 5"=FALSE, "Warning Inverter Alimentatore"=FALSE, "Variac Abilitato"=FALSE, "Linea 125 A abilitata"=FALSE, "Linea 63 A abilitata"=FALSE, "Linea 16 A abilitata"=FALSE, "Scorta 6"=FALSE, "Enable force mode"=FALSE}, "AI plc"={"Allarmi 1"=0.0, "Allarmi 2"=0.0, "RPM motore prova"=0.0, "Corrente motore prova"=0.0, "RPM freno"=0.0, "Corrente freno"=0.0, "Tipo motore keb"=0.0, "I nom keb"=0.0, "RPM nom keb"=0.0, "V nom keb"=0.0, "F nom keb"=0.0, "T rampa keb"=0.0, "scorta"=0.0, "Scorta 2"=0.0}}, "DCREG"={"Parametri di misura"={"M000"=0.0, "M001"=0.0, "M002"=0.0, "M003"=0.0, "M004"=0.0, "M005"=0.0, "M006"=0.0, "M007"=0.0, "M008"=0.0, "M009"=0.0, "M010"=0.0, "M011"=0.0, "M012"=0.0, "M013"=0.0, "M014"=0.0, "M015"=0.0, "M016"=0.0, "M017"=0.0, "M018"=0.0, "M019"=0.0, "M020"=0.0, "M021"=0.0, "M022"=0.0, "M023"=0.0, "M024"=0.0, "M025"=0.0, "M026"=0.0, "M027"=0.0, "M028"=0.0, "M029"=0.0, "M030"=0.0, "M031"=0.0}, "Parametri di programmazione"={"P000"=0.0, "P001"=0.0, "P002"=0.0, "P003"=0.0, "P004"=0.0, "P005"=0.0, "P006"=0.0, "P010"=0.0, "P011"=0.0, "P012"=0.0, "P013"=0.0, "P014"=0.0, "P015"=0.0, "P016"=0.0, "P030"=0.0, "P031"=0.0, "P032"=0.0, "P033"=0.0, "P034"=0.0, "P035"=0.0, "P036"=0.0, "P037"=0.0, "P038"=0.0, "P039"=0.0, "P040"=0.0, "P050"=0.0, "P051"=0.0, "P052"=0.0, "P053"=0.0, "P054"=0.0, "P055"=0.0, "P056"=0.0, "P057"=0.0, "P058"=0.0, "P059"=0.0, "P060"=0.0, "P061"=0.0, "P062"=0.0, "P070"=0.0, "P071"=0.0, "P073"=0.0, "P074"=0.0, "P076"=0.0, "P077"=0.0, "P079"=0.0, "P080"=0.0, "P082"=0.0, "P083"=0.0, "P084"=0.0, "P085"=0.0, "P086"=0.0, "P087"=0.0, "P088"=0.0, "P100"=0.0, "P101"=0.0, "P102"=0.0, "P103"=0.0, "P104"=0.0, "P110"=0.0, "P111"=0.0, "P120"=0.0, "P121"=0.0, "P122"=0.0, "P123"=0.0, "P124"=0.0, "P125"=0.0, "P126"=0.0, "P127"=0.0, "P128"=0.0, "P129"=0.0, "P130"=0.0, "P131"=0.0, "P132"=0.0, "P133"=0.0, "P134"=0.0, "P150"=0.0, "P151"=0.0, "P152"=0.0, "P153"=0.0, "P154"=0.0, "P155"=0.0, "P156"=0.0, "P157"=0.0, "P158"=0.0, "P170"=0.0, "P171"=0.0, "P172"=0.0, "P173"=0.0, "P174"=0.0, "P175"=0.0, "P176"=0.0, "P177"=0.0, "P178"=0.0, "P179"=0.0, "P180"=0.0, "P181"=0.0, "P182"=0.0, "P183"=0.0, "P184"=0.0, "P185"=0.0, "P186"=0.0, "P187"=0.0, "P188"=0.0, "P189"=0.0, "P190"=0.0, "P191"=0.0, "P192"=0.0, "P193"=0.0, "P194"=0.0, "P195"=0.0, "P196"=0.0, "P197"=0.0, "P198"=0.0, "P199"=0.0, "P211"=0.0, "P212"=0.0, "P213"=0.0, "P214"=0.0, "P215"=0.0, "P216"=0.0, "P217"=0.0, "P221"=0.0, "P222"=0.0, "P223"=0.0, "P224"=0.0, "P230"=0.0, "P231"=0.0, "P240"=0.0, "P250"=0.0, "P251"=0.0}, "Parametri di configurazione"={"C000"=0.0, "C001"=0.0, "C002"=0.0, "C010"=0.0, "C011"=0.0, "C012"=0.0, "C014"=0.0, "C015"=0.0, "C016"=0.0, "C017"=0.0, "C018"=0.0, "C030"=0.0, "C050"=0.0, "C051"=0.0, "C052"=0.0, "C060"=0.0, "C061"=0.0, "C062"=0.0, "C063"=0.0, "C070"=0.0, "C072"=0.0, "C074"=0.0, "C090"=0.0, "C091"=0.0, "C092"=0.0, "C093"=0.0, "C094"=0.0, "C100"=0.0, "C101"=0.0, "C102"=0.0, "C103"=0.0, "C105"=0.0, "C106"=0.0, "C107"=0.0, "C108"=0.0, "C110"=0.0, "C111"=0.0, "C112"=0.0, "C120"=0.0, "C121"=0.0, "C122"=0.0, "C130"=0.0, "C131"=0.0, "C132"=0.0, "C133"=0.0, "C134"=0.0, "C135"=0.0, "C141"=0.0, "C142"=0.0, "C143"=0.0, "C150"=0.0, "C151"=0.0, "C153"=0.0, "C154"=0.0, "C155"=0.0, "C156"=0.0, "C157"=0.0, "C158"=0.0, "C159"=0.0, "C160"=0.0, "C161"=0.0, "C162"=0.0, "C163"=0.0, "C164"=0.0, "C165"=0.0, "C170"=0.0}, "Codice allarme"=0.0, "Comunicazione"=FALSE}}}  # Cluster MISURE
  # "devo considerare la coppia con il segno del torsiometro, \nnon la coppia con segno a seconda se sto frenando o trasicnando"
  # "gestione segno coppia: + sto frenando, - sto trascinando.\n(segni concordi sto frenando, altrimenti sto trascinando)"
  # "TOLLERANZA RMP PER LA CARATTERISTICA MECCANICA\nse la cmecc viene fatta con segno negativo, quando si ferma\ne rpm=0 il segno cambia e mi inverte il segno della coppia."
  # "GESTIONE TEMPO PROVA:\nla variabile globale \"prova in corso?\" viene impostata a true\nquando si avvia la pompa (parte il tempo prova). Viene \nimpostata a false non quando si ferma la pompa ma quando\nsi disabilita il collaudo cliccando il tasto rotondo start/stop\nin alto nel main2.vi. Questo per non reinizializzare a 0 il tempo\nprova quando avviene un allarme e la pompa viene fermata \nin automatico ( in tal modo se durante una termica\navviene un allarme, l'operatore può avviare la pompa continuando\nad acquisire con il tempo prova reale e non inizializzato a 0)"
  n1 = Unbundle By Name("Cluster INFO") -> ("banco selezionato"=w16:i8)
  n2 = case shown="1" w16 {
    tunnel: "MISURE ALL" -> [w129 w137]
    tunnel: [w124 w130] -> w38
    tunnel: [w128 w136] -> w36
    tunnel: [w127 w135] -> w35
    frame 0, Default {
      # "BANCO 1 - SINUS PENTA"
      n3 = Unbundle By Name(w129) -> ("STATO PLC 1.AI plc.RPM freno"=w125:dbl, "STATO PLC 1.Stato DI_PLC.Alim sinus penta in marcia"=w128:bool, "STATO PLC 1.Stato DI_PLC.Freno in marcia"=w127:bool)
      n4 = call <vilib>:"Mean PtByPt.vi"("x"=w125, "sample length"=5) -> ("mean"=w124:dbl)  [unwired: 2 in, 1 out]
    }
    frame 1 {
      w133 = -1.0  # ??? DA METTERE -1 SE TROVO COPPIA <0 IN FRENATURA
      # "BANCO 2 - KEB"
      n5 = Unbundle By Name(w137) -> ("STATO PLC 3.AI plc.RPM freno"=w134:dbl, "STATO PLC 3.Stato DI_PLC.Alimentatore in marcia"=w136:bool, "STATO PLC 1.Stato DI_PLC.Freno in marcia"=w135:bool)
      n6 = Multiply(x=w133, y=w134) -> (x*y=w131:dbl)
      n7 = call <vilib>:"Mean PtByPt.vi"("x"=w131, "sample length"=5) -> ("mean"=w130:dbl)  [unwired: 2 in, 1 out]
    }
  }
  n8 = Unbundle By Name("MISURE ALL") -> ("INTERFACCIA.DO (logici).Scala torsiometro B2"=w85:bool)  [unwired: 1 out]
  n9 = Unbundle By Name("Cluster INFO") -> ("banco selezionato"=w23:i8)
  n10 = global read "Stato comandi freno.vi" "Stato inverter"() -> (w13:T37)
  n11 = call "Grandezze linea.vi"("Cluster INFO"="Cluster INFO", "MISURE ALL"="MISURE ALL") -> ("Grandezze"=w120:T39)  [unwired: 9 in]
  n12 = Unbundle By Name(w13) -> ("Stato.Controllo effettivo"=w12:T35)
  n13 = Unbundle By Name("MISURE ALL") -> ("INTERFACCIA.DI (logici).FRENO 1 run"=w61:bool, "INTERFACCIA.DI (logici).ALIM 1 run"=w62:bool, "INTERFACCIA.DI (logici).ALIM 2 run"=w15:bool, "INTERFACCIA.DI (logici).FRENO 2 run"=w14:bool)
  n14 = property class="Clust (strict)"(reference="Torsiometro") -> (reference out=w80:refnum<vi>, "Value"=w79:T40)  [unwired: 1 in, 1 out]
  n15 = global write "Global grandezze linea.vi" "Grandezze 2"(w120) -> ()
  n16 = Unbundle By Name(w120) -> ("Coppia"=w64:dbl, "RPM"=w72:dbl, "Tamb"=w19:dbl, "Temperature"=w93:dbl[])
  n17 = Equal?(x=w12, y=T35."Speed [RPM]" ("Stato.Controllo effettivo")) -> (x = y?=w10:bool)
  n18 = Unbundle By Name(w79) -> ("Togli offset"=w87:bool, "SCALA"=w81:enum32{"SCALA HIGH", "SCALA LOW", "AUTO"})
  n19 = global read "Global procedura abilitata.vi" "Procedura abilitata"() -> (w119:bool)
  n20 = In Range and Coerce(upper limit=500.0, x=w38, lower limit=-500.0) -> (In Range?=w44:bool)  [unwired: 1 out]
  n21 = And(x=w36, y=w35) -> (x .and. y?=w39:bool)
  n22 = Build Array(w24, w85) -> (w84:bool[])
  n23 = Compound Arithmetic op=OR(w61, w62, w15, w14) -> (w58:bool)
  n24 = Not Equal To 0?(x=w23) -> (x != 0?=w21:bool)
  n25 = Greater Or Equal To 0?(x=w38) -> (x >= 0?=w43:bool)
  n26 = Compound Arithmetic op=AND(w39, w44, w10) -> (w40:bool)
  n27 = Equal?(x=w81, y=enum32{"SCALA HIGH", "SCALA LOW", "AUTO"}."AUTO") -> (x = y?=w86:bool)
  n28 = Index Array(array=w84, index=w23) -> (element=w83:bool)
  n29 = feedback #1() -> (w41:bool)  [unwired: 1 in]
  n30 = Select(t=w41, s=w40, f=w43) -> (s? t:f=w42:bool)
  n31 = feedback-in #1(w42) -> ()
  n32 = Absolute Value(x=w64) -> (abs(x)=w71:dbl)
  n33 = And(x=w21, y=w86) -> (x .and. y?=w22:bool)
  n34 = Select(t=1.0, s=w42, f=-1.0) -> (s? t:f=w37:dbl)
  n35 = Multiply(x=w72, y=w37) -> (x*y=w26:dbl)
  n36 = while {
    shift-right: [w141] -> _
    shift-left: _ -> [w142]
    tunnel: w64 -> [w140]
    tunnel: w87 -> [w143]
    tunnel: [w138] -> w65
    stop <- TRUE stop-if-true
    n37 = case shown="False" w143 {
      tunnel: w142 -> [_ w145]
      tunnel: [w144 w145] -> w141
      tunnel: w140 -> [w144 _]
      tunnel: [_ w145] -> w138
      frame False {
      }
      frame True {
      }
    }
  }
  n38 = Subtract(x=w64, y=w65) -> (x-y=w66:dbl)
  n39 = call "AGG MISURE EL NM.vi"("ACQ RESISTOMAT?"="ACQ RESISTOMAT?", "Cluster INFO"="Cluster INFO", "RPM"=w26, "tamb"=w19, "MISURE ALL"="MISURE ALL", "MISURE NM in"=T28 {"Banco"="", "Anno"="", "Numero"="", "Ntabella"="", "Misura"="", "Tipo Prova"="", "ProgressivoAcq"="", "Descrizione"="", "Data_ora"="", "t. acq [h:m:s]"="", "t. acq [min]"="", "t. acq [s]"="", "n [rpm]"="", "f [Hz]"="", "U1[V]"="", "U2 [V]"="", "U3 [V]"="", "U123_media [V]"="", "I1[A]"="", "I2[A]"="", "I3[A]"="", "I123_media [A]*I"="", "I_123_sbil [%]"="", "Ulin[V]"="", "Uc [V]"="", "Uaux [V]"="", "Ilin[A]*I"="", "Imar[A]"="", "Iaux[A]"="", "Uarm[V]"="", "Uecc[V]"="", "Iarm[A]*I"="", "Iecc[A]"="", "pf"="", "P1 [W]"="", "P1 [kW]"="", "Q [VAR]"="", "Q [kVAR]"="", "S [VA]"="", "S [kVA]"="", "P1arm[W]"="", "P1ecc[W]"="", "Parm[kW]"="", "P1ecc[kW]"="", "Cond[uF]"="", "P1_linea_6fili[W]"="", "P1_linea_6fili[kW]"="", "eta_gr_6fili [%]"="", "eta_inverter_6fili [%]"="", "pf_linea_6fili"="", "U4 [V]"="", "U5 [V]"="", "U6 [V]"="", "U456_media [V]"="", "I4 [A]"="", "I5 [A]"="", "I6 [A]"="", "I456_media [A]"="", "C [Nm]*C"="", "Cric [Nm]"="", "Cric\\Cnom"="", "Iric[A]"="", "Iric\\Inom"="", "P2_mecc [W]"="", "P2_mecc [kW]"="", "eta motore [%]"="", "Scorr[%]"="", "Tamb[°C]"="", "R1[ohm]"="", "R2[ohm]"="", "R3[ohm]"="", "Rmedia[ohm]"="", "DT_R1[°C]"="", "DT_R2[°C]"="", "DT_R3[°C]"="", "DT_media[°C]"="", "R_marcia[ohm]"="", "R_aux[ohm]"="", "DT_marcia[°C]"="", "DT_aux[°C]"="", "R_Arm[ohm]"="", "R_Ecc[ohm]"="", "DT_Arm[°C]"="", "DT_Ecc[°C]"="", "TambFreddo[°C]"="", "R1_freddo[ohm]"="", "R2_freddo[ohm]"="", "R3_freddo[ohm]"="", "Rmedia_freddo[ohm]"="", "R_Marcia_freddo[ohm]"="", "R_Aux_freddo[ohm]"="", "R_Arm_freddo[ohm]"="", "R_Ecc_freddo[ohm]"="", "TC1 [°C]"="", "TC2 [°C]"="", "TC3 [°C]"="", "TC4 [°C]"="", "TC5 [°C]"="", "TC6 [°C]"="", "TC7 [°C]"="", "TC8 [°C]"="", "PT1000_1[°C]"="", "PT1000_2[°C]"="", "PT1000_3[°C]"="", "Vdc eccitatrice[V]"="", "Idc eccitatrice[A]"="", "Vdc rotore[V]"="", "Idc rotore[A]"="", "Vac rotore[V]"="", "Iac rotore[V]"="", "V dinamo[V]"="", "Portata Q"="", "Pressione H"="", "U1'[V]"="", "U2'[V]"="", "U3'[V]"="", "I1'[A]"="", "I2'[A]"="", "I3'[A]"="", "U''R-N"="", "U''S-N"="", "U'' T-N"="", "U''R-S"="", "U''R-T"="", "U''S-T"="", "I1''[A]"="", "I2''[A]"="", "I3''[A]"="", "F''[Hz]"="", "P''[kW]"="", "CosFi''"="", "PT1000_4[°C]"="", "Scorta 3"=""} ("MISURE NM")) -> ("V"=w96:dbl, "MISURE NM out"=w60:T28, "P1[W]"=w57:dbl)  [unwired: 3 in]
  n40 = feedback #2() -> (w73:dbl)  [unwired: 1 in]
  n41 = Greater Than 0?(x=w26) -> (x > 0?=w70:bool)
  n42 = Select(t=1.0 ("y"), s=w70, f=-1.0) -> (s? t:f=w68:dbl)
  n43 = case shown="True" w22 {
    tunnel: w71 -> [_ w148]
    tunnel: w83 -> [_ w149]
    tunnel: w82 -> [_ w147]
    tunnel: [_ w146] -> w75
    frame False {
    }
    frame True {
      n44 = case shown="False" w149 {
        tunnel: w148 -> [w159 w171]
        tunnel: w147 -> [w158 w170]
        tunnel: [w155 w167] -> w146
        frame False {
          # "scala alta"
          n45 = Multiply(x=w158, y=0.85) -> (x*y=w156:dbl)
          n46 = Less?(x=w159, y=w156) -> (x < y?=w152:bool)
          n47 = Not(x=w152) -> (.not. x?=w150:bool)
          n48 = call "Elapsed Time3"("Time Target (s)"=0.5, "Reset"=w150, "Auto Reset"=FALSE) -> ("Time has Elapsed"=w151:bool)  [unwired: 9 in, 7 out]
          n49 = case shown="True" w151 {
            tunnel: [_ TRUE] -> w155
            frame False {
            }
            frame True {
              n50 = call "Set DO.vi"("Cluster SET DO"=T41 [{"DO"=enum."*Scala torsiometro B1", "Value"=TRUE}, {"DO"=enum."*Scala torsiometro B2", "Value"=TRUE}]) -> ()  [unwired: 10 in, 1 out]
            }
          }
        }
        frame True {
          # "scala bassa"
          n51 = Multiply(x=w170, y=0.95) -> (x*y=w168:dbl)
          n52 = Greater?(x=w171, y=w168) -> (0:w164:bool)
          n53 = Not(x=w164) -> (.not. x?=w162:bool)
          n54 = call "Elapsed Time2"("Time Target (s)"=0.5, "Reset"=w162, "Auto Reset"=FALSE) -> ("Time has Elapsed"=w163:bool)  [unwired: 9 in, 7 out]
          n55 = case shown="True" w163 {
            tunnel: [_ TRUE] -> w167
            frame False {
            }
            frame True {
              n56 = call "Set DO.vi"("Cluster SET DO"=T41 [{"DO"=enum."*Scala torsiometro B1", "Value"=FALSE}, {"DO"=enum."*Scala torsiometro B2", "Value"=FALSE}]) -> ()  [unwired: 10 in, 1 out]
            }
          }
        }
      }
    }
  }
  n57 = Bundle By Name(cluster=w79, "Offset"=w65) -> (w78:T40)
  n58 = property class="Clust (strict)"(reference=w80, "Value"=w78) -> ()  [unwired: 1 in, 2 out]
  n59 = call "Elapsed Time"("Time Target (s)"=0.5, "Reset"=w75, "Auto Reset"=FALSE) -> ("Time has Elapsed"=w59:bool)  [unwired: 9 in, 7 out]
  n60 = Select(t=w66, s=w59, f=w73) -> (s? t:f=w29:dbl)
  n61 = feedback-in #2(w29) -> ()
  n62 = call "Compensa attriti.vi"("BANCO"=w23, "Procedura abilitata?"=w119, "C[Nm] in"=w29, "rpm"=w26, "Cluster INFO"="Cluster INFO") -> ("C[Nm] out"=w34:dbl)  [unwired: 6 in]
  n63 = Multiply(x=w34, y=w68) -> (x*y=w33:dbl)
  n64 = call <vilib>:"Mean PtByPt.vi"("x"=w29, "sample length"=10) -> ("mean"=w28:dbl)  [unwired: 2 in, 1 out]
  n65 = global read "Global prova in corso.vi" "Reset tempo prova"() -> (w89:bool)
  n66 = call <vilib>:"Mean PtByPt.vi"("x"=w26, "sample length"=10) -> ("mean"=w25:dbl)  [unwired: 2 in, 1 out]
  n67 = global read "Prova selezionata.vi" "Prova selezionata"() -> (w54:i16)
  n68 = global read "Global prova in corso.vi" "Reset tutti i timer"() -> (w50:bool)
  n69 = Bundle By Name(cluster=T36 {"Coppia compensazione"=0.0, "RPM compensazione"=0.0} ("compensazione attriti"), "Coppia compensazione"=w28, "RPM compensazione"=w25) -> (w31:T36)
  n70 = for {
    N: 10 -> [_]
    tunnel: [w181] -> w91 mode=indexing
    tunnel: w54 -> [w180]
    tunnel: w58 -> [w178]
    tunnel: w89 -> [w177]
    tunnel: [w176] -> w55 mode=indexing
    tunnel: w50 -> [w175]
    tunnel: [FALSE ("Reset tutti i timer")] -> w49
    i -> [w179]
    n71 = case shown="4" w179 {
      selector: w179 -> [w188 w208 w228 w248 w268 w288 w308 w328 w348 w368]
      tunnel: [w191 w211 w231 w251 w271 w291 w311 w331 w351 w371] -> w181
      tunnel: w180 -> [w190 w210 w230 w250 w270 w290 w310 w330 w350 w370]
      tunnel: w178 -> [w187 w207 w227 w247 w267 w287 w307 w327 w347 w367]
      tunnel: w177 -> [w186 w206 w226 w246 w266 w286 w306 w326 w346 w366]
      tunnel: [w182 w202 w222 w243 w262 w282 w303 w322 w342 w362] -> w176
      tunnel: w175 -> [w185 w204 w224 w242 w264 w284 w302 w324 w344 w364]
      frame 0, Default {
        n72 = Equal?(x=w190, y=w188) -> (x = y?=w189:bool)
        n73 = case shown="True" w189 {
          tunnel: [w192 w197] -> w184
          tunnel: w187 -> [w194 w201]
          tunnel: w186 -> [_ w195]
          frame False {
            w192 = enum32{"START", "STOP", "RESET", "RIPRENDI"}."STOP" ("Azione")
            n74 = Select(t=enum32{"START", "STOP", "RESET", "RIPRENDI"}."RESET", s=w194, f=w192) -> ()  [unwired: 1 out]
          }
          frame True {
            n75 = Select(t=enum32{"START", "STOP", "RESET", "RIPRENDI"}."START" ("Azione"), s=w201, f=enum32{"START", "STOP", "RESET", "RIPRENDI"}."STOP" ("Azione")) -> (s? t:f=w198:enum32{"START", "STOP", "RESET", "RIPRENDI"})
            n76 = Select(t=enum32{"START", "STOP", "RESET", "RIPRENDI"}."RESET", s=w195, f=w198) -> (s? t:f=w197:enum32{"START", "STOP", "RESET", "RIPRENDI"})
          }
        }
        n77 = Select(t=enum32{"START", "STOP", "RESET", "RIPRENDI"}."RESET", s=w185, f=w184) -> (s? t:f=w182:enum32{"START", "STOP", "RESET", "RIPRENDI"})
        n78 = call "timer.vi"("Azione"=w182) -> ("f"=w191:dbl)  [unwired: 10 in]
      }
      frame 1 {
        n79 = Equal?(x=w210, y=w208) -> (x = y?=w209:bool)
        n80 = case shown="False" w209 {
          tunnel: [w212 w217] -> w203
          tunnel: w207 -> [w214 w221]
          tunnel: w206 -> [_ w215]
          frame False {
            w212 = enum32{"START", "STOP", "RESET", "RIPRENDI"}."STOP" ("Azione")
            n81 = Select(t=enum32{"START", "STOP", "RESET", "RIPRENDI"}."RESET", s=w214, f=w212) -> ()  [unwired: 1 out]
          }
          frame True {
            n82 = Select(t=enum32{"START", "STOP", "RESET", "RIPRENDI"}."START" ("Azione"), s=w221, f=enum32{"START", "STOP", "RESET", "RIPRENDI"}."STOP" ("Azione")) -> (s? t:f=w218:enum32{"START", "STOP", "RESET", "RIPRENDI"})
            n83 = Select(t=enum32{"START", "STOP", "RESET", "RIPRENDI"}."RESET", s=w215, f=w218) -> (s? t:f=w217:enum32{"START", "STOP", "RESET", "RIPRENDI"})
          }
        }
        n84 = Select(t=enum32{"START", "STOP", "RESET", "RIPRENDI"}."RESET", s=w204, f=w203) -> (s? t:f=w202:enum32{"START", "STOP", "RESET", "RIPRENDI"})
        n85 = call "timer.vi"("Azione"=w202) -> ("f"=w211:dbl)  [unwired: 10 in]
      }
      frame 2 {
        n86 = Equal?(x=w230, y=w228) -> (x = y?=w229:bool)
        n87 = case shown="True" w229 {
          tunnel: [w232 w237] -> w223
          tunnel: w227 -> [w234 w241]
          tunnel: w226 -> [_ w235]
          frame False {
            w232 = enum32{"START", "STOP", "RESET", "RIPRENDI"}."STOP" ("Azione")
            n88 = Select(t=enum32{"START", "STOP", "RESET", "RIPRENDI"}."RESET", s=w234, f=w232) -> ()  [unwired: 1 out]
          }
          frame True {
            n89 = Select(t=enum32{"START", "STOP", "RESET", "RIPRENDI"}."START" ("Azione"), s=w241, f=enum32{"START", "STOP", "RESET", "RIPRENDI"}."STOP" ("Azione")) -> (s? t:f=w238:enum32{"START", "STOP", "RESET", "RIPRENDI"})
            n90 = Select(t=enum32{"START", "STOP", "RESET", "RIPRENDI"}."RESET", s=w235, f=w238) -> (s? t:f=w237:enum32{"START", "STOP", "RESET", "RIPRENDI"})
          }
        }
        n91 = Select(t=enum32{"START", "STOP", "RESET", "RIPRENDI"}."RESET", s=w224, f=w223) -> (s? t:f=w222:enum32{"START", "STOP", "RESET", "RIPRENDI"})
        n92 = call "timer.vi"("Azione"=w222) -> ("f"=w231:dbl)  [unwired: 10 in]
      }
      frame 3 {
        n93 = Equal?(x=w250, y=w248) -> (x = y?=w249:bool)
        n94 = case shown="False" w249 {
          tunnel: [w252 w257] -> w244
          tunnel: w247 -> [w254 w261]
          tunnel: w246 -> [_ w255]
          frame False {
            w252 = enum32{"START", "STOP", "RESET", "RIPRENDI"}."STOP" ("Azione")
            n95 = Select(t=enum32{"START", "STOP", "RESET", "RIPRENDI"}."RESET", s=w254, f=w252) -> ()  [unwired: 1 out]
          }
          frame True {
            n96 = Select(t=enum32{"START", "STOP", "RESET", "RIPRENDI"}."START" ("Azione"), s=w261, f=enum32{"START", "STOP", "RESET", "RIPRENDI"}."STOP" ("Azione")) -> (s? t:f=w258:enum32{"START", "STOP", "RESET", "RIPRENDI"})
            n97 = Select(t=enum32{"START", "STOP", "RESET", "RIPRENDI"}."RESET", s=w255, f=w258) -> (s? t:f=w257:enum32{"START", "STOP", "RESET", "RIPRENDI"})
          }
        }
        n98 = Select(t=enum32{"START", "STOP", "RESET", "RIPRENDI"}."RESET", s=w242, f=w244) -> (s? t:f=w243:enum32{"START", "STOP", "RESET", "RIPRENDI"})
        n99 = call "timer.vi"("Azione"=w243) -> ("f"=w251:dbl)  [unwired: 10 in]
      }
      frame 4 {
        n100 = Equal?(x=w270, y=w268) -> (x = y?=w269:bool)
        n101 = case shown="True" w269 {
          tunnel: [w272 w277] -> w263
          tunnel: w267 -> [w274 w281]
          tunnel: w266 -> [_ w275]
          frame False {
            w272 = enum32{"START", "STOP", "RESET", "RIPRENDI"}."STOP" ("Azione")
            n102 = Select(t=enum32{"START", "STOP", "RESET", "RIPRENDI"}."RESET", s=w274, f=w272) -> ()  [unwired: 1 out]
          }
          frame True {
            n103 = Select(t=enum32{"START", "STOP", "RESET", "RIPRENDI"}."START" ("Azione"), s=w281, f=enum32{"START", "STOP", "RESET", "RIPRENDI"}."STOP" ("Azione")) -> (s? t:f=w278:enum32{"START", "STOP", "RESET", "RIPRENDI"})
            n104 = Select(t=enum32{"START", "STOP", "RESET", "RIPRENDI"}."RESET", s=w275, f=w278) -> (s? t:f=w277:enum32{"START", "STOP", "RESET", "RIPRENDI"})
          }
        }
        n105 = Select(t=enum32{"START", "STOP", "RESET", "RIPRENDI"}."RESET", s=w264, f=w263) -> (s? t:f=w262:enum32{"START", "STOP", "RESET", "RIPRENDI"})
        n106 = call "timer.vi"("Azione"=w262) -> ("f"=w271:dbl)  [unwired: 10 in]
      }
      frame 5 {
        n107 = Equal?(x=w290, y=w288) -> (x = y?=w289:bool)
        n108 = case shown="False" w289 {
          tunnel: [w292 w297] -> w283
          tunnel: w287 -> [w294 w301]
          tunnel: w286 -> [_ w295]
          frame False {
            w292 = enum32{"START", "STOP", "RESET", "RIPRENDI"}."STOP" ("Azione")
            n109 = Select(t=enum32{"START", "STOP", "RESET", "RIPRENDI"}."RESET", s=w294, f=w292) -> ()  [unwired: 1 out]
          }
          frame True {
            n110 = Select(t=enum32{"START", "STOP", "RESET", "RIPRENDI"}."START" ("Azione"), s=w301, f=enum32{"START", "STOP", "RESET", "RIPRENDI"}."STOP" ("Azione")) -> (s? t:f=w298:enum32{"START", "STOP", "RESET", "RIPRENDI"})
            n111 = Select(t=enum32{"START", "STOP", "RESET", "RIPRENDI"}."RESET", s=w295, f=w298) -> (s? t:f=w297:enum32{"START", "STOP", "RESET", "RIPRENDI"})
          }
        }
        n112 = Select(t=enum32{"START", "STOP", "RESET", "RIPRENDI"}."RESET", s=w284, f=w283) -> (s? t:f=w282:enum32{"START", "STOP", "RESET", "RIPRENDI"})
        n113 = call "timer.vi"("Azione"=w282) -> ("f"=w291:dbl)  [unwired: 10 in]
      }
      frame 6 {
        n114 = Equal?(x=w310, y=w308) -> (x = y?=w309:bool)
        n115 = case shown="False" w309 {
          tunnel: [w312 w317] -> w304
          tunnel: w307 -> [w314 w321]
          tunnel: w306 -> [_ w315]
          frame False {
            w312 = enum32{"START", "STOP", "RESET", "RIPRENDI"}."STOP" ("Azione")
            n116 = Select(t=enum32{"START", "STOP", "RESET", "RIPRENDI"}."RESET", s=w314, f=w312) -> ()  [unwired: 1 out]
          }
          frame True {
            n117 = Select(t=enum32{"START", "STOP", "RESET", "RIPRENDI"}."START" ("Azione"), s=w321, f=enum32{"START", "STOP", "RESET", "RIPRENDI"}."STOP" ("Azione")) -> (s? t:f=w318:enum32{"START", "STOP", "RESET", "RIPRENDI"})
            n118 = Select(t=enum32{"START", "STOP", "RESET", "RIPRENDI"}."RESET", s=w315, f=w318) -> (s? t:f=w317:enum32{"START", "STOP", "RESET", "RIPRENDI"})
          }
        }
        n119 = Select(t=enum32{"START", "STOP", "RESET", "RIPRENDI"}."RESET", s=w302, f=w304) -> (s? t:f=w303:enum32{"START", "STOP", "RESET", "RIPRENDI"})
        n120 = call "timer.vi"("Azione"=w303) -> ("f"=w311:dbl)  [unwired: 10 in]
      }
      frame 7 {
        n121 = Equal?(x=w330, y=w328) -> (x = y?=w329:bool)
        n122 = case shown="False" w329 {
          tunnel: [w332 w337] -> w323
          tunnel: w327 -> [w334 w341]
          tunnel: w326 -> [_ w335]
          frame False {
            w332 = enum32{"START", "STOP", "RESET", "RIPRENDI"}."STOP" ("Azione")
            n123 = Select(t=enum32{"START", "STOP", "RESET", "RIPRENDI"}."RESET", s=w334, f=w332) -> ()  [unwired: 1 out]
          }
          frame True {
            n124 = Select(t=enum32{"START", "STOP", "RESET", "RIPRENDI"}."START" ("Azione"), s=w341, f=enum32{"START", "STOP", "RESET", "RIPRENDI"}."STOP" ("Azione")) -> (s? t:f=w338:enum32{"START", "STOP", "RESET", "RIPRENDI"})
            n125 = Select(t=enum32{"START", "STOP", "RESET", "RIPRENDI"}."RESET", s=w335, f=w338) -> (s? t:f=w337:enum32{"START", "STOP", "RESET", "RIPRENDI"})
          }
        }
        n126 = Select(t=enum32{"START", "STOP", "RESET", "RIPRENDI"}."RESET", s=w324, f=w323) -> (s? t:f=w322:enum32{"START", "STOP", "RESET", "RIPRENDI"})
        n127 = call "timer.vi"("Azione"=w322) -> ("f"=w331:dbl)  [unwired: 10 in]
      }
      frame 8 {
        n128 = Equal?(x=w350, y=w348) -> (x = y?=w349:bool)
        n129 = case shown="False" w349 {
          tunnel: [w352 w357] -> w343
          tunnel: w347 -> [w354 w361]
          tunnel: w346 -> [_ w355]
          frame False {
            w352 = enum32{"START", "STOP", "RESET", "RIPRENDI"}."STOP" ("Azione")
            n130 = Select(t=enum32{"START", "STOP", "RESET", "RIPRENDI"}."RESET", s=w354, f=w352) -> ()  [unwired: 1 out]
          }
          frame True {
            n131 = Select(t=enum32{"START", "STOP", "RESET", "RIPRENDI"}."START" ("Azione"), s=w361, f=enum32{"START", "STOP", "RESET", "RIPRENDI"}."STOP" ("Azione")) -> (s? t:f=w358:enum32{"START", "STOP", "RESET", "RIPRENDI"})
            n132 = Select(t=enum32{"START", "STOP", "RESET", "RIPRENDI"}."RESET", s=w355, f=w358) -> (s? t:f=w357:enum32{"START", "STOP", "RESET", "RIPRENDI"})
          }
        }
        n133 = Select(t=enum32{"START", "STOP", "RESET", "RIPRENDI"}."RESET", s=w344, f=w343) -> (s? t:f=w342:enum32{"START", "STOP", "RESET", "RIPRENDI"})
        n134 = call "timer.vi"("Azione"=w342) -> ("f"=w351:dbl)  [unwired: 10 in]
      }
      frame 9 {
        n135 = Equal?(x=w370, y=w368) -> (x = y?=w369:bool)
        n136 = case shown="True" w369 {
          tunnel: [w372 w377] -> w363
          tunnel: w367 -> [w374 w381]
          tunnel: w366 -> [_ w375]
          frame False {
            w372 = enum32{"START", "STOP", "RESET", "RIPRENDI"}."STOP" ("Azione")
            n137 = Select(t=enum32{"START", "STOP", "RESET", "RIPRENDI"}."RESET", s=w374, f=w372) -> ()  [unwired: 1 out]
          }
          frame True {
            n138 = Select(t=enum32{"START", "STOP", "RESET", "RIPRENDI"}."START" ("Azione"), s=w381, f=enum32{"START", "STOP", "RESET", "RIPRENDI"}."STOP" ("Azione")) -> (s? t:f=w378:enum32{"START", "STOP", "RESET", "RIPRENDI"})
            n139 = Select(t=enum32{"START", "STOP", "RESET", "RIPRENDI"}."RESET", s=w375, f=w378) -> (s? t:f=w377:enum32{"START", "STOP", "RESET", "RIPRENDI"})
          }
        }
        n140 = Select(t=enum32{"START", "STOP", "RESET", "RIPRENDI"}."RESET", s=w364, f=w363) -> (s? t:f=w362:enum32{"START", "STOP", "RESET", "RIPRENDI"})
        n141 = call "timer.vi"("Azione"=w362) -> ("f"=w371:dbl)  [unwired: 10 in]
      }
    }
  }
  n142 = global write "Global compensazione attriti.vi" "compensazione attriti"(w31) -> ()
  n143 = Get Date/Time In Seconds() -> (seconds since 1Jan1904=w108:timestamp)
  n144 = Format Date/Time String(time format string (%c)="%y", seconds (now)=w108) -> (date/time string=w104:string)  [unwired: 1 in]
  n145 = Index Array(array=w55, index=w54) -> (element=w53:enum32{"START", "STOP", "RESET", "RIPRENDI"})
  n146 = Index Array(array=w91, index=w54) -> (element=w90:dbl)
  n147 = flat-sequence {
    tunnel: w49 -> [w382]
    frame #0 {
      n148 = global write "Global prova in corso.vi" "Reset tutti i timer"(w382) -> ()
    }
  }
  n149 = Number To Fractional String(number=w19, precision (6)=i16 5) -> (F-format string=w18:string)  [unwired: 2 in]
  n150 = Equal?(x=w53, y=enum32{"START", "STOP", "RESET", "RIPRENDI"}."START") -> (x = y?=w51:bool)
  n151 = global write "Global prova in corso.vi" "timer on"(w51) -> ()
  n152 = Number To Fractional String(number=w93, precision (6)=i16 5) -> (F-format string=w9:string[])  [unwired: 2 in]
  n153 = call "Tempo prova hhmmss.vi"("Tempo [s]"=w90) -> ("H:m:s"=w99:string)  [unwired: 10 in]
  n154 = Divide(x=w90, y=60.0) -> (x/y=w111:dbl)
  n155 = Number To Fractional String(number=w90, precision (6)=i16 5) -> (F-format string=w101:string)  [unwired: 2 in]
  n156 = Number To Fractional String(number=w111, precision (6)=i16 5) -> (F-format string=w102:string)  [unwired: 2 in]
  n157 = global read "Linea idraulica selezionata.vi" "Banco"() -> (w106:i32)
  n158 = Get Date/Time In Seconds() -> (seconds since 1Jan1904=w118:timestamp)
  n159 = Number To Fractional String(number=w106) -> (F-format string=w105:string)  [unwired: 3 in]
  n160 = Get Date/Time String(seconds (now)=w118, want seconds? (F)=TRUE) -> (date string=w116:string, time string=w114:string)  [unwired: 1 in]
  n161 = Concatenate Strings(w116, " " ("string"), w114) -> (w98:string)
  n162 = Index Array(array=w9) -> (element #1=w8:string, element #2=w7:string, element #3=w6:string, element #4=w5:string, element #5=w4:string, element #6=w3:string, element #7=w2:string, element #8=w1:string)  [unwired: 8 in]
  n163 = Bundle By Name(cluster=w60, "Banco"=w105, "Anno"=w104, "Numero"=w103, "Ntabella"=w103, "Misura"=w103, "Tipo Prova"=w103, "ProgressivoAcq"=w103, "Descrizione"="Descrizione", "Data_ora"=w98, "t. acq [h:m:s]"=w99, "t. acq [min]"=w102, "t. acq [s]"=w101, "Tamb[°C]"=w18, "TC1 [°C]"=w8, "TC2 [°C]"=w7, "TC3 [°C]"=w6, "TC4 [°C]"=w5, "PT1000_1[°C]"=w4, "PT1000_2[°C]"=w3, "PT1000_3[°C]"=w2, "PT1000_4[°C]"=w1) -> (w100:T28)
  n164 = case shown="True" "SIMULAZIONE" {
    tunnel: [w414 w467] -> w122
    tunnel: w100 -> [w415 w458]
    tunnel: w33 -> [w389 _]
    tunnel: w26 -> [w391 _]
    tunnel: w57 -> [w387 _]
    tunnel: "MISURE ALL" -> [_ w455]
    tunnel: "Cluster INFO" -> [w395 w420]
    tunnel: w96 -> [w393 _]
    frame False {
      # "SACCARDO disabilito, solo motori"
      # "SE COPPIA <0 TRASCINO \nALTERNATORE QUINDI REND\n= PELETTRICA(out)\\P MECC (in)"
      n165 = Unbundle By Name(w395) -> ("Dati targa motore.Vnom"=w394:dbl, "Dati targa motore.Cnom"=w392:dbl)
      n166 = Absolute Value(x=w391) -> (abs(x)=w390:dbl)
      n167 = Less Than 0?(x=w389) -> ()  [unwired: 1 out]
      n168 = Divide(x=w390, y=60.0) -> (x/y=w410:dbl)
      n169 = call "ricalcolo grandezze.vi"("^2?"=TRUE, "grandezza nom"=w392, "V"=w393, "Vn"=w394, "grandezza"=w389) -> ("grandezza ric. /nom."=w398:dbl, "grandezza ric."=w399:dbl)  [unwired: 5 in]
      n170 = Multiply(x=w410, y=6.283185307179586) -> (x*y=w412:dbl)
      n171 = Multiply(x=w412, y=w389) -> (x*y=w388:dbl)
      n172 = Divide(x=w388, y=w387) -> (x/y=w385:dbl)
      n173 = Divide(x=w387, y=w388) -> (x/y=w386:dbl)
      n174 = Select(t=w386, s=FALSE, f=w385) -> (s? t:f=w384:dbl)
      n175 = Divide(x=w388, y=1000.0) -> (x/y=w407:dbl)
      n176 = Multiply(x=w384, y=100.0) -> (x*y=w402:dbl)
      n177 = Number To Fractional String(number=w389) -> (F-format string=w413:string)  [unwired: 3 in]
      n178 = Number To Fractional String(number=w407) -> (F-format string=w405:string)  [unwired: 3 in]
      n179 = Number To Fractional String(number=w388) -> (F-format string=w408:string)  [unwired: 3 in]
      n180 = Number To Fractional String(number=w402) -> (F-format string=w401:string)  [unwired: 3 in]
      n181 = Number To Fractional String(number=w390) -> (F-format string=w404:string)  [unwired: 3 in]
      n182 = Number To Fractional String(number=w399) -> (F-format string=w397:string)  [unwired: 3 in]
      n183 = Number To Fractional String(number=w398) -> (F-format string=w396:string)  [unwired: 3 in]
      n184 = Bundle By Name(cluster=w415, "C [Nm]*C"=w413, "P2_mecc [kW]"=w405, "P2_mecc [W]"=w408, "eta motore [%]"=w401, "n [rpm]"=w404, "Cric [Nm]"=w397, "Cric\\Cnom"=w396) -> (w414:T28)
    }
    frame True {
      # "SE COPPIA <0 TRASCINO \nALTERNATORE QUINDI REND\n= PELETTRICA(out)\\P MECC (in)"
      n185 = Unbundle By Name(w455) -> ("INTERFACCIA.DI (logici).FRENO 1 run"=w444:bool, "INTERFACCIA.AO non scalati.FRENO1 rif Coppia"=w443:dbl, "INTERFACCIA.AO non scalati.FRENO1 rif vel"=w456:dbl, "INTERFACCIA.AO non scalati.FRENO2 rif Coppia"=w440:dbl, "INTERFACCIA.AO non scalati.FRENO2 rif vel"=w445:dbl, "INTERFACCIA.DI (logici).FRENO 2 run"=w438:bool)
      n186 = global read "Stato alimentatore 1.vi" "Stato alimentatore 1"() -> (w450:T45)
      n187 = global read "Stato comandi freno.vi" "Stato inverter"() -> (w457:T37)
      n188 = Unbundle By Name(w457) -> ("Stato comandi freno.Control.Control Type"=w435:T46)
      n189 = Unbundle By Name(w420) -> ("Dati targa motore.Vnom"=w422:dbl, "Dati targa motore.Cnom"=w421:dbl)
      n190 = Unbundle By Name(w450) -> ("Alimentatore 1.RIF 1"=w449:dbl, "Alimentatore 1.RIF 2"=w430:dbl)
      n191 = global read "Stato comandi freno.vi" "RPM max freno"() -> (w447:dbl)
      n192 = global read "Stato comandi freno.vi" "Cmax freno"() -> (w446:dbl)
      n193 = Absolute Value(x=w456) -> (abs(x)=w441:dbl)
      n194 = Absolute Value(x=w445) -> (abs(x)=w439:dbl)
      n195 = case shown="True" w444 {
        tunnel: w443 -> [_ w476]
        tunnel: [w471 w476] -> w442
        tunnel: w441 -> [_ w475]
        tunnel: [w469 w475] -> w437
        tunnel: w438 -> [w472 _]
        tunnel: w440 -> [w470 _]
        tunnel: w439 -> [w468 _]
        frame False {
          n196 = case shown="True" w472 {
            tunnel: [_ w474] -> w471
            tunnel: w470 -> [_ w474]
            tunnel: [_ w473] -> w469
            tunnel: w468 -> [_ w473]
            frame False {
            }
            frame True {
            }
          }
        }
        frame True {
        }
      }
      n197 = Greater Than 0?(x=w437) -> (x > 0?=w436:bool)
      n198 = Select(t=T35."Speed [RPM]", s=w436, f=w435) -> (s? t:f=w434:T46)
      n199 = Number To Fractional String(number=w430) -> (F-format string=w432:string)  [unwired: 3 in]
      n200 = Unbundle By Name(w420) -> ("Dati targa motore.Npoli"=w431:dbl)
      n201 = case shown="\"Speed [RPM]\"" w434 {
        tunnel: [w504 w538 w569 w600] -> w459
        tunnel: [w502 w536 w567 w599] -> w466
        tunnel: [w501 w535 w566 w598] -> w465
        tunnel: [w500 w534 w565 w597] -> w464
        tunnel: [w498 w532 w563 w596] -> w462
        tunnel: [w496 w530 w561 w595] -> w463
        tunnel: w437 -> [w484 _ _ _]
        tunnel: [w495 w529 w560 w594] -> w452
        tunnel: w442 -> [_ w510 w544 w591]
        tunnel: [w485 w524 w551 w592] -> w461
        tunnel: [w486 w520 w555 w593] -> w460
        tunnel: w449 -> [w477 w505 w540 w588]
        tunnel: [w480 w508 w542 w590] -> w448
        tunnel: w447 -> [w479 _ _ _]
        tunnel: w446 -> [_ w507 w541 w589]
        tunnel: [w478 w506 w539 w587] -> w417
        tunnel: [w477 w505 w540 w588] -> w416
        frame "Speed [RPM]" {
          n202 = Multiply(x=w484, y=w479) -> (x*y=w483:dbl)
          n203 = Divide(x=w483, y=100.0) -> (x/y=w481:dbl)
          n204 = call "simula cmecc.vi"("RPM"=w481, "String"="CMECC") -> ("RPM"=w494:dbl, "cosfi"=w503:dbl, "C[nm]"=w478:dbl, "I[A]"=w497:dbl, "Pin kw"=w490:dbl, "Pout kw"=w487:dbl, "eff%"=w499:dbl)  [unwired: 11 in]
          n205 = Multiply(x=w487, y=1000.0) -> (x*y=w488:dbl)
          n206 = Multiply(x=w490, y=1000.0) -> (x*y=w491:dbl)
          n207 = Number To Fractional String(number=w488) -> (F-format string=w485:string)  [unwired: 3 in]
          n208 = Number To Fractional String(number=w491) -> (F-format string=w486:string)  [unwired: 3 in]
          n209 = Number To Fractional String(number=w477) -> (F-format string=w480:string)  [unwired: 3 in]
          n210 = Number To Fractional String(number=w503) -> (F-format string=w502:string)  [unwired: 3 in]
          n211 = Number To Fractional String(number=w478) -> (F-format string=w504:string)  [unwired: 3 in]
          n212 = Number To Fractional String(number=w490) -> (F-format string=w501:string)  [unwired: 3 in]
          n213 = Number To Fractional String(number=w494) -> (F-format string=w495:string)  [unwired: 3 in]
          n214 = Number To Fractional String(number=w497) -> (F-format string=w496:string)  [unwired: 3 in]
          n215 = Number To Fractional String(number=w487) -> (F-format string=w500:string)  [unwired: 3 in]
          n216 = Number To Fractional String(number=w499) -> (F-format string=w498:string)  [unwired: 3 in]
        }
        frame "Torque [Nm]" {
          n217 = Multiply(x=w505, y=440.0) -> (x*y=w514:dbl)
          n218 = Multiply(x=w510, y=w507) -> (x*y=w511:dbl)
          n219 = Divide(x=w514, y=100.0) -> ()  [unwired: 1 out]
          n220 = Divide(x=w511, y=100.0) -> (x/y=w509:dbl)
          n221 = Equal To 0?(x=w509) -> (x = 0?=w519:bool)
          n222 = Select(t="VUOTO", s=w519, f="CARICO" ("String")) -> (s? t:f=w517:string)
          n223 = call "simula cmecc.vi"("C"=w509, "String"=w517, "V"=w505) -> ("RPM"=w528:dbl, "cosfi"=w537:dbl, "C[nm]"=w506:dbl, "I[A]"=w531:dbl, "Pin kw"=w522:dbl, "Pout kw"=w527:dbl, "eff%"=w533:dbl)  [unwired: 10 in]
          n224 = Multiply(x=w522, y=1000.0) -> (x*y=w521:dbl)
          n225 = Multiply(x=w527, y=1000.0) -> (x*y=w525:dbl)
          n226 = Number To Fractional String(number=w521) -> (F-format string=w520:string)  [unwired: 3 in]
          n227 = Number To Fractional String(number=w505) -> (F-format string=w508:string)  [unwired: 3 in]
          n228 = Number To Fractional String(number=w537) -> (F-format string=w536:string)  [unwired: 3 in]
          n229 = Number To Fractional String(number=w506) -> (F-format string=w538:string)  [unwired: 3 in]
          n230 = Number To Fractional String(number=w522) -> (F-format string=w535:string)  [unwired: 3 in]
          n231 = Number To Fractional String(number=w528) -> (F-format string=w529:string)  [unwired: 3 in]
          n232 = Number To Fractional String(number=w531) -> (F-format string=w530:string)  [unwired: 3 in]
          n233 = Number To Fractional String(number=w527) -> (F-format string=w534:string)  [unwired: 3 in]
          n234 = Number To Fractional String(number=w525) -> (F-format string=w524:string)  [unwired: 3 in]
          n235 = Number To Fractional String(number=w533) -> (F-format string=w532:string)  [unwired: 3 in]
        }
        frame "Power [W]" {
          n236 = Multiply(x=w544, y=w541) -> (x*y=w545:dbl)
          n237 = Equal To 0?(x=w544) -> (x = 0?=w550:bool)
          n238 = Divide(x=w545, y=100.0) -> (x/y=w543:dbl)
          n239 = Select(t="VUOTO", s=w550, f="CARICO" ("String")) -> (s? t:f=w547:string)
          n240 = call "simula cmecc.vi"("C"=w543, "String"=w547, "V"=w540) -> ("RPM"=w559:dbl, "cosfi"=w568:dbl, "C[nm]"=w539:dbl, "I[A]"=w562:dbl, "Pin kw"=w556:dbl, "Pout kw"=w552:dbl, "eff%"=w564:dbl)  [unwired: 10 in]
          n241 = Multiply(x=w556, y=1000.0) -> (x*y=w557:dbl)
          n242 = Multiply(x=w552, y=1000.0) -> (x*y=w553:dbl)
          n243 = Number To Fractional String(number=w557) -> (F-format string=w555:string)  [unwired: 3 in]
          n244 = Number To Fractional String(number=w553) -> (F-format string=w551:string)  [unwired: 3 in]
          n245 = Number To Fractional String(number=w540) -> (F-format string=w542:string)  [unwired: 3 in]
          n246 = Number To Fractional String(number=w568) -> (F-format string=w567:string)  [unwired: 3 in]
          n247 = Number To Fractional String(number=w539) -> (F-format string=w569:string)  [unwired: 3 in]
          n248 = Number To Fractional String(number=w556) -> (F-format string=w566:string)  [unwired: 3 in]
          n249 = Number To Fractional String(number=w559) -> (F-format string=w560:string)  [unwired: 3 in]
          n250 = Number To Fractional String(number=w562) -> (F-format string=w561:string)  [unwired: 3 in]
          n251 = Number To Fractional String(number=w564) -> (F-format string=w563:string)  [unwired: 3 in]
          n252 = Number To Fractional String(number=w552) -> (F-format string=w565:string)  [unwired: 3 in]
        }
        frame "Corrente [A]" {
          n253 = Multiply(x=w591, y=w589) -> (x*y=w571:dbl)
          n254 = Equal To 0?(x=w591) -> (x = 0?=w576:bool)
          n255 = Divide(x=w571, y=100.0) -> (x/y=w570:dbl)
          n256 = Select(t="VUOTO", s=w576, f="CARICO" ("String")) -> (s? t:f=w573:string)
          n257 = call "simula cmecc.vi"("C"=w570, "String"=w573, "V"=w588) -> ("RPM"=w583:dbl, "cosfi"=w586:dbl, "C[nm]"=w587:dbl, "I[A]"=w584:dbl, "Pin kw"=w580:dbl, "Pout kw"=w577:dbl, "eff%"=w585:dbl)  [unwired: 10 in]
          n258 = Multiply(x=w580, y=1000.0) -> (x*y=w581:dbl)
          n259 = Multiply(x=w577, y=1000.0) -> (x*y=w578:dbl)
          n260 = Number To Fractional String(number=w581) -> (F-format string=w593:string)  [unwired: 3 in]
          n261 = Number To Fractional String(number=w578) -> (F-format string=w592:string)  [unwired: 3 in]
          n262 = Number To Fractional String(number=w588) -> (F-format string=w590:string)  [unwired: 3 in]
          n263 = Number To Fractional String(number=w586) -> (F-format string=w599:string)  [unwired: 3 in]
          n264 = Number To Fractional String(number=w587) -> (F-format string=w600:string)  [unwired: 3 in]
          n265 = Number To Fractional String(number=w580) -> (F-format string=w598:string)  [unwired: 3 in]
          n266 = Number To Fractional String(number=w583) -> (F-format string=w594:string)  [unwired: 3 in]
          n267 = Number To Fractional String(number=w584) -> (F-format string=w595:string)  [unwired: 3 in]
          n268 = Number To Fractional String(number=w585) -> (F-format string=w596:string)  [unwired: 3 in]
          n269 = Number To Fractional String(number=w577) -> (F-format string=w597:string)  [unwired: 3 in]
        }
      }
      n270 = call "ricalcolo grandezze.vi"("^2?"=TRUE, "grandezza nom"=w421, "V"=w416, "Vn"=w422, "grandezza"=w417) -> ("grandezza ric. /nom."=w423:dbl, "grandezza ric."=w424:dbl)  [unwired: 5 in]
      n271 = global read "Stato alimentatore 1.vi" "Stato alimentatore 1"() -> (w453:T45)
      n272 = Number To Fractional String(number=w424) -> (F-format string=w419:string)  [unwired: 3 in]
      n273 = Number To Fractional String(number=w423) -> (F-format string=w418:string)  [unwired: 3 in]
      n274 = Unbundle By Name(w453) -> ("In marcia"=w454:bool)
      n275 = Select(t=w452, s=w454, f="0") -> (s? t:f=w429:string)
      n276 = Fract/Exp String To Number(string=w429) -> (number=w428:dbl)  [unwired: 3 in, 1 out]
      n277 = call "Calcolo SCORRIMENTO.vi"("POLI"=w431, "FREQ"=w430, "RPM"=w428) -> ("SCORRIMENTO"=w427:dbl)  [unwired: 8 in]
      n278 = Number To Fractional String(number=w427) -> (F-format string=w426:string)  [unwired: 3 in]
      n279 = Bundle By Name(cluster=w458, "C [Nm]*C"=w459, "pf"=w466, "P1 [kW]"=w465, "P1 [W]"=w460, "P2_mecc [kW]"=w464, "P2_mecc [W]"=w461, "eta motore [%]"=w462, "I1[A]"=w463, "I2[A]"=w463, "I3[A]"=w463, "I123_media [A]*I"=w463, "n [rpm]"=w429, "U123_media [V]"=w448, "U1[V]"=w448, "U2 [V]"=w448, "U3 [V]"=w448, "f [Hz]"=w432, "Scorr[%]"=w426, "Cric [Nm]"=w419, "Cric\\Cnom"=w418) -> (w467:T28)
    }
  }
  n280 = Bundle By Name(cluster=w123, "MISURE NM"=w122, "MISURE ALL"="MISURE ALL") -> (→"Cluster MISURE":T27)
